vi "Labview_Mqtt_Toolkit.vi"() -> ()   [LabVIEW 2021]
uses:
  class/mqtt/mqttTypedef/mqttQOSlevel.ctl
  class/mqtt/mqttTypedef/mqttConnectionStatus.ctl
  class/mqtt/mqttTypedef/mqttBroker.ctl
  class/mqtt/mqttTXqueue/mqttTXdataQueueFunction.ctl
  class/mqtt/mqttConfigFunction.ctl
  class/mqtt/mqttTXqueue/mqttRXsubscriptionEventFunction.ctl
  class/mqtt/mqttTypedef/mqttConnectionFlags.ctl
  <vilib>/Utility/sysdir.llb/System Directory Type.ctl
  library/Epoch Date & Time/epoch.UNIX/Epoch.UNIX.lvclass
  C:/Users/Fujitsu/Desktop/Nouveau dossier/avril/Project mqtt/Src/library/Epoch Date & Time/epoch/Epoch.lvclass
  <vilib>/Utility/file.llb/Write Delimited Spreadsheet (string).vi
  library/Epoch Date & Time/Get Epoch Time.vi
  class/mqtt/mqtt.lvclass
panel:
  out "concatenated string":string
  in  "Tab Control":T1(tab)
  out "Connection Success":bool
  in  "connect":bool
  out "ConnStatus":T2
  in  "disconnect":bool
  in  "subscribe":bool
  out "Subscribe Success":bool
  out "subscribeMessageID":u16 format="%02x"
  in  "Subscription_Info":cluster{"Topic":string, "QoS":T3}[](array[cluster])=[{"Topic"="MacID/Topic", "QoS"=enum."At most once"}]
  out "Subscribed_Topic":string
  out "messageID":u16
  in  "quit":bool
  in  "Broker configuration":T4={"IP or  URL of the broker"="", "connTimeout"=2000, "writeTimeout"=2000, "readTimeout"=2000, "subTimeout"=30000, "port"=1883}
  out "Measure Graph":dbl(graph)
  out "Measure Mode":string
  out "Sensor Label":string
  out "Measure":dbl
  out "Date & time":string
  out "Device type":string
  out "End Date":string
  out "Start Date":string
  out "Average value":dbl
  out "Minimum value":dbl
  out "Maximum value":dbl
  out "Date":string
  out "Date":string
  out "File path":path
  out "File path":path
  out "Measure Mode":string
  out "Sensor Label":string
  out "Measure":dbl
  out "Date & time":string
  out "Device type":string
  out "Alarm status":string
  out "Waveform Chart":dbl(graph) caption="Measure Graph"
  out "File path 3":path
  out "Sampling rate":i16
  out "Frame sequence Id":u32
  out "Number of daq per channel":u16
  out "Data acquisition cycle":u32
  out "Data acquisition duration":u32
  out "Prev.Number of daq per channel":u16
  out "Enabled channels":string
  out "Device Type":string
  out "Measure Mode":string
  out "millisec":u16
  out "not synchronised":bool
  out "synchronised":bool
  out "Network Quality (LQI)":u8 format="%.0p"
  out "Time Ref":string
  out "INC_Y Graph":dbl[](graph)
  out "CH_Z Graph":dbl[](graph)
  out "CH_X Graph":dbl[](graph)
  out "CH_Y Graph":dbl[](graph)
  out "INC_X Graph":dbl[](graph)
  out "File path":path
  out "Enabled channels":string
  out "Device Type":string
  out "Measure Mode":string
  out "Frame sequence Id":u32
  out "Number of daq per channel":u16
  out "Data Notification cycle":u32
  out "Data acquisition duration":u32
  out "Prev.Number of daq per channel":u16
  out "not synchronised":bool
  out "synchronised":bool
  out "Network Quality (LQI)":u8 format="%.0p"
  out "Sampling rate":i16
  out "millisec":u16
  out "Time Ref":string
  out "channel that received alarm":u8
  out "CH_Z Graph":dbl[](graph)=[0.984, 0.974, 0.974, 0.986, 1.009, 0.965, 0.949, 0.987, 0.909, 0.979, 0.976, 1.021, 0.92, 0.95, 1.042, 0.989, 0.939, 1.09, 0.874, 0.972, 0.98, 0.977, 0.963, 0.971, 0.982, 0.977, 0.992, 0.993, 0.98, 0.969, 0.975, 0.969, 0.986, 0.985, 0.978, 0.977, 0.982, 0.979, 0.977, 0.972, 0.967, 0.968, 0.986, 0.97, 0.973, 0.977, 0.982, 0.973, 0.953, 0.969, 0.983, 0.968, 0.965, 0.975, 0.974, 0.972, 0.983, 0.99, 0.968, 0.972, 0.97, 0.981, 0.968, 0.982, 0.979, 0.972]
  out "CH_X Graph":dbl[](graph)=[0.011, 0.001, 0.002, 0.005, 0.007, 0.003, 0.001, 0.011, -0.001, 0.008, 0.006, 0.001, -0.001, 0.017, -0.002, 0.004, 0.0, -0.007, 0.002, -0.007, 0.001, 0.002, 0.0, 0.003, 0.004, 0.009, 0.004, 0.012, 0.003, 0.003, 0.004, 0.003, 0.006, 0.001, -0.001, 0.003, 0.002, 0.001, 0.003, 0.0, -0.001, 0.005, 0.0, 0.005, 0.001, 0.005, 0.005, -0.001, -0.002, -0.001, 0.005, 0.003, -0.003, -0.003, 0.002, -0.002, 0.002, 0.007, 0.0, 0.0, -0.002, 0.001, 0.002, 0.005, 0.011, 0.006]
  out "CH_Y Graph":dbl[](graph)=[-0.006, -0.012, -0.012, -0.009, -0.015, 0.009, 0.007, -0.013, 0.026, 0.009, -0.014, -0.014, 0.046, 0.055, -0.014, 0.004, 0.027, -0.027, 0.076, -0.008, -0.016, -0.026, -0.02, -0.015, -0.01, -0.002, -0.005, -0.011, -0.019, -0.019, -0.014, -0.009, -0.01, -0.01, -0.017, -0.015, -0.01, -0.013, -0.014, -0.014, -0.014, -0.014, -0.013, -0.017, -0.015, -0.013, -0.008, -0.015, -0.02, -0.017, -0.011, -0.014, -0.015, -0.016, -0.019, -0.016, -0.016, -0.012, -0.016, -0.016, -0.01, -0.013, -0.013, -0.019, -0.015, -0.012]
  out "INC_X Graph":dbl[](graph)=[0.03, 0.047, 0.036, 0.04, 0.082, 0.015, 0.021, 0.002, -0.032, 0.039, 0.026, 0.014, 0.037, 0.052, 0.099, 0.049, 0.039, 0.13, -0.382, 0.13, 0.113, 0.024, 0.006, -0.008, 0.051, 0.01, 0.082, 0.011, 0.03, 0.0, 0.031, 0.032, 0.033, 0.046, 0.032, 0.037, 0.018, 0.028, 0.024, 0.031, -0.008, 0.054, 0.011, 0.025, 0.04, 0.026, 0.022, 0.017, 0.028, 0.042, 0.024, 0.016, 0.034, 0.035, 0.018, 0.043, 0.014, 0.039, 0.033, 0.018, 0.035, 0.027, 0.041, 0.031, 0.035, 0.03]
  out "INC_Y Graph":dbl[](graph)=[0.458, 0.458, 0.458, 0.458, 0.458, 0.458, 0.458, 0.458, 0.458, 0.458, 0.458, 0.458, 0.458, 0.458, 0.458, 0.458, 0.458, 0.458, 0.458, 0.458, 0.458, 0.458, 0.458, 0.458, 0.458, 0.458, 0.458, 0.458, 0.458, 0.458, 0.458, 0.458, 0.458, 0.458, 0.458, 0.458, 0.458, 0.458, 0.458, 0.458, 0.458, 0.458, 0.458, 0.458, 0.458, 0.458, 0.458, 0.458, 0.458, 0.458, 0.458, 0.458, 0.458, 0.458, 0.458, 0.458, 0.458, 0.458, 0.458, 0.458, 0.458, 0.458, 0.458, 0.458, 0.458, 0.458]
  out "File path":path
  out "Device type":string
  out "Acquisition Mode":string
  out "Acquisition frequency":u16
  out "Acquisition cycle":u32
  out "Acquisition duration":u32
  out "Enabled channels":string
  out "Start date":string
  out "End date":string
  out "Number of data per channel":u16
  out "fid min ch1":u32
  out "index minval":u16
  out "fid max ch1":u32
  out "index maxval":u16
  out "Max value":dbl[](array[numeric])
  out "Average value":dbl[](array[numeric])
  out "Min value":dbl[](array[numeric])
  out "String":string="Ch_Z                    Ch_X                     Ch_Y                     INC_X                     INC_Y"
  out "File path":path
  out "Min date":string[](array[string])
  out "Max date":string[](array[string])
  out "Numeric":i32
  # "LowDutyCycle Measurement"
  # "MathMode Result"
  # "AlarmMode Data"
types:
  T1 = enum32{"Configuration", "LowDutyCycleData", "AlarmData ", "StreamingModeData", "S.E.T Mode", "Dynamic Math Result"}
  T2 = typedef "mqttConnectionStatus.ctl" = enum16{"Connection accepted", "Connection refused: unacceptable protocol version", "Connection refused: identifier rejected", "Connection refused: Server unavailable", "Connection refused: bad user name or password", "Connection refused: not authorized"}
  T3 = typedef "mqttQOSlevel.ctl" = enum8{"At most once", "At least once", "Exactly once", "Reserved"}
  T4 = typedef "mqttBroker.ctl" = cluster{"IP or  URL of the broker":string, "connTimeout":i32, "writeTimeout":i32, "readTimeout":i32, "subTimeout":i32, "port":u16}
  T5 = typedef "mqttConnectionFlags.ctl" = cluster{"reserved":bool, "clean session":bool, "will flag":bool, "willQOS":enum8{"At most once", "At least once", "Exactly once", "Reserved"}, "will retain":bool, "password":bool, "user name":bool}
  T6 = typedef "mqttRXsubscriptionEventFunction.ctl" = enum16{"init", "deinit", "getEventRef", "event"}
  T7 = typedef "mqtt.lvclass/mqttConfigFunction.ctl" = enum16{"init", "deinit", "set", "get"}
  T8 = typedef "mqttTXdataQueueFunction.ctl" = enum16{"init", "deinit", "getQueue", "enqueue"}
  T9 = enum8{"Enabled", "Disabled", "Disabled and Grayed Out"}
  T10 = enum16{"open", "replace", "create", "open or create", "replace or create", "replace or create with confirmation"}
  T11 = cluster{"[0]":u8, "[1]":u8, "[2]":u8, "[3]":u8, "[4]":u8, "[5]":u8, "[6]":u8, "[7]":u8, "[8]":u8}
  T12 = cluster{"[0]":u8, "[1]":u8, "[2]":u8, "[3]":u8, "[4]":u8, "[5]":u8, "[6]":u8, "[7]":u8, "[8]":u8, "[9]":u8, "[10]":u8, "[11]":u8, "[12]":u8}
  T13 = typedef "System Directory Type.ctl" = i32
  T14 = cluster{"unsigned byte array[0]":u8, "unsigned byte array[1]":u8}
  T15 = cluster{"[0]":u8, "[1]":u8, "[2]":u8, "[3]":u8, "[4]":u8, "[5]":u8, "[6]":u8, "[7]":u8, "[8]":u8, "[9]":u8, "[10]":u8, "[11]":u8, "[12]":u8, "[13]":u8, "[14]":u8, "[15]":u8}
  T16 = cluster{"unsigned byte array[0]":u8, "unsigned byte array[1]":u8, "unsigned byte array[2]":u8, "unsigned byte array[3]":u8, "unsigned byte array[4]":u8, "unsigned byte array[5]":u8, "unsigned byte array[6]":u8, "unsigned byte array[7]":u8, "unsigned byte array[8]":u8, "unsigned byte array[9]":u8, "unsigned byte array[10]":u8, "unsigned byte array[11]":u8, "unsigned byte array[12]":u8, "unsigned byte array[13]":u8, "unsigned byte array[14]":u8, "unsigned byte array[15]":u8, "unsigned byte array[16]":u8, "unsigned byte array[17]":u8, "unsigned byte array[18]":u8, "unsigned byte array[19]":u8, "unsigned byte array[20]":u8, "unsigned byte array[21]":u8, "unsigned byte array[22]":u8, "unsigned byte array[23]":u8, "unsigned byte array[24]":u8, "unsigned byte array[25]":u8, "unsigned byte array[26]":u8, "unsigned byte array[27]":u8, "unsigned byte array[28]":u8, "unsigned byte array[29]":u8, "unsigned byte array[30]":u8, "unsigned byte array[31]":u8, "unsigned byte array[32]":u8, "unsigned byte array[33]":u8, "unsigned byte array[34]":u8, "unsigned byte array[35]":u8}
  T17 = cluster{"[0]":string, "[1]":string, "[2]":string, "[3]":string, "[4]":string}
  T18 = cluster{"[0]":dbl, "[1]":dbl, "[2]":dbl, "[3]":dbl, "[4]":dbl}
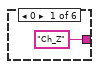
[diagram p7: hidden frame]
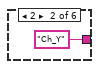
[diagram p8: hidden frame]
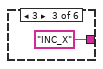
[diagram p9: hidden frame]
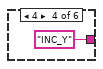
[diagram p10: hidden frame]
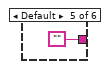
[diagram p11: hidden frame]
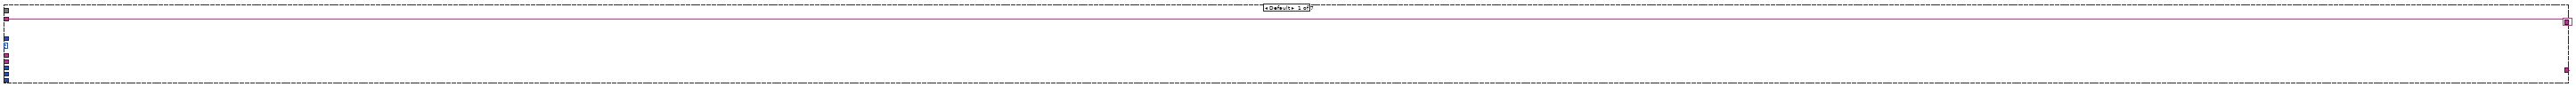
[diagram p12: hidden frame]
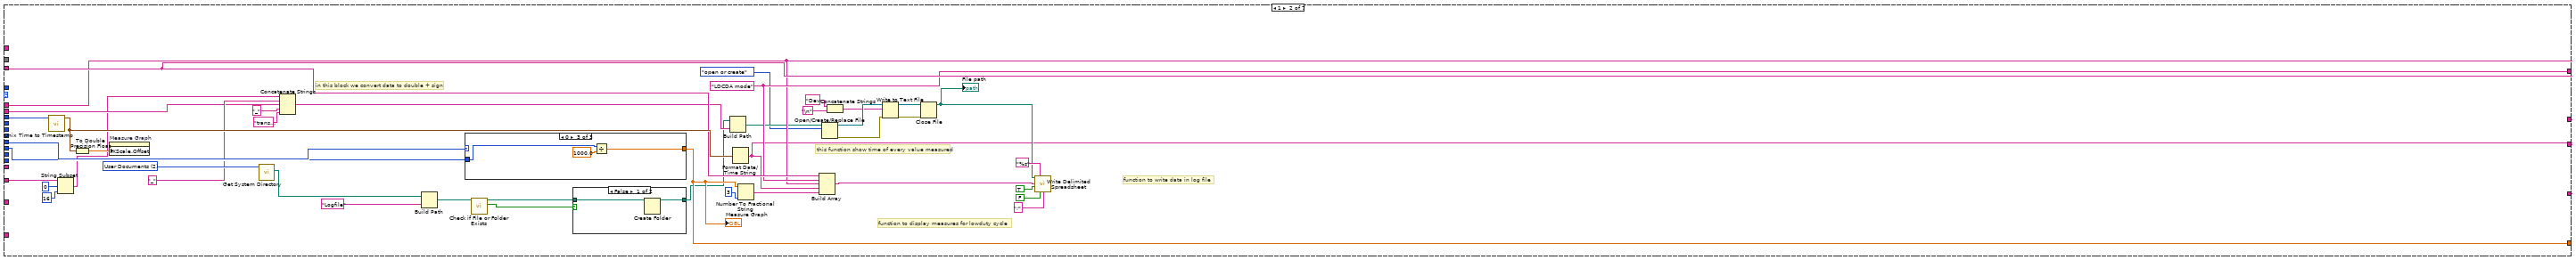
[diagram p13: hidden frame]
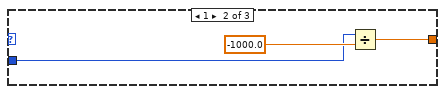
[diagram p16: hidden frame]
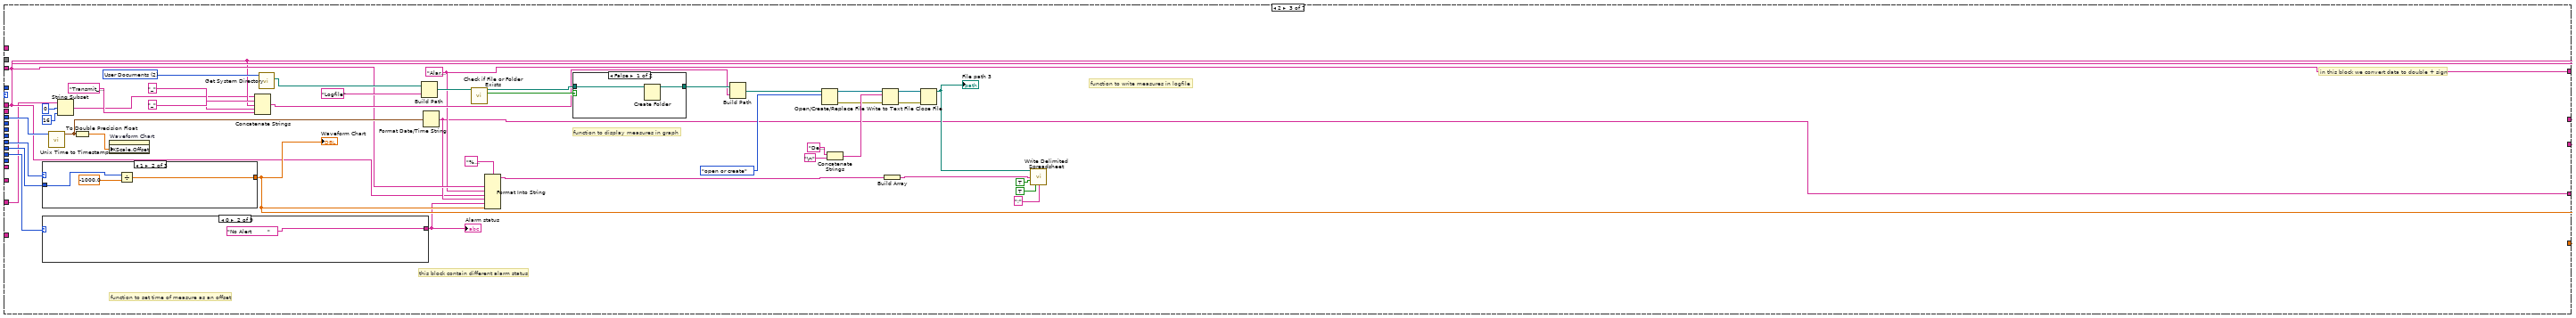
[diagram p17: hidden frame]
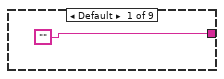
[diagram p18: hidden frame]
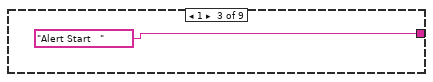
[diagram p19: hidden frame]
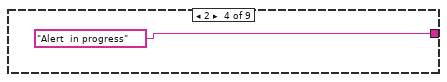
[diagram p20: hidden frame]
diagram:
  w6 = T5 {"reserved"=FALSE, "clean session"=TRUE, "will flag"=TRUE, "willQOS"=enum."At most once", "will retain"=FALSE, "password"=FALSE, "user name"=FALSE}  # connFlags
  # "used to reinitialize to default  data when you execute VI"
  # "cluster contain connection flags"
  # "cluster contain broker configuration"
  # "you will find the subscriptionData in event number 4 by click on this arrow"
  n1 = flat-sequence {
    tunnel: [w25] -> w19
    tunnel: [w22] -> w13
    frame #0 {
      w21 = T9."Disabled and Grayed Out" ("Disabled")
      n2 = property on="disconnect" class="Bool"("DisabledEnum"=w21) -> ()  [unwired: 2 in, 2 out]
      n3 = property on="subscribe" class="Bool"("DisabledEnum"=w21) -> ()  [unwired: 2 in, 2 out]
      n4 = call "mqttRXsubscriptionEvent.vi"("function"=mqttRXsubscriptionEventFunction."init") -> ("subscriptionData"=w22:refnum<user-event>, "error out"=w24:errorcluster)  [unwired: 13 in]
      n5 = call "mqttTXdataQueue.vi"("function"=mqttTXdataQueueFunction."init", "error in (no error)"=w24) -> ("error out"=w25:errorcluster)  [unwired: 12 in, 1 out]
    }
  }
  n6 = control-ref of="This VI"() -> (w5:refnum<vi>)
  n7 = invoke class="VI" method="Default Vals.Reinit All"(reference=w5) -> (reference out=w3:refnum<vi>, error out=w4:errorcluster)  [unwired: 2 in, 1 out]
  n8 = call "api_mqttInit.vi"("broker"="Broker configuration", "connFlags"=w6, "error in (no error)"=w19) -> ("error out"=w17:errorcluster)  [unwired: 12 in]
  n9 = register-events(w13) -> (reference out=w12:refnum<event-registration>)  [unwired: 2 in, 1 out]
  n10 = call "mqttConfigStore.vi"("function"=mqttConfigFunction."get", "error in (no error)"=w17) -> ("mqtt.lvclass out"=w16:refnum<class "mqtt.lvclass">, "error out"=w15:errorcluster)  [unwired: 12 in]
  n11 = call "mqttTCPIPserver.vi"("mqtt.lvclass"=w16, "error in (no error)"=w15) -> ()  [unwired: 12 in, 2 out]
  n12 = Close Reference(reference=w3, error in (no error)=w4) -> (error out=w2:errorcluster)
  n13 = while {
    shift-right: [w32] -> w9
    shift-left: w15 -> [w27]
    tunnel: w12 -> [w31]
    tunnel: [w30] -> w7
    tunnel: w2 -> [_]
    i -> [w28]
    stop <- w29 stop-if-true
    n14 = event shown="[4] <subscriptionData>: User Event" {
      selector: w31 -> [_ _ _ _ _]
      dyn-events: [_ _ _ _ _] -> w30
      timeout: _ -> [_ _ _ _ _]
      tunnel: [w33 w37 w40 w44 w129] -> w32
      tunnel: w27 -> [w33 w38 w41 w42 w129]
      tunnel: [TRUE _ _ _ _] -> w29
      tunnel: w28 -> [_ _ _ _ w50]
      event "quit": Value Change {
        # "when we press quit in front panel the process is stopped"
        n15 = event-data() -> ()  [unwired: 1 in, 1 out]
      }
      event "connect": Value Change {
        n16 = event-data() -> ()  [unwired: 1 in, 4 out]
        n17 = call "api_mqttConnect.vi"("error in (no error)"=w38) -> ("success"=→"Connection Success":bool, "connStatus"=w36:T2, "error out"=w37:errorcluster)  [unwired: 11 in, 1 out]
        "ConnStatus" <- w36
        n18 = case shown="\"Connection accepted\"" w36 {
          frame "Connection accepted" {
            w39 = T9."Enabled" ("Disabled")
            n19 = property on="subscribe" class="Bool"("DisabledEnum"=w39) -> ()  [unwired: 2 in, 2 out]
            n20 = property on="disconnect" class="Bool"("DisabledEnum"=w39) -> ()  [unwired: 2 in, 2 out]
          }
          frame Default {
          }
        }
      }
      event "disconnect": Value Change {
        n21 = event-data() -> ()  [unwired: 1 in, 4 out]
        n22 = call "api_mqttDisconnect.vi"("error in (no error)"=w41) -> ("error out"=w40:errorcluster)  [unwired: 13 in, 1 out]
      }
      event "subscribe": Value Change {
        # "this indicator turn to green when the subscription sucssed"
        n23 = event-data() -> ()  [unwired: 1 in, 4 out]
        n24 = feedback #1(u16 0) -> (w47:u16)
        n25 = Increment(x=w47) -> (x+1=w43:u16)
        "subscribeMessageID" <- w43
        n26 = feedback-in #1(w43) -> ()
        n27 = call "api_mqttSubscribe.vi"("subscriptionInfo"="Subscription_Info", "messageID"=w43, "error in (no error)"=w42) -> ("success"=→"Subscribe Success":bool, "error out"=w44:errorcluster)  [unwired: 11 in]
      }
      event User Event {
        # "here you will find different modes of  data acquisition"
        n28 = event-data() -> ("topic"=w49:string, "value"=w63:string, "messageID"=→"messageID":u16)  [unwired: 1 in]
        "Subscribed_Topic" <- w49
        n29 = String To Byte Array(string=w63) -> (unsigned byte array=w71:u8[])
        n30 = Reverse 1D Array(array=w71) -> (reversed array=w115:u8[])
        n31 = Array Subset(array=w115, index=0, length=3) -> (w54:u8[])
        n32 = Array Subset(array=w71, index=0, length=7) -> (w66:u8[])
        n33 = Array Subset(array=w71, index=7, length=1) -> (w73:u8[])
        n34 = Array To Cluster(array=w73) -> (cluster=w72:cluster{"[0]":u8})
        n35 = Array To Cluster(array=w66) -> (cluster=w121:T11)
        n36 = Array Subset(array=w71, index=3, length=13) -> (w108:u8[])
        n37 = Unbundle By Name(w72) -> ("[0]"=w52:u8)
        n38 = Unbundle By Name(w121) -> ("[0]"=w53:u8, "[1]"=w79:u8, "[2]"=w116:u8, "[3]"=w120:u8, "[4]"=w119:u8, "[5]"=w118:u8, "[6]"=w117:u8)
        n39 = Array To Cluster(array=w108) -> (cluster=w107:T12)
        n40 = Array To Cluster(array=w54) -> (cluster=w61:cluster{"[0]":u8, "[1]":u8, "[2]":u8})
        n41 = Unbundle By Name(w107) -> ("[0]"=w64:u8, "[1]"=w87:u8, "[2]"=w86:u8, "[3]"=w85:u8, "[4]"=w84:u8, "[5]"=w91:u8, "[6]"=w90:u8, "[7]"=w89:u8, "[8]"=w88:u8, "[9]"=w81:u8, "[10]"=w80:u8, "[11]"=w83:u8, "[12]"=w82:u8)
        n42 = Join Numbers(hi=w117, lo=w118) -> ((hi.lo)=w112:u16)
        n43 = Join Numbers(hi=w119, lo=w120) -> ((hi.lo)=w111:u16)
        n44 = Unbundle(w61) -> ("[0]"=w58:u8, "[1]"=w59:u8, "[2]"=w60:u8)
        n45 = case shown="6" w53 {
          tunnel: ["AX-3D" "HI_INC_MONO" "HI_INC_BI" "X_INC_MONO " "X _INC_BI " "AX_3DS" ""] -> w62
          frame 1 {
          }
          frame 2 {
          }
          frame 3 {
          }
          frame 4 {
          }
          frame 5 {
          }
          frame 6 {
          }
          frame Default {
          }
        }
        "Device type" <- w62
        n46 = case shown="1" w116 {
          tunnel: ["Ch_Z" "Ch_Y" "INC_X" "INC_Y" "" "Ch_X"] -> w51
          frame 0 {
          }
          frame 2 {
          }
          frame 3 {
          }
          frame 4 {
          }
          frame Default {
          }
          frame 1 {
          }
        }
        n47 = Join Numbers(hi=w59, lo=w60) -> ((hi.lo)=w56:u16)
        n48 = Join Numbers(hi=w84, lo=w85) -> ((hi.lo)=w103:u16)
        n49 = Join Numbers(hi=w86, lo=w87) -> ((hi.lo)=w102:u16)
        n50 = Join Numbers(hi=w88, lo=w89) -> ((hi.lo)=w98:u16)
        n51 = Join Numbers(hi=w90, lo=w91) -> ((hi.lo)=w97:u16)
        n52 = Join Numbers(hi=w82, lo=w83) -> ((hi.lo)=w93:u16)
        n53 = Join Numbers(hi=w80, lo=w81) -> ((hi.lo)=w92:u16)
        n54 = To Unsigned Word Integer(number=w112) -> (unsigned 16bit integer=w125:u16)
        n55 = To Unsigned Word Integer(number=w111) -> (unsigned 16bit integer=w124:u16)
        n56 = To Word Integer(number=w58) -> (16bit integer=w127:i16)
        n57 = Sign(1:w127) -> (0:w57:i16)
        n58 = Join Numbers(hi=w125, lo=w124) -> ((hi.lo)=w126:u32)
        n59 = To Unsigned Word Integer(number=w103) -> (unsigned 16bit integer=w105:u16)
        n60 = To Unsigned Word Integer(number=w102) -> (unsigned 16bit integer=w104:u16)
        n61 = To Unsigned Word Integer(number=w98) -> (unsigned 16bit integer=w100:u16)
        n62 = To Unsigned Word Integer(number=w97) -> (unsigned 16bit integer=w99:u16)
        n63 = To Unsigned Word Integer(number=w93) -> (unsigned 16bit integer=w95:u16)
        n64 = To Unsigned Word Integer(number=w92) -> (unsigned 16bit integer=w94:u16)
        n65 = Join Numbers(hi=w105, lo=w104) -> ((hi.lo)=w106:u32)
        n66 = Join Numbers(hi=w100, lo=w99) -> ((hi.lo)=w101:u32)
        n67 = Join Numbers(hi=w95, lo=w94) -> ((hi.lo)=w96:u32)
        n68 = To Unsigned Long Integer(number=w126) -> (unsigned 32bit integer=w78:u32)
        n69 = To Unsigned Long Integer(number=w106) -> (unsigned 32bit integer=w75:u32)
        n70 = To Unsigned Long Integer(number=w101) -> (unsigned 32bit integer=w76:u32)
        n71 = To Unsigned Long Integer(number=w96) -> (unsigned 32bit integer=w77:u32)
        n72 = case shown="3" w79 {
          tunnel: ["" w172 w206 "Streaming mode" "LDC Math Result" "S.E.T mode " "Dynamic Math Result"] -> w70
          tunnel: w78 -> [_ w178 w232 _ _ _ _]
          tunnel: [_ w146 w198 _ "" _ _] -> w65
          tunnel: w62 -> [w136 w174 w207 w406 w2481 w2648 w4843]
          tunnel: [w136 w174 w207 w406 w2481 w2648 w4843] -> w69
          tunnel: w51 -> [_ w171 w196 w405 w2479 _ w4842]
          tunnel: [_ w171 w196 w405 w2479 _ w4842] -> w68
          tunnel: w57 -> [_ w180 w230 _ w2475 _ _]
          tunnel: w56 -> [_ w179 w231 _ w2477 _ _]
          tunnel: [_ w175 w205 _ _ _ _] -> w55
          tunnel: w64 -> [_ _ _ _ w2476 _ _]
          tunnel: w77 -> [_ _ _ _ w2478 _ _]
          tunnel: w76 -> [_ _ _ _ w2433 _ _]
          tunnel: w75 -> [_ _ _ _ w2434 _ _]
          tunnel: w63 -> [_ _ _ w352 _ w2637 w4840]
          tunnel: w62 -> [_ _ _ _ _ _ w4841]
          tunnel: w54 -> [_ _ _ _ _ _ _]
          tunnel: w49 -> [_ _ _ w255 w2439 _ _]
          tunnel: w49 -> [_ _ w191 _ _ w2503 w4683]
          tunnel: w49 -> [_ w141 _ _ _ _ _]
          tunnel: w53 -> [_ _ _ _ _ _ w4721]
          tunnel: w52 -> [_ _ w200 _ _ _ _]
          tunnel: w51 -> [_ w144 _ _ w2444 _ _]
          frame Default {
          }
          frame 1 {
            w152 = T13 2 items=["User Home"=0, "User Desktop"=1, "User Documents"=2, "User Application Data"=3, "User Preferences"=4, "User Temporary"=5, "Public Documents"=6, "Public Application Data"=7, "Public Preferences"=8, "Public Cache"=13, "System Core Libraries"=9, "System Installed Libraries"=10, "Application Files"=11, "Boot Volume Root"=12] ("system directory type")
            w172 = "LDCDA mode"
            # "this function show time of every value measured"
            # "function to display measures for lowduty cycle"
            # "function to write data in log file"
            # "in this block we convert data to double + sign"
            n73 = call "Unix Time to Timestamp.vi"("Unix Time (s)"=w178) -> ("Timestamp"=w177:timestamp)  [unwired: 9 in, 1 out]
            n74 = String Subset(string=w141, offset (0)=0, length (rest)=16 ("length (rest)")) -> (substring=w138:string)
            n75 = To Double Precision Float(number=w177) -> (double precision float=w165:dbl)
            n76 = property on="Measure Graph" class="WFChart (strict)"("XScale.Offset"=w165) -> ()  [unwired: 2 in, 2 out]
            n77 = call <vilib>:"Get System Directory.vi"("system directory type"=w152) -> ("system directory"=w158:path)  [unwired: 10 in]
            n78 = Concatenate Strings(w138, "_" ("string"), w144, "_" ("string"), "transmit_LowDutyCycle.csv") -> (w164:string)
            n79 = Build Path(base path=w158, name or relative path="Logfile") -> (appended path=w159:path)
            n80 = case shown="0" w180 {
              tunnel: [_ w185 w188] -> w175
              tunnel: w179 -> [_ w184 w187]
              frame Default {
              }
              frame 1 {
                n81 = Divide(x=w184, y=-1000.0) -> (x/y=w185:dbl)
              }
              frame 0 {
                n82 = Divide(x=w187, y=1000.0) -> (x/y=w188:dbl)
              }
            }
            "Measure Graph" <- w175
            n83 = call <vilib>:"Check if File or Folder Exists.vi"("path"=w159) -> ("file or folder exists?"=w160:bool, "dup path"=w161:path)  [unwired: 8 in, 1 out]
            n84 = case shown="False" w160 {
              tunnel: w161 -> [w182 w183]
              tunnel: [w181 w183] -> w162
              frame False {
                n85 = Create Folder(path (use dialog)=w182) -> (created path=w181:path)  [unwired: 2 in, 2 out]
              }
              frame True {
              }
            }
            n86 = Build Path(base path=w162, name or relative path=w164) -> (appended path=w163:path)
            n87 = Format Date/Time String(seconds (now)=w177) -> (date/time string=w146:string)  [unwired: 2 in]
            n88 = Number To Fractional String(number=w175, precision (6)=i16 3) -> (F-format string=w173:string)  [unwired: 2 in]
            n89 = Build Array(w174, w172, w171, w146, w173) -> (w167:string[])
            n90 = Open/Create/Replace File(file path (use dialog)=w163, operation (0:open)=T10."open or create") -> (refnum out=w154:refnum<file>, error out=w156:errorcluster)  [unwired: 4 in, 1 out]
            n91 = Concatenate Strings("Device Type ;Measure mode;Sensor label;date & time;Measure  ", "\n") -> (w153:string)
            n92 = Write to Text File(file (use dialog)=w154, text=w153, error in=w156) -> (refnum out=w155:refnum<file>, error out=w157:errorcluster)  [unwired: 1 in, 1 out]
            n93 = Close File(refnum=w155, error in=w157) -> (path=w147:path)  [unwired: 1 out]
            "File path" <- w147
            n94 = call-poly <vilib>:"Write Delimited Spreadsheet.vi"("file path (dialog if empty)"=w147, "format (%s)"="%s" ("format (%.3f)"), "1D data"=w167, "append to file? (new file:F)"=TRUE, "transpose? (no:F)"=FALSE, "delimiter (\\t)"=";" ("delimiter (\\t)")) -> ()  [unwired: 8 in, 2 out]
          }
          frame 2 {
            w215 = T13 2 items=["User Home"=0, "User Desktop"=1, "User Documents"=2, "User Application Data"=3, "User Preferences"=4, "User Temporary"=5, "Public Documents"=6, "Public Application Data"=7, "Public Preferences"=8, "Public Cache"=13, "System Core Libraries"=9, "System Installed Libraries"=10, "Application Files"=11, "Boot Volume Root"=12] ("system directory type")
            w206 = "Alarm mode"
            # "function to write measures in logfile"
            # "function to set time of measure as an offset"
            # "function to display measures in graph"
            # "this block contain different alarm status"
            # "in this block we convert data to double + sign"
            n95 = case shown="1" w230 {
              tunnel: [_ w246 w249] -> w205
              tunnel: w231 -> [_ w245 w248]
              frame Default {
              }
              frame 1 {
                n96 = Divide(x=w245, y=-1000.0) -> (x/y=w246:dbl)
              }
              frame 0 {
                n97 = Divide(x=w248, y=1000.0) -> (x/y=w249:dbl)
              }
            }
            "Waveform Chart" <- w205
            n98 = case shown="0" w200 {
              tunnel: ["" "No Alert         " "Alert Start   " "Alert  in progress" "Alert  End   " "Action Start" "Action in Progress" "Alarm Start" "Alarm Progress"] -> w199
              frame Default {
              }
              frame 0 {
              }
              frame 1 {
              }
              frame 2 {
              }
              frame 3 {
              }
              frame 4 {
              }
              frame 5 {
              }
              frame 6 {
              }
              frame 7 {
              }
            }
            "Alarm status" <- w199
            n99 = call "Unix Time to Timestamp.vi"("Unix Time (s)"=w232) -> ("Timestamp"=w229:timestamp)  [unwired: 9 in, 1 out]
            n100 = String Subset(string=w191, offset (0)=0, length (rest)=16 ("length (rest)")) -> (substring=w190:string)
            n101 = To Double Precision Float(number=w229) -> (double precision float=w225:dbl)
            n102 = property on="Waveform Chart" class="WFChart (strict)"("XScale.Offset"=w225) -> ()  [unwired: 2 in, 2 out]
            n103 = Concatenate Strings(w190, "_" ("string"), w196, "_" ("string"), "Transmit_AlarmMode.csv") -> (w208:string)
            n104 = call <vilib>:"Get System Directory.vi"("system directory type"=w215) -> ("system directory"=w216:path)  [unwired: 10 in]
            n105 = Build Path(base path=w216, name or relative path="Logfile") -> (appended path=w213:path)
            n106 = Format Date/Time String(seconds (now)=w229) -> (date/time string=w198:string)  [unwired: 2 in]
            n107 = call <vilib>:"Check if File or Folder Exists.vi"("path"=w213) -> ("file or folder exists?"=w212:bool, "dup path"=w211:path)  [unwired: 8 in, 1 out]
            n108 = Format Into String(format string="%s;%s;%s;%s;%s;%.3f", w207, w206, w196, w198, w199, w205) -> (resulting string=w201:string)  [unwired: 2 in, 1 out]
            n109 = case shown="False" w212 {
              tunnel: w211 -> [w243 w244]
              tunnel: [w242 w244] -> w210
              frame False {
                n110 = Create Folder(path (use dialog)=w243) -> (created path=w242:path)  [unwired: 2 in, 2 out]
              }
              frame True {
              }
            }
            n111 = Build Path(base path=w210, name or relative path=w208) -> (appended path=w209:path)
            n112 = Open/Create/Replace File(file path (use dialog)=w209, operation (0:open)=T10."open or create") -> (refnum out=w223:refnum<file>, error out=w221:errorcluster)  [unwired: 4 in, 1 out]
            n113 = Concatenate Strings("Device Type ;Measure mode;Sensor label;date & time;Alarm status ;Measure  ", "\n") -> (w224:string)
            n114 = Write to Text File(file (use dialog)=w223, text=w224, error in=w221) -> (refnum out=w222:refnum<file>, error out=w220:errorcluster)  [unwired: 1 in, 1 out]
            n115 = Build Array(w201) -> (w203:string[])
            n116 = Close File(refnum=w222, error in=w220) -> (path=w202:path)  [unwired: 1 out]
            "File path 3" <- w202
            n117 = call-poly <vilib>:"Write Delimited Spreadsheet.vi"("file path (dialog if empty)"=w202, "1D data"=w203, "append to file? (new file:F)"=TRUE, "transpose? (no:F)"=TRUE, "delimiter (\\t)"=";") -> ()  [unwired: 9 in, 2 out]
          }
          frame 3 {
            # "this block contain measures+ time stamp which saved in the logfile"
            # "this block contain measured values"
            # "this block contain different device type"
            # "function towrite headers of the logfile"
            # "this block contain different types of streaming mode"
            # "function to calculate timestamp"
            n118 = String To Byte Array(string=w352) -> (unsigned byte array=w362:u8[])
            n119 = Array Size(array=w362) -> (size(s)=w363:i32)
            n120 = Array To Cluster(array=w362) -> (cluster=w371:T14)
            n121 = Array Subset(array=w362, index=2, length=8) -> (w402:u8[])
            n122 = Array Subset(array=w362, index=10, length=4) -> (w398:u8[])
            n123 = Array Subset(array=w362, index=14, length=15) -> (w393:u8[])
            n124 = Unbundle(w371) -> ("unsigned byte array[0]"=w329:u8, "unsigned byte array[1]"=w370:u8)
            n125 = Array To Cluster(array=w398) -> (cluster=w397:T11)
            n126 = Array To Cluster(array=w393) -> (cluster=w392:T15)
            n127 = Array To Cluster(array=w402) -> (cluster=w401:T11)
            n128 = Subtract(x=w363, y=29) -> (x-y=w358:i32)
            n129 = Unbundle By Name(w392) -> ("[0]"=w391:u8, "[1]"=w253:u8, "[2]"=w390:u8, "[3]"=w387:u8, "[4]"=w386:u8, "[5]"=w384:u8, "[6]"=w383:u8, "[7]"=w382:u8, "[8]"=w379:u8, "[9]"=w378:u8, "[10]"=w377:u8, "[11]"=w374:u8, "[12]"=w373:u8, "[13]"=w367:u8, "[14]"=→"Network Quality (LQI)":u8)
            n130 = Unbundle By Name(w397) -> ("[0]"=w396:u8)
            n131 = Unbundle By Name(w401) -> ("[0]"=w343:u8, "[1]"=w344:u8, "[2]"=w347:u8, "[3]"=w348:u8, "[4]"=w341:u8, "[5]"=w342:u8, "[6]"=w350:u8, "[7]"=w349:u8)
            n132 = Join Numbers(hi=w373, lo=w374) -> ((hi.lo)=w372:u16)
            n133 = To Unsigned Byte Integer(number=w396) -> (unsigned 8bit integer=w310:u8)
            n134 = Join Numbers(hi=w378, lo=w379) -> ((hi.lo)=w376:u16)
            n135 = Join Numbers(hi=w383, lo=w384) -> ((hi.lo)=w381:u16)
            n136 = Join Numbers "time"(hi=w344, lo=w343) -> ((hi.lo)=w340:u16)
            n137 = Join Numbers "date"(hi=w348, lo=w347) -> ((hi.lo)=w346:u16)
            n138 = Join Numbers(hi=w349, lo=w350) -> ((hi.lo)=w351:u16)
            n139 = Array Subset(array=w362, index=29, length=w358) -> (w360:u8[])
            n140 = To Word Integer(number=w372) -> (16bit integer=→"Prev.Number of daq per channel":i16)
            n141 = Join Numbers(hi=w342, lo=w341) -> ((hi.lo)=w333:u16)
            "millisec" <- w333
            n142 = To Word Integer(number=w351) -> (16bit integer=w277:i16)
            "Sampling rate" <- w277
            n143 = Join Numbers(hi=w382, lo=w381) -> ((hi.lo)=w380:u32)
            n144 = To Unsigned Word Integer(number=w346) -> (unsigned 16bit integer=w306:u16)
            n145 = Join Numbers(hi=w377, lo=w376) -> ((hi.lo)=w375:u32)
            n146 = To Long Integer(number=w380) -> (32bit integer=w275:i32)
            "Data acquisition cycle" <- w275
            n147 = To Long Integer(number=w375) -> (32bit integer=w276:i32)
            "Data acquisition duration" <- w276
            n148 = Join Numbers(hi=w386, lo=w387) -> ((hi.lo)=w385:u16)
            n149 = Join Numbers(hi=w253, lo=w391) -> ((hi.lo)=w389:u16)
            n150 = Equal To 0?(x=w367) -> (x = 0?=→"not synchronised":bool)
            n151 = Decimate 1D Array(w360) -> (w353:u8[], w359:u8[], w357:u8[])
            n152 = Not Equal To 0?(x=w367) -> (x != 0?=→"synchronised":bool)
            n153 = Join Numbers(hi=w359, lo=w353) -> ((hi.lo)=w356:u16[])
            n154 = Join Numbers(hi=w390, lo=w389) -> ((hi.lo)=w388:u32)
            n155 = To Double Precision Float(number=w277) -> (double precision float=w304:dbl)
            n156 = To Word Integer(number=w385) -> (16bit integer=w354:i16)
            "Number of daq per channel" <- w354
            n157 = Divide(x=w333, y=i16 1000) -> (x/y=w334:dbl)
            n158 = To Long Integer(number=w388) -> (32bit integer=w355:i32)
            "Frame sequence Id" <- w355
            n159 = To Unsigned Word Integer(number=w334) -> (unsigned 16bit integer=w338:u16)
            n160 = Add(x=w340, y=w338) -> (x+y=w307:u16)
            n161 = Join Numbers(hi=w306, lo=w307) -> ((hi.lo)=w345:u32)
            n162 = To Unsigned Quad Integer(1:w345) -> (0:w339:u64)
            n163 = Multiply(x=w354, y=w355) -> (x*y=w327:i32)
            n164 = To Unsigned Quad Integer(1:w327) -> (0:w326:u64)
            n165 = for {
              tunnel: w357 -> [w2391] mode=indexing
              tunnel: [w2389] -> w308 mode=indexing
              tunnel: w356 -> [w2387] mode=indexing
              n166 = To Word Integer(number=w2391) -> (16bit integer=w2388:i16)
              n167 = Sign(1:w2388) -> (0:w2390:i16)
              n168 = case shown="1" w2390 {
                tunnel: [_ w2393 w2396] -> w2389
                tunnel: w2387 -> [_ w2392 w2395]
                frame Default {
                }
                frame 1 {
                  n169 = Divide(x=w2392, y=-1000.0) -> (x/y=w2393:dbl)
                }
                frame 0 {
                  n170 = Divide(x=w2395, y=1000.0) -> (x/y=w2396:dbl)
                }
              }
            }
            n171 = case shown="3" w370 {
              tunnel: ["" "LDCDA mode" "Alarm mode" "Streaming mode" "Shock Detection mode" "LDC Math Result" "SET mode " "Dynamic Math Result"] -> w303
              tunnel: w276 -> [_ _ _ w2406 _ _ _ _]
              tunnel: w275 -> [_ _ _ w2418 _ _ _ _]
              tunnel: [w2398 _ _ w2409 _ _ _ _] -> w301
              tunnel: [w2398 _ _ w2403 _ _ _ _] -> w300
              tunnel: [w2398 _ _ w2402 _ _ _ _] -> w299
              frame Default {
                w2398 = ""
              }
              frame 1 {
              }
              frame 2 {
              }
              frame 3 {
                n172 = Equal To 0?(x=w2418) -> (x = 0?=w2420:bool)
                n173 = Greater Than 0?(x=w2418) -> (x > 0?=w2404:bool)
                n174 = Equal To 0?(x=w2418) -> (x = 0?=w2416:bool)
                n175 = Equal To 0?(x=w2406) -> (x = 0?=w2417:bool)
                n176 = Greater Than 0?(x=w2406) -> (x > 0?=w2405:bool)
                n177 = And(x=w2420, y=w2405) -> (x .and. y?=w2414:bool)
                n178 = And(x=w2405, y=w2404) -> (x .and. y?=w2413:bool)
                n179 = And(x=w2417, y=w2416) -> (x .and. y?=w2415:bool)
                n180 = Select(t="burst", s=w2413, f="") -> (s? t:f=w2403:string)
                n181 = Select(t="one shot", s=w2414, f="") -> (s? t:f=w2409:string)
                n182 = Select(t="continuous monitoring", s=w2415, f="") -> (s? t:f=w2402:string)
              }
              frame 4 {
              }
              frame 5 {
              }
              frame 6 {
              }
              frame 7 {
              }
            }
            n183 = call "Unix Time to Timestamp.vi"("Fractional Second"=w334, "Unix Time (s)"=w339) -> ("Timestamp"=w336:timestamp)  [unwired: 8 in, 1 out]
            n184 = Increment(x=w326) -> (x+1=w330:u64)
            n185 = for {
              N: w330 -> [_]
              tunnel: w326 -> [w2386]
              tunnel: [w2386] -> w332
            }
            n186 = Format Date/Time String(time format string (%c)="%x %X %3u", seconds (now)=w336) -> (date/time string=w269:string)  [unwired: 1 in]
            "Time Ref" <- w269
            n187 = Decrement(x=w332) -> (x-1=w331:u64)
            n188 = for {
              tunnel: w308 -> [w2385] mode=indexing
              shift-right: [w2383] -> _
              shift-left: w331 -> [w2384]
              tunnel: [w2382] -> w328 mode=indexing
              tunnel: [w2385] -> _ mode=indexing
              n189 = Increment(x=w2384) -> (x+1=w2383:u64)
              n190 = To Unsigned Quad Integer(1:w2383) -> (0:w2382:u64)
            }
            n191 = Search and Replace String(replace all?=TRUE ("replace all? (F)"), input string=w269, search string=":", replace string="_") -> (result string=w290:string)  [unwired: 4 in, 3 out]
            n192 = Search and Replace String(replace all?=TRUE ("replace all? (F)"), input string=w290, search string=",", replace string="_") -> (result string=w289:string)  [unwired: 4 in, 3 out]
            n193 = To Unsigned Quad Integer(1:w328) -> (0:w305:u64[])
            n194 = case shown="6" w329 {
              tunnel: ["AX-3D" "HI_INC_MONO" "HI_INC_BI" "X_INC_MONO " "X _INC_BI " "AX_3DS" ""] -> w251
              frame 1 {
              }
              frame 2 {
              }
              frame 3 {
              }
              frame 4 {
              }
              frame 5 {
              }
              frame 6 {
              }
              frame Default {
              }
            }
            "Device Type" <- w251
            n195 = call <vilib>:"Space Constant.vi"() -> ("String"=w302:string)
            n196 = Concatenate Strings(w303, w302, w301, w300, w299) -> (w252:string)
            "Measure Mode" <- w252
            "concatenated string" <- w252
            n197 = Number To Decimal String(number=w277) -> (decimal integer string=w266:string)  [unwired: 1 in]
            n198 = Number To Decimal String(number=w275) -> (decimal integer string=w263:string)  [unwired: 1 in]
            n199 = Number To Decimal String(number=w276) -> (decimal integer string=w260:string)  [unwired: 1 in]
            n200 = Search and Replace String(replace all?=TRUE ("replace all? (F)"), input string=w289, search string="/", replace string="_") -> (result string=w285:string)  [unwired: 4 in, 3 out]
            n201 = String Subset(string=w285, offset (0)=0, length (rest)=20 ("length (rest)")) -> (substring=w282:string)
            n202 = Concatenate Strings("Device type :", w251, ";", "Measure Mode :", w252, ";", "Time reference :" ("string"), w269, ";", " Sampling rate :", w266, ";" ("string"), "Data acquisition cycle :" ("string"), w263, ";" ("string"), "Data acquisition duration :" ("string"), w260, ";" ("string"), "\n") -> (w279:string)
            n203 = String Subset(string=w255, offset (0)=0, length (rest)=16 ("length (rest)")) -> (substring=w254:string)
            n204 = call <vilib>:"Space Constant.vi"() -> ("String"=w281:string)
            n205 = Build Array(w279) -> (w274:string[])
            n206 = Concatenate Strings(w282, "_" ("string"), w254, w281) -> (w295:string)
            n207 = case shown="1" w310 {
              tunnel: ["" "no active channel" "chZ " "chX  " "chZ & chX " "chY" "chZ & chY  " "chX & chY " "chZ& chX& chY " "INC_X " "chZ & INC_X  " "chX & INC_X" "chZ& chX & INC_X  " "chY & INC_X   " "chZ  & chY & INC_X " "chX  & chY & INC_X " "chZ& chX  & chY & INC_X " "INC_Y is " " chZ & INC_Y " " chX & INC_Y  " "chZ & chX & INC_Y " " chY & INC_Y  " "chZ & chY & INC_Y " "chX & chY & INC_Y  " " chZ &chX & chY & INC_Y" " INC_X & INC_Y " "chZ &   INC_X & INC_Y" "chX & INC_X & INC_Y  " " chZ & chX &  INC_X & INC_Y  " " chY &  INC_X & INC_Y " "chZ & chY &  INC_X & INC_Y " "chX & chY &  INC_X & INC_Y" "chZ & chX & chY &  INC_X & INC_Y"] -> w309
              tunnel: w308 -> [_ _ w444 w499 w556 w614 w672 w733 w797 w858 w916 w977 w1041 w1105 w1169 w1236 w1306 w1370 w1428 w1488 w1552 w1615 w1679 w1746 w1813 w1878 w1940 w2005 w2072 w2140 w2207 w2277 w2349]
              tunnel: [_ _ w441 w496 w552 w611 w670 w729 w793 w857 w913 w975 w1037 w1101 w1165 w1231 w1301 w1367 w1425 w1485 w1549 w1612 w1676 w1743 w1808 w1874 w1936 w2001 w2071 w2135 w2204 w2271 w2342] -> w278
              tunnel: w305 -> [_ _ w443 w498 w555 w612 w671 w732 w792 w856 w914 w976 w1040 w1104 w1168 w1235 w1305 w1369 w1427 w1487 w1551 w1614 w1678 w1744 w1809 w1877 w1939 w2002 w2068 w2139 w2206 w2275 w2344]
              tunnel: [_ _ w440 _ w551 _ w667 _ w791 _ w911 _ w1035 _ w1163 _ w1299 _ w1423 _ w1546 _ w1673 _ w1806 _ w1934 _ w2065 _ w2200 _ w2341] -> w321
              tunnel: [_ _ _ w495 w550 _ _ w728 w790 _ _ w972 w1034 _ _ w1230 w1298 _ _ w1483 w1545 _ _ w1740 w1805 _ _ w1999 w2064 _ _ w2270 w2340] -> w320
              tunnel: [_ _ _ _ _ w610 w666 w727 w789 _ _ _ _ w1100 w1162 w1229 w1297 _ _ _ _ w1610 w1672 w1739 w1804 _ _ _ _ w2134 w2199 w2269 w2339] -> w319
              tunnel: [_ _ _ _ _ _ _ _ _ w854 w910 w971 w1033 w1099 w1161 w1228 w1296 _ _ _ _ _ _ _ _ w1873 w1933 w1998 w2063 w2133 w2198 w2268 w2338] -> w318
              tunnel: [_ _ _ _ _ _ _ _ _ _ _ _ _ _ _ _ _ w1366 w1422 w1482 w1544 w1609 w1671 w1738 w1803 w1872 w1932 w1997 w2062 w2132 w2197 w2267 w2337] -> w317
              tunnel: w307 -> [_ _ w439 w493 w548 w608 w664 w725 w787 w852 w908 w969 w1031 w1097 w1159 w1226 w1294 w1364 w1420 w1480 w1542 w1607 w1669 w1736 w1801 w1870 w1930 w1995 w2060 w2130 w2195 w2265 w2335]
              tunnel: w306 -> [_ _ w438 w494 w549 w609 w665 w726 w788 w853 w909 w970 w1032 w1098 w1160 w1227 w1295 w1365 w1421 w1481 w1543 w1608 w1670 w1737 w1802 w1871 w1931 w1996 w2061 w2131 w2196 w2266 w2336]
              tunnel: w305 -> [_ _ w437 w492 w547 w607 w663 w724 w786 w851 w907 w968 w1030 w1096 w1158 w1225 w1293 w1363 w1419 w1479 w1541 w1606 w1668 w1735 w1800 w1869 w1929 w1994 w2059 w2129 w2194 w2264 w2334]
              tunnel: w304 -> [_ _ w436 w491 w546 w606 w662 w723 w785 w850 w906 w967 w1029 w1095 w1157 w1224 w1292 w1362 w1418 w1478 w1540 w1605 w1667 w1734 w1799 w1868 w1928 w1993 w2058 w2128 w2193 w2263 w2333]
              tunnel: [_ _ w435 _ w545 _ w661 _ w784 _ w905 _ w1028 _ w1156 _ w1291 _ w1417 _ w1539 _ w1666 _ w1798 _ w1927 _ w2057 _ w2192 _ w2332] -> w316
              tunnel: [_ _ _ w490 w545 _ _ w722 w783 _ _ w966 w1027 _ _ w1223 w1290 _ _ w1477 w1538 _ _ w1733 w1798 _ _ w1992 w2057 _ _ w2262 w2332] -> w315
              tunnel: [_ _ _ _ _ w605 w660 w721 w782 _ _ _ _ w1094 w1155 w1222 w1289 _ _ _ _ w1604 w1665 w1732 w1798 _ _ _ _ w2127 w2192 w2262 w2332] -> w314
              tunnel: [_ _ _ _ _ _ _ _ _ w849 w904 w965 w1026 w1093 w1154 w1221 w1288 _ _ _ _ _ _ _ _ w1867 w1927 w1992 w2057 w2127 w2192 w2262 w2332] -> w313
              tunnel: [_ _ _ _ _ _ _ _ _ _ _ _ _ _ _ _ _ w1361 w1416 w1477 w1537 w1604 w1664 w1731 w1798 w1867 w1927 w1992 w2057 w2127 w2192 w2262 w2332] -> w311
              tunnel: w295 -> [_ _ w421 w467 w522 w582 w636 w698 w759 w826 w881 w942 w1003 w1070 w1131 w1198 w1265 w1338 w1393 w1453 w1514 w1580 w1641 w1708 w1774 w1844 w1904 w1969 w2034 w2104 w2169 w2239 w2309]
              tunnel: [_ _ w411 w466 w521 w581 w637 w697 w758 w825 w880 w941 w1002 w1069 w1130 w1197 w1264 w1337 w1392 w1454 w1513 w1581 w1640 w1707 w1775 w1843 w1903 w1968 w2033 w2103 w2168 w2238 w2308] -> w312
              tunnel: w274 -> [_ _ w410 w465 w520 w580 w635 w696 w757 w824 w879 w940 w1001 w1068 w1129 w1196 w1263 w1336 w1391 w1452 w1512 w1579 w1639 w1706 w1773 w1842 w1902 w1967 w2032 w2102 w2167 w2237 w2307]
              frame Default {
              }
              frame 0 {
              }
              frame 1 {
                w416 = T13 2 items=["User Home"=0, "User Desktop"=1, "User Documents"=2, "User Application Data"=3, "User Preferences"=4, "User Temporary"=5, "Public Documents"=6, "Public Application Data"=7, "Public Preferences"=8, "Public Cache"=13, "System Core Libraries"=9, "System Installed Libraries"=10, "Application Files"=11, "Boot Volume Root"=12] ("system directory type")
                n208 = Decimate 1D Array(w444) -> (w442:dbl[])
                n209 = Search and Replace String(replace all?=TRUE ("replace all? (F)"), input string=w421, search string="/") -> (result string=w433:string)  [unwired: 5 in, 3 out]
                n210 = Concatenate Strings(w410, "TimeStamp;MeasureCh_Z(g);", "\n") -> (w426:string)
                n211 = for {
                  tunnel: w442 -> [w459] mode=indexing
                  tunnel: [w462] -> w441 mode=indexing
                  tunnel: w443 -> [w461] mode=indexing
                  tunnel: [w459] -> w440 mode=indexing
                  tunnel: w439 -> [w454]
                  tunnel: w438 -> [w453]
                  tunnel: w437 -> [w452] mode=indexing
                  tunnel: w436 -> [w451]
                  tunnel: [w449] -> w435
                  n212 = Join Numbers(hi=w453, lo=w454) -> ((hi.lo)=w456:u32)
                  n213 = To Double Precision Float(number=w452) -> (double precision float=w457:dbl)
                  n214 = Number To Decimal String(number=w461) -> (decimal integer string=w460:string)  [unwired: 1 in]
                  n215 = Number To Fractional String(number=w459, precision (6)=i16 3 ("width (-)")) -> (F-format string=w463:string)  [unwired: 2 in]
                  n216 = Divide(x=w457, y=w451) -> (x/y=w458:dbl)
                  n217 = To Unsigned Quad Integer(1:w456) -> (0:w455:u64)
                  n218 = Build Array(w460, w463) -> (w462:string[])
                  n219 = call "Unix Time to Timestamp.vi"("Fractional Second"=w458, "Unix Time (s)"=w455) -> ("Timestamp"=w450:timestamp)  [unwired: 8 in, 1 out]
                  n220 = To Double Precision Float(number=w450) -> (double precision float=w449:dbl)
                }
                n221 = call <vilib>:"Get System Directory.vi"("system directory type"=w416) -> ("system directory"=w427:path)  [unwired: 10 in]
                n222 = Concatenate Strings(w433, "_" ("string"), "streaming.csv") -> (w434:string)
                n223 = Build Path(base path=w427, name or relative path="Logfile") -> (appended path=w428:path)
                n224 = call <vilib>:"Check if File or Folder Exists.vi"("path"=w428) -> ("file or folder exists?"=w429:bool, "dup path"=w430:path)  [unwired: 8 in, 1 out]
                n225 = case shown="False" w429 {
                  tunnel: w430 -> [w447 w448]
                  tunnel: [w446 w448] -> w431
                  frame False {
                    n226 = Create Folder(path (use dialog)=w447) -> (created path=w446:path)  [unwired: 2 in, 2 out]
                  }
                  frame True {
                  }
                }
                n227 = Build Path(base path=w431, name or relative path=w434) -> (appended path=w432:path)
                n228 = Open/Create/Replace File(file path (use dialog)=w432, operation (0:open)=T10."open or create") -> (refnum out=w425:refnum<file>, error out=w423:errorcluster)  [unwired: 4 in, 1 out]
                n229 = Write to Text File(file (use dialog)=w425, text=w426, error in=w423) -> (refnum out=w424:refnum<file>, error out=w422:errorcluster)  [unwired: 1 in, 1 out]
                n230 = Close File(refnum=w424, error in=w422) -> (path=w411:path)  [unwired: 1 out]
              }
              frame 2 {
                w472 = T13 2 items=["User Home"=0, "User Desktop"=1, "User Documents"=2, "User Application Data"=3, "User Preferences"=4, "User Temporary"=5, "Public Documents"=6, "Public Application Data"=7, "Public Preferences"=8, "Public Cache"=13, "System Core Libraries"=9, "System Installed Libraries"=10, "Application Files"=11, "Boot Volume Root"=12] ("system directory type")
                n231 = Decimate 1D Array(w499) -> (w497:dbl[])
                n232 = Search and Replace String(replace all?=TRUE ("replace all? (F)"), input string=w467, search string="/") -> (result string=w488:string)  [unwired: 5 in, 3 out]
                n233 = for {
                  tunnel: w497 -> [w514] mode=indexing
                  tunnel: [w517] -> w496 mode=indexing
                  tunnel: w498 -> [w516] mode=indexing
                  tunnel: [w514] -> w495 mode=indexing
                  tunnel: w494 -> [w509]
                  tunnel: w493 -> [w508]
                  tunnel: w492 -> [w507] mode=indexing
                  tunnel: w491 -> [w506]
                  tunnel: [w504] -> w490
                  n234 = Join Numbers(hi=w509, lo=w508) -> ((hi.lo)=w511:u32)
                  n235 = To Double Precision Float(number=w507) -> (double precision float=w512:dbl)
                  n236 = Number To Decimal String(number=w516) -> (decimal integer string=w515:string)  [unwired: 1 in]
                  n237 = Number To Fractional String(number=w514, precision (6)=i16 3 ("width (-)")) -> (F-format string=w518:string)  [unwired: 2 in]
                  n238 = Divide(x=w512, y=w506) -> (x/y=w513:dbl)
                  n239 = To Unsigned Quad Integer(1:w511) -> (0:w510:u64)
                  n240 = Build Array(w515, w518) -> (w517:string[])
                  n241 = call "Unix Time to Timestamp.vi"("Fractional Second"=w513, "Unix Time (s)"=w510) -> ("Timestamp"=w505:timestamp)  [unwired: 8 in, 1 out]
                  n242 = To Double Precision Float(number=w505) -> (double precision float=w504:dbl)
                }
                n243 = Concatenate Strings(w465, "TimeStamp;MeasureCh_X(g);", "\n") -> (w481:string)
                n244 = call <vilib>:"Get System Directory.vi"("system directory type"=w472) -> ("system directory"=w482:path)  [unwired: 10 in]
                n245 = Concatenate Strings(w488, "_" ("string"), "streaming.csv") -> (w489:string)
                n246 = Build Path(base path=w482, name or relative path="Logfile") -> (appended path=w483:path)
                n247 = call <vilib>:"Check if File or Folder Exists.vi"("path"=w483) -> ("file or folder exists?"=w484:bool, "dup path"=w485:path)  [unwired: 8 in, 1 out]
                n248 = case shown="False" w484 {
                  tunnel: w485 -> [w502 w503]
                  tunnel: [w501 w503] -> w486
                  frame False {
                    n249 = Create Folder(path (use dialog)=w502) -> (created path=w501:path)  [unwired: 2 in, 2 out]
                  }
                  frame True {
                  }
                }
                n250 = Build Path(base path=w486, name or relative path=w489) -> (appended path=w487:path)
                n251 = Open/Create/Replace File(file path (use dialog)=w487, operation (0:open)=T10."open or create") -> (refnum out=w480:refnum<file>, error out=w478:errorcluster)  [unwired: 4 in, 1 out]
                n252 = Write to Text File(file (use dialog)=w480, text=w481, error in=w478) -> (refnum out=w479:refnum<file>, error out=w477:errorcluster)  [unwired: 1 in, 1 out]
                n253 = Close File(refnum=w479, error in=w477) -> (path=w466:path)  [unwired: 1 out]
              }
              frame 3 {
                w527 = T13 2 items=["User Home"=0, "User Desktop"=1, "User Documents"=2, "User Application Data"=3, "User Preferences"=4, "User Temporary"=5, "Public Documents"=6, "Public Application Data"=7, "Public Preferences"=8, "Public Cache"=13, "System Core Libraries"=9, "System Installed Libraries"=10, "Application Files"=11, "Boot Volume Root"=12] ("system directory type")
                n254 = Decimate 1D Array(w556) -> (w554:dbl[], w553:dbl[])
                n255 = Search and Replace String(replace all?=TRUE ("replace all? (F)"), input string=w522, search string="/") -> (result string=w543:string)  [unwired: 5 in, 3 out]
                n256 = for {
                  tunnel: w554 -> [w572] mode=indexing
                  tunnel: w553 -> [w571] mode=indexing
                  tunnel: [w575] -> w552 mode=indexing
                  tunnel: w555 -> [w574] mode=indexing
                  tunnel: [w572] -> w551 mode=indexing
                  tunnel: [w571] -> w550 mode=indexing
                  tunnel: w549 -> [w566]
                  tunnel: w548 -> [w565]
                  tunnel: w547 -> [w564] mode=indexing
                  tunnel: w546 -> [w563]
                  tunnel: [w561] -> w545
                  n257 = Join Numbers(hi=w566, lo=w565) -> ((hi.lo)=w568:u32)
                  n258 = To Double Precision Float(number=w564) -> (double precision float=w569:dbl)
                  n259 = Number To Decimal String(number=w574) -> (decimal integer string=w573:string)  [unwired: 1 in]
                  n260 = Number To Fractional String(number=w572, precision (6)=i16 3 ("width (-)")) -> (F-format string=w577:string)  [unwired: 2 in]
                  n261 = Number To Fractional String(number=w571, precision (6)=i16 3 ("width (-)")) -> (F-format string=w576:string)  [unwired: 2 in]
                  n262 = Divide(x=w569, y=w563) -> (x/y=w570:dbl)
                  n263 = To Unsigned Quad Integer(1:w568) -> (0:w567:u64)
                  n264 = Build Array(w573, w577, w576) -> (w575:string[])
                  n265 = call "Unix Time to Timestamp.vi"("Fractional Second"=w570, "Unix Time (s)"=w567) -> ("Timestamp"=w562:timestamp)  [unwired: 8 in, 1 out]
                  n266 = To Double Precision Float(number=w562) -> (double precision float=w561:dbl)
                }
                n267 = Concatenate Strings(w520, "TimeStamp;MeasureCh_Z(g);Ch_X(g);", "\n") -> (w536:string)
                n268 = call <vilib>:"Get System Directory.vi"("system directory type"=w527) -> ("system directory"=w537:path)  [unwired: 10 in]
                n269 = Concatenate Strings(w543, "_" ("string"), "streaming.csv") -> (w544:string)
                n270 = Build Path(base path=w537, name or relative path="Logfile") -> (appended path=w538:path)
                n271 = call <vilib>:"Check if File or Folder Exists.vi"("path"=w538) -> ("file or folder exists?"=w539:bool, "dup path"=w540:path)  [unwired: 8 in, 1 out]
                n272 = case shown="False" w539 {
                  tunnel: w540 -> [w559 w560]
                  tunnel: [w558 w560] -> w541
                  frame False {
                    n273 = Create Folder(path (use dialog)=w559) -> (created path=w558:path)  [unwired: 2 in, 2 out]
                  }
                  frame True {
                  }
                }
                n274 = Build Path(base path=w541, name or relative path=w544) -> (appended path=w542:path)
                n275 = Open/Create/Replace File(file path (use dialog)=w542, operation (0:open)=T10."open or create") -> (refnum out=w535:refnum<file>, error out=w533:errorcluster)  [unwired: 4 in, 1 out]
                n276 = Write to Text File(file (use dialog)=w535, text=w536, error in=w533) -> (refnum out=w534:refnum<file>, error out=w532:errorcluster)  [unwired: 1 in, 1 out]
                n277 = Close File(refnum=w534, error in=w532) -> (path=w521:path)  [unwired: 1 out]
              }
              frame 4 {
                w587 = T13 2 items=["User Home"=0, "User Desktop"=1, "User Documents"=2, "User Application Data"=3, "User Preferences"=4, "User Temporary"=5, "Public Documents"=6, "Public Application Data"=7, "Public Preferences"=8, "Public Cache"=13, "System Core Libraries"=9, "System Installed Libraries"=10, "Application Files"=11, "Boot Volume Root"=12] ("system directory type")
                n278 = Decimate 1D Array(w614) -> (w613:dbl[])
                n279 = Search and Replace String(replace all?=TRUE ("replace all? (F)"), input string=w582, search string="/") -> (result string=w603:string)  [unwired: 5 in, 3 out]
                n280 = for {
                  tunnel: w613 -> [w629] mode=indexing
                  tunnel: [w632] -> w611 mode=indexing
                  tunnel: w612 -> [w631] mode=indexing
                  tunnel: [w629] -> w610 mode=indexing
                  tunnel: w609 -> [w623]
                  tunnel: w608 -> [w620]
                  tunnel: w607 -> [w621] mode=indexing
                  tunnel: w606 -> [w622]
                  tunnel: [w619] -> w605
                  n281 = Join Numbers(hi=w623, lo=w620) -> ((hi.lo)=w626:u32)
                  n282 = To Double Precision Float(number=w621) -> (double precision float=w627:dbl)
                  n283 = Number To Decimal String(number=w631) -> (decimal integer string=w630:string)  [unwired: 1 in]
                  n284 = Number To Fractional String(number=w629, precision (6)=i16 3 ("width (-)")) -> (F-format string=w633:string)  [unwired: 2 in]
                  n285 = Divide(x=w627, y=w622) -> (x/y=w628:dbl)
                  n286 = To Unsigned Quad Integer(1:w626) -> (0:w625:u64)
                  n287 = Build Array(w630, w633) -> (w632:string[])
                  n288 = call "Unix Time to Timestamp.vi"("Fractional Second"=w628, "Unix Time (s)"=w625) -> ("Timestamp"=w624:timestamp)  [unwired: 8 in, 1 out]
                  n289 = To Double Precision Float(number=w624) -> (double precision float=w619:dbl)
                }
                n290 = Concatenate Strings(w580, "TimeStamp;MeasureCh_Y(g);", "\n") -> (w596:string)
                n291 = call <vilib>:"Get System Directory.vi"("system directory type"=w587) -> ("system directory"=w597:path)  [unwired: 10 in]
                n292 = Concatenate Strings(w603, "_" ("string"), "streaming.csv") -> (w604:string)
                n293 = Build Path(base path=w597, name or relative path="Logfile") -> (appended path=w598:path)
                n294 = call <vilib>:"Check if File or Folder Exists.vi"("path"=w598) -> ("file or folder exists?"=w599:bool, "dup path"=w600:path)  [unwired: 8 in, 1 out]
                n295 = case shown="False" w599 {
                  tunnel: w600 -> [w617 w618]
                  tunnel: [w616 w618] -> w601
                  frame False {
                    n296 = Create Folder(path (use dialog)=w617) -> (created path=w616:path)  [unwired: 2 in, 2 out]
                  }
                  frame True {
                  }
                }
                n297 = Build Path(base path=w601, name or relative path=w604) -> (appended path=w602:path)
                n298 = Open/Create/Replace File(file path (use dialog)=w602, operation (0:open)=T10."open or create") -> (refnum out=w595:refnum<file>, error out=w593:errorcluster)  [unwired: 4 in, 1 out]
                n299 = Write to Text File(file (use dialog)=w595, text=w596, error in=w593) -> (refnum out=w594:refnum<file>, error out=w592:errorcluster)  [unwired: 1 in, 1 out]
                n300 = Close File(refnum=w594, error in=w592) -> (path=w581:path)  [unwired: 1 out]
              }
              frame 5 {
                w642 = T13 2 items=["User Home"=0, "User Desktop"=1, "User Documents"=2, "User Application Data"=3, "User Preferences"=4, "User Temporary"=5, "Public Documents"=6, "Public Application Data"=7, "Public Preferences"=8, "Public Cache"=13, "System Core Libraries"=9, "System Installed Libraries"=10, "Application Files"=11, "Boot Volume Root"=12] ("system directory type")
                n301 = Decimate 1D Array(w672) -> (w668:dbl[], w669:dbl[])
                n302 = Search and Replace String(replace all?=TRUE ("replace all? (F)"), input string=w636, search string="/") -> (result string=w658:string)  [unwired: 5 in, 3 out]
                n303 = Concatenate Strings(w635, "TimeStamp;MeasureCh_Z(g);Ch_Y(g);", "\n") -> (w651:string)
                n304 = for {
                  tunnel: [w691] -> w670 mode=indexing
                  tunnel: w671 -> [w690] mode=indexing
                  tunnel: w668 -> [w688] mode=indexing
                  tunnel: w669 -> [w687] mode=indexing
                  tunnel: [w688] -> w667 mode=indexing
                  tunnel: [w687] -> w666 mode=indexing
                  tunnel: w665 -> [w681]
                  tunnel: w664 -> [w680]
                  tunnel: w663 -> [w679] mode=indexing
                  tunnel: w662 -> [w678]
                  tunnel: [w677] -> w661
                  tunnel: [w677] -> w660
                  n305 = Join Numbers(hi=w681, lo=w680) -> ((hi.lo)=w684:u32)
                  n306 = To Double Precision Float(number=w679) -> (double precision float=w685:dbl)
                  n307 = Number To Decimal String(number=w690) -> (decimal integer string=w689:string)  [unwired: 1 in]
                  n308 = Number To Fractional String(number=w688, precision (6)=i16 3 ("width (-)")) -> (F-format string=w693:string)  [unwired: 2 in]
                  n309 = Number To Fractional String(number=w687, precision (6)=i16 3 ("width (-)")) -> (F-format string=w692:string)  [unwired: 2 in]
                  n310 = Divide(x=w685, y=w678) -> (x/y=w686:dbl)
                  n311 = To Unsigned Quad Integer(1:w684) -> (0:w683:u64)
                  n312 = Build Array(w689, w693, w692) -> (w691:string[])
                  n313 = call "Unix Time to Timestamp.vi"("Fractional Second"=w686, "Unix Time (s)"=w683) -> ("Timestamp"=w682:timestamp)  [unwired: 8 in, 1 out]
                  n314 = To Double Precision Float(number=w682) -> (double precision float=w677:dbl)
                }
                n315 = call <vilib>:"Get System Directory.vi"("system directory type"=w642) -> ("system directory"=w652:path)  [unwired: 10 in]
                n316 = Concatenate Strings(w658, "_" ("string"), "streaming.csv") -> (w659:string)
                n317 = Build Path(base path=w652, name or relative path="Logfile") -> (appended path=w653:path)
                n318 = call <vilib>:"Check if File or Folder Exists.vi"("path"=w653) -> ("file or folder exists?"=w654:bool, "dup path"=w655:path)  [unwired: 8 in, 1 out]
                n319 = case shown="False" w654 {
                  tunnel: w655 -> [w675 w676]
                  tunnel: [w674 w676] -> w656
                  frame False {
                    n320 = Create Folder(path (use dialog)=w675) -> (created path=w674:path)  [unwired: 2 in, 2 out]
                  }
                  frame True {
                  }
                }
                n321 = Build Path(base path=w656, name or relative path=w659) -> (appended path=w657:path)
                n322 = Open/Create/Replace File(file path (use dialog)=w657, operation (0:open)=T10."open or create") -> (refnum out=w650:refnum<file>, error out=w648:errorcluster)  [unwired: 4 in, 1 out]
                n323 = Write to Text File(file (use dialog)=w650, text=w651, error in=w648) -> (refnum out=w649:refnum<file>, error out=w647:errorcluster)  [unwired: 1 in, 1 out]
                n324 = Close File(refnum=w649, error in=w647) -> (path=w637:path)  [unwired: 1 out]
              }
              frame 6 {
                w703 = T13 2 items=["User Home"=0, "User Desktop"=1, "User Documents"=2, "User Application Data"=3, "User Preferences"=4, "User Temporary"=5, "Public Documents"=6, "Public Application Data"=7, "Public Preferences"=8, "Public Cache"=13, "System Core Libraries"=9, "System Installed Libraries"=10, "Application Files"=11, "Boot Volume Root"=12] ("system directory type")
                n325 = Decimate 1D Array(w733) -> (w731:dbl[], w730:dbl[])
                n326 = Search and Replace String(replace all?=TRUE ("replace all? (F)"), input string=w698, search string="/") -> (result string=w719:string)  [unwired: 5 in, 3 out]
                n327 = for {
                  tunnel: w731 -> [w749] mode=indexing
                  tunnel: w730 -> [w748] mode=indexing
                  tunnel: [w752] -> w729 mode=indexing
                  tunnel: w732 -> [w751] mode=indexing
                  tunnel: [w749] -> w728 mode=indexing
                  tunnel: [w748] -> w727 mode=indexing
                  tunnel: w726 -> [w742]
                  tunnel: w725 -> [w741]
                  tunnel: w724 -> [w740] mode=indexing
                  tunnel: w723 -> [w739]
                  tunnel: [w738] -> w722
                  tunnel: [w738] -> w721
                  n328 = Join Numbers(hi=w742, lo=w741) -> ((hi.lo)=w745:u32)
                  n329 = To Double Precision Float(number=w740) -> (double precision float=w746:dbl)
                  n330 = Number To Decimal String(number=w751) -> (decimal integer string=w750:string)  [unwired: 1 in]
                  n331 = Number To Fractional String(number=w749, precision (6)=i16 3 ("width (-)")) -> (F-format string=w754:string)  [unwired: 2 in]
                  n332 = Number To Fractional String(number=w748, precision (6)=i16 3 ("width (-)")) -> (F-format string=w753:string)  [unwired: 2 in]
                  n333 = Divide(x=w746, y=w739) -> (x/y=w747:dbl)
                  n334 = To Unsigned Quad Integer(1:w745) -> (0:w744:u64)
                  n335 = Build Array(w750, w754, w753) -> (w752:string[])
                  n336 = call "Unix Time to Timestamp.vi"("Fractional Second"=w747, "Unix Time (s)"=w744) -> ("Timestamp"=w743:timestamp)  [unwired: 8 in, 1 out]
                  n337 = To Double Precision Float(number=w743) -> (double precision float=w738:dbl)
                }
                n338 = Concatenate Strings(w696, "TimeStamp;MeasureCh_X(g);Ch_Y(g);", "\n") -> (w712:string)
                n339 = call <vilib>:"Get System Directory.vi"("system directory type"=w703) -> ("system directory"=w713:path)  [unwired: 10 in]
                n340 = Concatenate Strings(w719, "_" ("string"), "streaming.csv") -> (w720:string)
                n341 = Build Path(base path=w713, name or relative path="Logfile") -> (appended path=w714:path)
                n342 = call <vilib>:"Check if File or Folder Exists.vi"("path"=w714) -> ("file or folder exists?"=w715:bool, "dup path"=w716:path)  [unwired: 8 in, 1 out]
                n343 = case shown="False" w715 {
                  tunnel: w716 -> [w736 w737]
                  tunnel: [w735 w737] -> w717
                  frame False {
                    n344 = Create Folder(path (use dialog)=w736) -> (created path=w735:path)  [unwired: 2 in, 2 out]
                  }
                  frame True {
                  }
                }
                n345 = Build Path(base path=w717, name or relative path=w720) -> (appended path=w718:path)
                n346 = Open/Create/Replace File(file path (use dialog)=w718, operation (0:open)=T10."open or create") -> (refnum out=w711:refnum<file>, error out=w709:errorcluster)  [unwired: 4 in, 1 out]
                n347 = Write to Text File(file (use dialog)=w711, text=w712, error in=w709) -> (refnum out=w710:refnum<file>, error out=w708:errorcluster)  [unwired: 1 in, 1 out]
                n348 = Close File(refnum=w710, error in=w708) -> (path=w697:path)  [unwired: 1 out]
              }
              frame 7 {
                w764 = T13 2 items=["User Home"=0, "User Desktop"=1, "User Documents"=2, "User Application Data"=3, "User Preferences"=4, "User Temporary"=5, "Public Documents"=6, "Public Application Data"=7, "Public Preferences"=8, "Public Cache"=13, "System Core Libraries"=9, "System Installed Libraries"=10, "Application Files"=11, "Boot Volume Root"=12] ("system directory type")
                n349 = Search and Replace String(replace all?=TRUE ("replace all? (F)"), input string=w759, search string="/") -> (result string=w780:string)  [unwired: 5 in, 3 out]
                n350 = Concatenate Strings(w757, "TimeStamp;MeasureCh_Z(g);Ch_X(g);Ch_Y(g);", "\n") -> (w773:string)
                n351 = call <vilib>:"Get System Directory.vi"("system directory type"=w764) -> ("system directory"=w774:path)  [unwired: 10 in]
                n352 = Concatenate Strings(w780, "_" ("string"), "streaming.csv") -> (w781:string)
                n353 = Build Path(base path=w774, name or relative path="Logfile") -> (appended path=w775:path)
                n354 = call <vilib>:"Check if File or Folder Exists.vi"("path"=w775) -> ("file or folder exists?"=w776:bool, "dup path"=w777:path)  [unwired: 8 in, 1 out]
                n355 = case shown="False" w776 {
                  tunnel: w777 -> [w800 w801]
                  tunnel: [w799 w801] -> w778
                  frame False {
                    n356 = Create Folder(path (use dialog)=w800) -> (created path=w799:path)  [unwired: 2 in, 2 out]
                  }
                  frame True {
                  }
                }
                n357 = Decimate 1D Array(w797) -> (w796:dbl[], w795:dbl[], w794:dbl[])
                n358 = for {
                  tunnel: w796 -> [w814] mode=indexing
                  tunnel: w795 -> [w813] mode=indexing
                  tunnel: w794 -> [w812] mode=indexing
                  tunnel: [w817] -> w793 mode=indexing
                  tunnel: w792 -> [w816] mode=indexing
                  tunnel: [w814] -> w791 mode=indexing
                  tunnel: [w813] -> w790 mode=indexing
                  tunnel: [w812] -> w789 mode=indexing
                  tunnel: w788 -> [w806]
                  tunnel: w787 -> [w805]
                  tunnel: w786 -> [w804] mode=indexing
                  tunnel: w785 -> [w803]
                  tunnel: [w802] -> w784
                  tunnel: [w802] -> w783
                  tunnel: [w802] -> w782
                  n359 = Join Numbers(hi=w806, lo=w805) -> ((hi.lo)=w809:u32)
                  n360 = To Double Precision Float(number=w804) -> (double precision float=w810:dbl)
                  n361 = Number To Decimal String(number=w816) -> (decimal integer string=w815:string)  [unwired: 1 in]
                  n362 = Number To Fractional String(number=w814, precision (6)=i16 3 ("width (-)")) -> (F-format string=w821:string)  [unwired: 2 in]
                  n363 = Number To Fractional String(number=w813, precision (6)=i16 3 ("width (-)")) -> (F-format string=w820:string)  [unwired: 2 in]
                  n364 = Number To Fractional String(number=w812, precision (6)=i16 3 ("width (-)")) -> (F-format string=w818:string)  [unwired: 2 in]
                  n365 = Divide(x=w810, y=w803) -> (x/y=w811:dbl)
                  n366 = To Unsigned Quad Integer(1:w809) -> (0:w808:u64)
                  n367 = Build Array(w815, w821, w820, w818) -> (w817:string[])
                  n368 = call "Unix Time to Timestamp.vi"("Fractional Second"=w811, "Unix Time (s)"=w808) -> ("Timestamp"=w807:timestamp)  [unwired: 8 in, 1 out]
                  n369 = To Double Precision Float(number=w807) -> (double precision float=w802:dbl)
                }
                n370 = Build Path(base path=w778, name or relative path=w781) -> (appended path=w779:path)
                n371 = Open/Create/Replace File(file path (use dialog)=w779, operation (0:open)=T10."open or create") -> (refnum out=w772:refnum<file>, error out=w770:errorcluster)  [unwired: 4 in, 1 out]
                n372 = Write to Text File(file (use dialog)=w772, text=w773, error in=w770) -> (refnum out=w771:refnum<file>, error out=w769:errorcluster)  [unwired: 1 in, 1 out]
                n373 = Close File(refnum=w771, error in=w769) -> (path=w758:path)  [unwired: 1 out]
              }
              frame 8 {
                w831 = T13 2 items=["User Home"=0, "User Desktop"=1, "User Documents"=2, "User Application Data"=3, "User Preferences"=4, "User Temporary"=5, "Public Documents"=6, "Public Application Data"=7, "Public Preferences"=8, "Public Cache"=13, "System Core Libraries"=9, "System Installed Libraries"=10, "Application Files"=11, "Boot Volume Root"=12] ("system directory type")
                n374 = Decimate 1D Array(w858) -> (w855:dbl[])
                n375 = Search and Replace String(replace all?=TRUE ("replace all? (F)"), input string=w826, search string="/") -> (result string=w847:string)  [unwired: 5 in, 3 out]
                n376 = Concatenate Strings(w824, "TimeStamp;Measure INC_X(Deg);", "\n") -> (w840:string)
                n377 = for {
                  tunnel: [w877] -> w857 mode=indexing
                  tunnel: w856 -> [w874] mode=indexing
                  tunnel: w855 -> [w873] mode=indexing
                  tunnel: [w873] -> w854 mode=indexing
                  tunnel: w853 -> [w867]
                  tunnel: w852 -> [w866]
                  tunnel: w851 -> [w865] mode=indexing
                  tunnel: w850 -> [w864]
                  tunnel: [w863] -> w849
                  n378 = Join Numbers(hi=w867, lo=w866) -> ((hi.lo)=w870:u32)
                  n379 = To Double Precision Float(number=w865) -> (double precision float=w871:dbl)
                  n380 = Number To Decimal String(number=w874) -> (decimal integer string=w876:string)  [unwired: 1 in]
                  n381 = Number To Fractional String(number=w873, precision (6)=i16 3 ("width (-)")) -> (F-format string=w875:string)  [unwired: 2 in]
                  n382 = Divide(x=w871, y=w864) -> (x/y=w872:dbl)
                  n383 = To Unsigned Quad Integer(1:w870) -> (0:w869:u64)
                  n384 = Build Array(w876, w875) -> (w877:string[])
                  n385 = call "Unix Time to Timestamp.vi"("Fractional Second"=w872, "Unix Time (s)"=w869) -> ("Timestamp"=w868:timestamp)  [unwired: 8 in, 1 out]
                  n386 = To Double Precision Float(number=w868) -> (double precision float=w863:dbl)
                }
                n387 = call <vilib>:"Get System Directory.vi"("system directory type"=w831) -> ("system directory"=w841:path)  [unwired: 10 in]
                n388 = Concatenate Strings(w847, "_" ("string"), "streaming.csv") -> (w848:string)
                n389 = Build Path(base path=w841, name or relative path="Logfile") -> (appended path=w842:path)
                n390 = call <vilib>:"Check if File or Folder Exists.vi"("path"=w842) -> ("file or folder exists?"=w843:bool, "dup path"=w844:path)  [unwired: 8 in, 1 out]
                n391 = case shown="False" w843 {
                  tunnel: w844 -> [w861 w862]
                  tunnel: [w860 w862] -> w845
                  frame False {
                    n392 = Create Folder(path (use dialog)=w861) -> (created path=w860:path)  [unwired: 2 in, 2 out]
                  }
                  frame True {
                  }
                }
                n393 = Build Path(base path=w845, name or relative path=w848) -> (appended path=w846:path)
                n394 = Open/Create/Replace File(file path (use dialog)=w846, operation (0:open)=T10."open or create") -> (refnum out=w839:refnum<file>, error out=w837:errorcluster)  [unwired: 4 in, 1 out]
                n395 = Write to Text File(file (use dialog)=w839, text=w840, error in=w837) -> (refnum out=w838:refnum<file>, error out=w836:errorcluster)  [unwired: 1 in, 1 out]
                n396 = Close File(refnum=w838, error in=w836) -> (path=w825:path)  [unwired: 1 out]
              }
              frame 9 {
                w886 = T13 2 items=["User Home"=0, "User Desktop"=1, "User Documents"=2, "User Application Data"=3, "User Preferences"=4, "User Temporary"=5, "Public Documents"=6, "Public Application Data"=7, "Public Preferences"=8, "Public Cache"=13, "System Core Libraries"=9, "System Installed Libraries"=10, "Application Files"=11, "Boot Volume Root"=12] ("system directory type")
                n397 = Decimate 1D Array(w916) -> (w912:dbl[], w915:dbl[])
                n398 = Search and Replace String(replace all?=TRUE ("replace all? (F)"), input string=w881, search string="/") -> (result string=w902:string)  [unwired: 5 in, 3 out]
                n399 = for {
                  tunnel: [w935] -> w913 mode=indexing
                  tunnel: w912 -> [w932] mode=indexing
                  tunnel: w915 -> [w931] mode=indexing
                  tunnel: w914 -> [w933] mode=indexing
                  tunnel: [w932] -> w911 mode=indexing
                  tunnel: [w931] -> w910 mode=indexing
                  tunnel: w909 -> [w925]
                  tunnel: w908 -> [w924]
                  tunnel: w907 -> [w923] mode=indexing
                  tunnel: w906 -> [w922]
                  tunnel: [w921] -> w904
                  tunnel: [w921] -> w905
                  n400 = Join Numbers(hi=w925, lo=w924) -> ((hi.lo)=w928:u32)
                  n401 = To Double Precision Float(number=w923) -> (double precision float=w929:dbl)
                  n402 = Number To Decimal String(number=w933) -> (decimal integer string=w934:string)  [unwired: 1 in]
                  n403 = Number To Fractional String(number=w932, precision (6)=i16 3 ("width (-)")) -> (F-format string=w937:string)  [unwired: 2 in]
                  n404 = Number To Fractional String(number=w931, precision (6)=i16 3 ("width (-)")) -> (F-format string=w936:string)  [unwired: 2 in]
                  n405 = Divide(x=w929, y=w922) -> (x/y=w930:dbl)
                  n406 = To Unsigned Quad Integer(1:w928) -> (0:w927:u64)
                  n407 = Build Array(w934, w937, w936) -> (w935:string[])
                  n408 = call "Unix Time to Timestamp.vi"("Fractional Second"=w930, "Unix Time (s)"=w927) -> ("Timestamp"=w926:timestamp)  [unwired: 8 in, 1 out]
                  n409 = To Double Precision Float(number=w926) -> (double precision float=w921:dbl)
                }
                n410 = Concatenate Strings(w879, "TimeStamp;Measure Ch_Z(g);INC_X(Deg);", "\n") -> (w895:string)
                n411 = call <vilib>:"Get System Directory.vi"("system directory type"=w886) -> ("system directory"=w896:path)  [unwired: 10 in]
                n412 = Concatenate Strings(w902, "_" ("string"), "streaming.csv") -> (w903:string)
                n413 = Build Path(base path=w896, name or relative path="Logfile") -> (appended path=w897:path)
                n414 = call <vilib>:"Check if File or Folder Exists.vi"("path"=w897) -> ("file or folder exists?"=w898:bool, "dup path"=w899:path)  [unwired: 8 in, 1 out]
                n415 = case shown="False" w898 {
                  tunnel: w899 -> [w919 w920]
                  tunnel: [w918 w920] -> w900
                  frame False {
                    n416 = Create Folder(path (use dialog)=w919) -> (created path=w918:path)  [unwired: 2 in, 2 out]
                  }
                  frame True {
                  }
                }
                n417 = Build Path(base path=w900, name or relative path=w903) -> (appended path=w901:path)
                n418 = Open/Create/Replace File(file path (use dialog)=w901, operation (0:open)=T10."open or create") -> (refnum out=w894:refnum<file>, error out=w892:errorcluster)  [unwired: 4 in, 1 out]
                n419 = Write to Text File(file (use dialog)=w894, text=w895, error in=w892) -> (refnum out=w893:refnum<file>, error out=w891:errorcluster)  [unwired: 1 in, 1 out]
                n420 = Close File(refnum=w893, error in=w891) -> (path=w880:path)  [unwired: 1 out]
              }
              frame 10 {
                w947 = T13 2 items=["User Home"=0, "User Desktop"=1, "User Documents"=2, "User Application Data"=3, "User Preferences"=4, "User Temporary"=5, "Public Documents"=6, "Public Application Data"=7, "Public Preferences"=8, "Public Cache"=13, "System Core Libraries"=9, "System Installed Libraries"=10, "Application Files"=11, "Boot Volume Root"=12] ("system directory type")
                n421 = Decimate 1D Array(w977) -> (w974:dbl[], w973:dbl[])
                n422 = Search and Replace String(replace all?=TRUE ("replace all? (F)"), input string=w942, search string="/") -> (result string=w963:string)  [unwired: 5 in, 3 out]
                n423 = for {
                  tunnel: [w994] -> _ mode=indexing
                  tunnel: [w998] -> w975 mode=indexing
                  tunnel: w976 -> [w997] mode=indexing
                  tunnel: w974 -> [w994] mode=indexing
                  tunnel: w973 -> [w993] mode=indexing
                  tunnel: [w994] -> w972 mode=indexing
                  tunnel: [w993] -> w971 mode=indexing
                  tunnel: w970 -> [w987]
                  tunnel: w969 -> [w986]
                  tunnel: w968 -> [w985] mode=indexing
                  tunnel: w967 -> [w984]
                  tunnel: [w983] -> w966
                  tunnel: [w983] -> w965
                  n424 = Join Numbers(hi=w987, lo=w986) -> ((hi.lo)=w990:u32)
                  n425 = To Double Precision Float(number=w985) -> (double precision float=w991:dbl)
                  n426 = Number To Decimal String(number=w997) -> (decimal integer string=w996:string)  [unwired: 1 in]
                  n427 = Number To Fractional String(number=w994, precision (6)=i16 3 ("width (-)")) -> (F-format string=w999:string)  [unwired: 2 in]
                  n428 = Number To Fractional String(number=w993, precision (6)=i16 3 ("width (-)")) -> (F-format string=w995:string)  [unwired: 2 in]
                  n429 = Divide(x=w991, y=w984) -> (x/y=w992:dbl)
                  n430 = To Unsigned Quad Integer(1:w990) -> (0:w989:u64)
                  n431 = Build Array(w996, w999, w995) -> (w998:string[])
                  n432 = call "Unix Time to Timestamp.vi"("Fractional Second"=w992, "Unix Time (s)"=w989) -> ("Timestamp"=w988:timestamp)  [unwired: 8 in, 1 out]
                  n433 = To Double Precision Float(number=w988) -> (double precision float=w983:dbl)
                }
                n434 = Concatenate Strings(w940, "TimeStamp;Measure Ch_X(g);INC_X(Deg);", "\n") -> (w956:string)
                n435 = call <vilib>:"Get System Directory.vi"("system directory type"=w947) -> ("system directory"=w957:path)  [unwired: 10 in]
                n436 = Concatenate Strings(w963, "_" ("string"), "streaming.csv") -> (w964:string)
                n437 = Build Path(base path=w957, name or relative path="Logfile") -> (appended path=w958:path)
                n438 = call <vilib>:"Check if File or Folder Exists.vi"("path"=w958) -> ("file or folder exists?"=w959:bool, "dup path"=w960:path)  [unwired: 8 in, 1 out]
                n439 = case shown="False" w959 {
                  tunnel: w960 -> [w980 w981]
                  tunnel: [w979 w981] -> w961
                  frame False {
                    n440 = Create Folder(path (use dialog)=w980) -> (created path=w979:path)  [unwired: 2 in, 2 out]
                  }
                  frame True {
                  }
                }
                n441 = Build Path(base path=w961, name or relative path=w964) -> (appended path=w962:path)
                n442 = Open/Create/Replace File(file path (use dialog)=w962, operation (0:open)=T10."open or create") -> (refnum out=w955:refnum<file>, error out=w953:errorcluster)  [unwired: 4 in, 1 out]
                n443 = Write to Text File(file (use dialog)=w955, text=w956, error in=w953) -> (refnum out=w954:refnum<file>, error out=w952:errorcluster)  [unwired: 1 in, 1 out]
                n444 = Close File(refnum=w954, error in=w952) -> (path=w941:path)  [unwired: 1 out]
              }
              frame 11 {
                w1008 = T13 2 items=["User Home"=0, "User Desktop"=1, "User Documents"=2, "User Application Data"=3, "User Preferences"=4, "User Temporary"=5, "Public Documents"=6, "Public Application Data"=7, "Public Preferences"=8, "Public Cache"=13, "System Core Libraries"=9, "System Installed Libraries"=10, "Application Files"=11, "Boot Volume Root"=12] ("system directory type")
                n445 = Search and Replace String(replace all?=TRUE ("replace all? (F)"), input string=w1003, search string="/") -> (result string=w1024:string)  [unwired: 5 in, 3 out]
                n446 = Concatenate Strings(w1001, "TimeStamp;Measure Ch_Z(g);Ch_X(g);INC_X(Deg);", "\n") -> (w1017:string)
                n447 = call <vilib>:"Get System Directory.vi"("system directory type"=w1008) -> ("system directory"=w1018:path)  [unwired: 10 in]
                n448 = Concatenate Strings(w1024, "_" ("string"), "streaming.csv") -> (w1025:string)
                n449 = Build Path(base path=w1018, name or relative path="Logfile") -> (appended path=w1019:path)
                n450 = call <vilib>:"Check if File or Folder Exists.vi"("path"=w1019) -> ("file or folder exists?"=w1020:bool, "dup path"=w1021:path)  [unwired: 8 in, 1 out]
                n451 = case shown="False" w1020 {
                  tunnel: w1021 -> [w1044 w1045]
                  tunnel: [w1043 w1045] -> w1022
                  frame False {
                    n452 = Create Folder(path (use dialog)=w1044) -> (created path=w1043:path)  [unwired: 2 in, 2 out]
                  }
                  frame True {
                  }
                }
                n453 = Decimate 1D Array(w1041) -> (w1039:dbl[], w1038:dbl[], w1036:dbl[])
                n454 = for {
                  tunnel: [w1065] -> w1037 mode=indexing
                  tunnel: w1040 -> [w1062] mode=indexing
                  tunnel: w1039 -> [w1060] mode=indexing
                  tunnel: w1038 -> [w1059] mode=indexing
                  tunnel: w1036 -> [w1058] mode=indexing
                  tunnel: [w1060] -> w1035 mode=indexing
                  tunnel: [w1059] -> w1034 mode=indexing
                  tunnel: [w1058] -> w1033 mode=indexing
                  tunnel: w1032 -> [w1052]
                  tunnel: w1031 -> [w1051]
                  tunnel: w1030 -> [w1050] mode=indexing
                  tunnel: w1029 -> [w1049]
                  tunnel: [w1048] -> w1028
                  tunnel: [w1048] -> w1027
                  tunnel: [w1048] -> w1026
                  n455 = Join Numbers(hi=w1052, lo=w1051) -> ((hi.lo)=w1055:u32)
                  n456 = To Double Precision Float(number=w1050) -> (double precision float=w1056:dbl)
                  n457 = Number To Decimal String(number=w1062) -> (decimal integer string=w1064:string)  [unwired: 1 in]
                  n458 = Number To Fractional String(number=w1060, precision (6)=i16 3 ("width (-)")) -> (F-format string=w1066:string)  [unwired: 2 in]
                  n459 = Number To Fractional String(number=w1059, precision (6)=i16 3 ("width (-)")) -> (F-format string=w1063:string)  [unwired: 2 in]
                  n460 = Number To Fractional String(number=w1058, precision (6)=i16 3 ("width (-)")) -> (F-format string=w1061:string)  [unwired: 2 in]
                  n461 = Divide(x=w1056, y=w1049) -> (x/y=w1057:dbl)
                  n462 = To Unsigned Quad Integer(1:w1055) -> (0:w1054:u64)
                  n463 = Build Array(w1064, w1066, w1063, w1061) -> (w1065:string[])
                  n464 = call "Unix Time to Timestamp.vi"("Fractional Second"=w1057, "Unix Time (s)"=w1054) -> ("Timestamp"=w1053:timestamp)  [unwired: 8 in, 1 out]
                  n465 = To Double Precision Float(number=w1053) -> (double precision float=w1048:dbl)
                }
                n466 = Build Path(base path=w1022, name or relative path=w1025) -> (appended path=w1023:path)
                n467 = Open/Create/Replace File(file path (use dialog)=w1023, operation (0:open)=T10."open or create") -> (refnum out=w1016:refnum<file>, error out=w1014:errorcluster)  [unwired: 4 in, 1 out]
                n468 = Write to Text File(file (use dialog)=w1016, text=w1017, error in=w1014) -> (refnum out=w1015:refnum<file>, error out=w1013:errorcluster)  [unwired: 1 in, 1 out]
                n469 = Close File(refnum=w1015, error in=w1013) -> (path=w1002:path)  [unwired: 1 out]
              }
              frame 12 {
                w1075 = T13 2 items=["User Home"=0, "User Desktop"=1, "User Documents"=2, "User Application Data"=3, "User Preferences"=4, "User Temporary"=5, "Public Documents"=6, "Public Application Data"=7, "Public Preferences"=8, "Public Cache"=13, "System Core Libraries"=9, "System Installed Libraries"=10, "Application Files"=11, "Boot Volume Root"=12] ("system directory type")
                n470 = Decimate 1D Array(w1105) -> (w1103:dbl[], w1102:dbl[])
                n471 = Search and Replace String(replace all?=TRUE ("replace all? (F)"), input string=w1070, search string="/") -> (result string=w1091:string)  [unwired: 5 in, 3 out]
                n472 = for {
                  tunnel: [w1126] -> w1101 mode=indexing
                  tunnel: w1104 -> [w1123] mode=indexing
                  tunnel: w1103 -> [w1122] mode=indexing
                  tunnel: w1102 -> [w1121] mode=indexing
                  tunnel: [w1122] -> w1100 mode=indexing
                  tunnel: [w1121] -> w1099 mode=indexing
                  tunnel: w1098 -> [w1115]
                  tunnel: w1097 -> [w1114]
                  tunnel: w1096 -> [w1113] mode=indexing
                  tunnel: w1095 -> [w1112]
                  tunnel: [w1111] -> w1094
                  tunnel: [w1111] -> w1093
                  n473 = Join Numbers(hi=w1115, lo=w1114) -> ((hi.lo)=w1118:u32)
                  n474 = To Double Precision Float(number=w1113) -> (double precision float=w1119:dbl)
                  n475 = Number To Decimal String(number=w1123) -> (decimal integer string=w1125:string)  [unwired: 1 in]
                  n476 = Number To Fractional String(number=w1122, precision (6)=i16 3 ("width (-)")) -> (F-format string=w1127:string)  [unwired: 2 in]
                  n477 = Number To Fractional String(number=w1121, precision (6)=i16 3 ("width (-)")) -> (F-format string=w1124:string)  [unwired: 2 in]
                  n478 = Divide(x=w1119, y=w1112) -> (x/y=w1120:dbl)
                  n479 = To Unsigned Quad Integer(1:w1118) -> (0:w1117:u64)
                  n480 = Build Array(w1125, w1127, w1124) -> (w1126:string[])
                  n481 = call "Unix Time to Timestamp.vi"("Fractional Second"=w1120, "Unix Time (s)"=w1117) -> ("Timestamp"=w1116:timestamp)  [unwired: 8 in, 1 out]
                  n482 = To Double Precision Float(number=w1116) -> (double precision float=w1111:dbl)
                }
                n483 = Concatenate Strings(w1068, "TimeStamp;Measure Ch_Y(g);INC_X(Deg);", "\n") -> (w1084:string)
                n484 = call <vilib>:"Get System Directory.vi"("system directory type"=w1075) -> ("system directory"=w1085:path)  [unwired: 10 in]
                n485 = Concatenate Strings(w1091, "_" ("string"), "streaming.csv") -> (w1092:string)
                n486 = Build Path(base path=w1085, name or relative path="Logfile") -> (appended path=w1086:path)
                n487 = call <vilib>:"Check if File or Folder Exists.vi"("path"=w1086) -> ("file or folder exists?"=w1087:bool, "dup path"=w1088:path)  [unwired: 8 in, 1 out]
                n488 = case shown="False" w1087 {
                  tunnel: w1088 -> [w1108 w1109]
                  tunnel: [w1107 w1109] -> w1089
                  frame False {
                    n489 = Create Folder(path (use dialog)=w1108) -> (created path=w1107:path)  [unwired: 2 in, 2 out]
                  }
                  frame True {
                  }
                }
                n490 = Build Path(base path=w1089, name or relative path=w1092) -> (appended path=w1090:path)
                n491 = Open/Create/Replace File(file path (use dialog)=w1090, operation (0:open)=T10."open or create") -> (refnum out=w1083:refnum<file>, error out=w1081:errorcluster)  [unwired: 4 in, 1 out]
                n492 = Write to Text File(file (use dialog)=w1083, text=w1084, error in=w1081) -> (refnum out=w1082:refnum<file>, error out=w1080:errorcluster)  [unwired: 1 in, 1 out]
                n493 = Close File(refnum=w1082, error in=w1080) -> (path=w1069:path)  [unwired: 1 out]
              }
              frame 13 {
                w1136 = T13 2 items=["User Home"=0, "User Desktop"=1, "User Documents"=2, "User Application Data"=3, "User Preferences"=4, "User Temporary"=5, "Public Documents"=6, "Public Application Data"=7, "Public Preferences"=8, "Public Cache"=13, "System Core Libraries"=9, "System Installed Libraries"=10, "Application Files"=11, "Boot Volume Root"=12] ("system directory type")
                n494 = Search and Replace String(replace all?=TRUE ("replace all? (F)"), input string=w1131, search string="/") -> (result string=w1152:string)  [unwired: 5 in, 3 out]
                n495 = Concatenate Strings(w1129, "TimeStamp;Measure Ch_Z(g);Ch_Y(g);INC_X(Deg)", "\n") -> (w1145:string)
                n496 = call <vilib>:"Get System Directory.vi"("system directory type"=w1136) -> ("system directory"=w1146:path)  [unwired: 10 in]
                n497 = Concatenate Strings(w1152, "_" ("string"), "streaming.csv") -> (w1153:string)
                n498 = Build Path(base path=w1146, name or relative path="Logfile") -> (appended path=w1147:path)
                n499 = call <vilib>:"Check if File or Folder Exists.vi"("path"=w1147) -> ("file or folder exists?"=w1148:bool, "dup path"=w1149:path)  [unwired: 8 in, 1 out]
                n500 = case shown="False" w1148 {
                  tunnel: w1149 -> [w1172 w1173]
                  tunnel: [w1171 w1173] -> w1150
                  frame False {
                    n501 = Create Folder(path (use dialog)=w1172) -> (created path=w1171:path)  [unwired: 2 in, 2 out]
                  }
                  frame True {
                  }
                }
                n502 = Decimate 1D Array(w1169) -> (w1164:dbl[], w1167:dbl[], w1166:dbl[])
                n503 = for {
                  tunnel: [w1193] -> w1165 mode=indexing
                  tunnel: w1168 -> [w1189] mode=indexing
                  tunnel: w1164 -> [w1188] mode=indexing
                  tunnel: w1167 -> [w1187] mode=indexing
                  tunnel: w1166 -> [w1186] mode=indexing
                  tunnel: [w1188] -> w1163 mode=indexing
                  tunnel: [w1187] -> w1162 mode=indexing
                  tunnel: [w1186] -> w1161 mode=indexing
                  tunnel: w1160 -> [w1180]
                  tunnel: w1159 -> [w1179]
                  tunnel: w1158 -> [w1178] mode=indexing
                  tunnel: w1157 -> [w1177]
                  tunnel: [w1176] -> w1156
                  tunnel: [w1176] -> w1155
                  tunnel: [w1176] -> w1154
                  n504 = Join Numbers(hi=w1180, lo=w1179) -> ((hi.lo)=w1183:u32)
                  n505 = To Double Precision Float(number=w1178) -> (double precision float=w1184:dbl)
                  n506 = Number To Decimal String(number=w1189) -> (decimal integer string=w1192:string)  [unwired: 1 in]
                  n507 = Number To Fractional String(number=w1188, precision (6)=i16 3 ("width (-)")) -> (F-format string=w1194:string)  [unwired: 2 in]
                  n508 = Number To Fractional String(number=w1187, precision (6)=i16 3 ("width (-)")) -> (F-format string=w1191:string)  [unwired: 2 in]
                  n509 = Number To Fractional String(number=w1186, precision (6)=i16 3 ("width (-)")) -> (F-format string=w1190:string)  [unwired: 2 in]
                  n510 = Divide(x=w1184, y=w1177) -> (x/y=w1185:dbl)
                  n511 = To Unsigned Quad Integer(1:w1183) -> (0:w1182:u64)
                  n512 = Build Array(w1192, w1194, w1191, w1190) -> (w1193:string[])
                  n513 = call "Unix Time to Timestamp.vi"("Fractional Second"=w1185, "Unix Time (s)"=w1182) -> ("Timestamp"=w1181:timestamp)  [unwired: 8 in, 1 out]
                  n514 = To Double Precision Float(number=w1181) -> (double precision float=w1176:dbl)
                }
                n515 = Build Path(base path=w1150, name or relative path=w1153) -> (appended path=w1151:path)
                n516 = Open/Create/Replace File(file path (use dialog)=w1151, operation (0:open)=T10."open or create") -> (refnum out=w1144:refnum<file>, error out=w1142:errorcluster)  [unwired: 4 in, 1 out]
                n517 = Write to Text File(file (use dialog)=w1144, text=w1145, error in=w1142) -> (refnum out=w1143:refnum<file>, error out=w1141:errorcluster)  [unwired: 1 in, 1 out]
                n518 = Close File(refnum=w1143, error in=w1141) -> (path=w1130:path)  [unwired: 1 out]
              }
              frame 14 {
                w1203 = T13 2 items=["User Home"=0, "User Desktop"=1, "User Documents"=2, "User Application Data"=3, "User Preferences"=4, "User Temporary"=5, "Public Documents"=6, "Public Application Data"=7, "Public Preferences"=8, "Public Cache"=13, "System Core Libraries"=9, "System Installed Libraries"=10, "Application Files"=11, "Boot Volume Root"=12] ("system directory type")
                n519 = Search and Replace String(replace all?=TRUE ("replace all? (F)"), input string=w1198, search string="/") -> (result string=w1219:string)  [unwired: 5 in, 3 out]
                n520 = Concatenate Strings(w1196, "TimeStamp;Measure Ch_X(g);Ch_Y(g);INC_X(Deg)", "\n") -> (w1212:string)
                n521 = call <vilib>:"Get System Directory.vi"("system directory type"=w1203) -> ("system directory"=w1213:path)  [unwired: 10 in]
                n522 = Concatenate Strings(w1219, "_" ("string"), "streaming.csv") -> (w1220:string)
                n523 = Build Path(base path=w1213, name or relative path="Logfile") -> (appended path=w1214:path)
                n524 = call <vilib>:"Check if File or Folder Exists.vi"("path"=w1214) -> ("file or folder exists?"=w1215:bool, "dup path"=w1216:path)  [unwired: 8 in, 1 out]
                n525 = case shown="False" w1215 {
                  tunnel: w1216 -> [w1239 w1240]
                  tunnel: [w1238 w1240] -> w1217
                  frame False {
                    n526 = Create Folder(path (use dialog)=w1239) -> (created path=w1238:path)  [unwired: 2 in, 2 out]
                  }
                  frame True {
                  }
                }
                n527 = Decimate 1D Array(w1236) -> (w1234:dbl[], w1233:dbl[], w1232:dbl[])
                n528 = for {
                  tunnel: [w1260] -> w1231 mode=indexing
                  tunnel: w1235 -> [w1256] mode=indexing
                  tunnel: w1234 -> [w1255] mode=indexing
                  tunnel: w1233 -> [w1254] mode=indexing
                  tunnel: w1232 -> [w1253] mode=indexing
                  tunnel: [w1255] -> w1230 mode=indexing
                  tunnel: [w1254] -> w1229 mode=indexing
                  tunnel: [w1253] -> w1228 mode=indexing
                  tunnel: w1227 -> [w1247]
                  tunnel: w1226 -> [w1246]
                  tunnel: w1225 -> [w1245] mode=indexing
                  tunnel: w1224 -> [w1244]
                  tunnel: [w1243] -> w1223
                  tunnel: [w1243] -> w1222
                  tunnel: [w1243] -> w1221
                  n529 = Join Numbers(hi=w1247, lo=w1246) -> ((hi.lo)=w1250:u32)
                  n530 = To Double Precision Float(number=w1245) -> (double precision float=w1251:dbl)
                  n531 = Number To Decimal String(number=w1256) -> (decimal integer string=w1259:string)  [unwired: 1 in]
                  n532 = Number To Fractional String(number=w1255, precision (6)=i16 3 ("width (-)")) -> (F-format string=w1261:string)  [unwired: 2 in]
                  n533 = Number To Fractional String(number=w1254, precision (6)=i16 3 ("width (-)")) -> (F-format string=w1258:string)  [unwired: 2 in]
                  n534 = Number To Fractional String(number=w1253, precision (6)=i16 3 ("width (-)")) -> (F-format string=w1257:string)  [unwired: 2 in]
                  n535 = Divide(x=w1251, y=w1244) -> (x/y=w1252:dbl)
                  n536 = To Unsigned Quad Integer(1:w1250) -> (0:w1249:u64)
                  n537 = Build Array(w1259, w1261, w1258, w1257) -> (w1260:string[])
                  n538 = call "Unix Time to Timestamp.vi"("Fractional Second"=w1252, "Unix Time (s)"=w1249) -> ("Timestamp"=w1248:timestamp)  [unwired: 8 in, 1 out]
                  n539 = To Double Precision Float(number=w1248) -> (double precision float=w1243:dbl)
                }
                n540 = Build Path(base path=w1217, name or relative path=w1220) -> (appended path=w1218:path)
                n541 = Open/Create/Replace File(file path (use dialog)=w1218, operation (0:open)=T10."open or create") -> (refnum out=w1211:refnum<file>, error out=w1209:errorcluster)  [unwired: 4 in, 1 out]
                n542 = Write to Text File(file (use dialog)=w1211, text=w1212, error in=w1209) -> (refnum out=w1210:refnum<file>, error out=w1208:errorcluster)  [unwired: 1 in, 1 out]
                n543 = Close File(refnum=w1210, error in=w1208) -> (path=w1197:path)  [unwired: 1 out]
              }
              frame 15 {
                w1270 = T13 2 items=["User Home"=0, "User Desktop"=1, "User Documents"=2, "User Application Data"=3, "User Preferences"=4, "User Temporary"=5, "Public Documents"=6, "Public Application Data"=7, "Public Preferences"=8, "Public Cache"=13, "System Core Libraries"=9, "System Installed Libraries"=10, "Application Files"=11, "Boot Volume Root"=12] ("system directory type")
                n544 = Search and Replace String(replace all?=TRUE ("replace all? (F)"), input string=w1265, search string="/") -> (result string=w1286:string)  [unwired: 5 in, 3 out]
                n545 = Concatenate Strings(w1263, "TimeStamp;MeasureCh_Z(g);Ch_X(g);Ch_Y(g);INC_X(Deg)", "\n") -> (w1279:string)
                n546 = call <vilib>:"Get System Directory.vi"("system directory type"=w1270) -> ("system directory"=w1280:path)  [unwired: 10 in]
                n547 = Concatenate Strings(w1286, "_" ("string"), "streaming.csv") -> (w1287:string)
                n548 = Build Path(base path=w1280, name or relative path="Logfile") -> (appended path=w1281:path)
                n549 = call <vilib>:"Check if File or Folder Exists.vi"("path"=w1281) -> ("file or folder exists?"=w1282:bool, "dup path"=w1283:path)  [unwired: 8 in, 1 out]
                n550 = case shown="False" w1282 {
                  tunnel: w1283 -> [w1309 w1310]
                  tunnel: [w1308 w1310] -> w1284
                  frame False {
                    n551 = Create Folder(path (use dialog)=w1309) -> (created path=w1308:path)  [unwired: 2 in, 2 out]
                  }
                  frame True {
                  }
                }
                n552 = Decimate 1D Array(w1306) -> (w1304:dbl[], w1303:dbl[], w1302:dbl[], w1300:dbl[])
                n553 = for {
                  tunnel: [w1333] -> w1301 mode=indexing
                  tunnel: w1305 -> [w1328] mode=indexing
                  tunnel: w1304 -> [w1327] mode=indexing
                  tunnel: w1303 -> [w1326] mode=indexing
                  tunnel: w1302 -> [w1325] mode=indexing
                  tunnel: w1300 -> [w1324] mode=indexing
                  tunnel: [w1327] -> w1299 mode=indexing
                  tunnel: [w1326] -> w1298 mode=indexing
                  tunnel: [w1325] -> w1297 mode=indexing
                  tunnel: [w1324] -> w1296 mode=indexing
                  tunnel: w1295 -> [w1318]
                  tunnel: w1294 -> [w1317]
                  tunnel: w1293 -> [w1316] mode=indexing
                  tunnel: w1292 -> [w1315]
                  tunnel: [w1314] -> w1291
                  tunnel: [w1314] -> w1290
                  tunnel: [w1314] -> w1289
                  tunnel: [w1314] -> w1288
                  n554 = Join Numbers(hi=w1318, lo=w1317) -> ((hi.lo)=w1321:u32)
                  n555 = To Double Precision Float(number=w1316) -> (double precision float=w1322:dbl)
                  n556 = Number To Decimal String(number=w1328) -> (decimal integer string=w1332:string)  [unwired: 1 in]
                  n557 = Number To Fractional String(number=w1327, precision (6)=i16 3 ("width (-)")) -> (F-format string=w1334:string)  [unwired: 2 in]
                  n558 = Number To Fractional String(number=w1326, precision (6)=i16 3 ("width (-)")) -> (F-format string=w1331:string)  [unwired: 2 in]
                  n559 = Number To Fractional String(number=w1325, precision (6)=i16 3 ("width (-)")) -> (F-format string=w1330:string)  [unwired: 2 in]
                  n560 = Number To Fractional String(number=w1324, precision (6)=i16 3 ("width (-)")) -> (F-format string=w1329:string)  [unwired: 2 in]
                  n561 = Divide(x=w1322, y=w1315) -> (x/y=w1323:dbl)
                  n562 = To Unsigned Quad Integer(1:w1321) -> (0:w1320:u64)
                  n563 = Build Array(w1332, w1334, w1331, w1330, w1329) -> (w1333:string[])
                  n564 = call "Unix Time to Timestamp.vi"("Fractional Second"=w1323, "Unix Time (s)"=w1320) -> ("Timestamp"=w1319:timestamp)  [unwired: 8 in, 1 out]
                  n565 = To Double Precision Float(number=w1319) -> (double precision float=w1314:dbl)
                }
                n566 = Build Path(base path=w1284, name or relative path=w1287) -> (appended path=w1285:path)
                n567 = Open/Create/Replace File(file path (use dialog)=w1285, operation (0:open)=T10."open or create") -> (refnum out=w1278:refnum<file>, error out=w1276:errorcluster)  [unwired: 4 in, 1 out]
                n568 = Write to Text File(file (use dialog)=w1278, text=w1279, error in=w1276) -> (refnum out=w1277:refnum<file>, error out=w1275:errorcluster)  [unwired: 1 in, 1 out]
                n569 = Close File(refnum=w1277, error in=w1275) -> (path=w1264:path)  [unwired: 1 out]
              }
              frame 16 {
                w1343 = T13 2 items=["User Home"=0, "User Desktop"=1, "User Documents"=2, "User Application Data"=3, "User Preferences"=4, "User Temporary"=5, "Public Documents"=6, "Public Application Data"=7, "Public Preferences"=8, "Public Cache"=13, "System Core Libraries"=9, "System Installed Libraries"=10, "Application Files"=11, "Boot Volume Root"=12] ("system directory type")
                n570 = Decimate 1D Array(w1370) -> (w1368:dbl[])
                n571 = Search and Replace String(replace all?=TRUE ("replace all? (F)"), input string=w1338, search string="/") -> (result string=w1359:string)  [unwired: 5 in, 3 out]
                n572 = for {
                  tunnel: [w1388] -> w1367 mode=indexing
                  tunnel: w1369 -> [w1386] mode=indexing
                  tunnel: w1368 -> [w1385] mode=indexing
                  tunnel: [w1385] -> w1366 mode=indexing
                  tunnel: w1365 -> [w1379]
                  tunnel: w1364 -> [w1378]
                  tunnel: w1363 -> [w1377] mode=indexing
                  tunnel: w1362 -> [w1376]
                  tunnel: [w1375] -> w1361
                  n573 = Join Numbers(hi=w1379, lo=w1378) -> ((hi.lo)=w1382:u32)
                  n574 = To Double Precision Float(number=w1377) -> (double precision float=w1383:dbl)
                  n575 = Number To Decimal String(number=w1386) -> (decimal integer string=w1387:string)  [unwired: 1 in]
                  n576 = Number To Fractional String(number=w1385, precision (6)=i16 3 ("width (-)")) -> (F-format string=w1389:string)  [unwired: 2 in]
                  n577 = Divide(x=w1383, y=w1376) -> (x/y=w1384:dbl)
                  n578 = To Unsigned Quad Integer(1:w1382) -> (0:w1381:u64)
                  n579 = Build Array(w1387, w1389) -> (w1388:string[])
                  n580 = call "Unix Time to Timestamp.vi"("Fractional Second"=w1384, "Unix Time (s)"=w1381) -> ("Timestamp"=w1380:timestamp)  [unwired: 8 in, 1 out]
                  n581 = To Double Precision Float(number=w1380) -> (double precision float=w1375:dbl)
                }
                n582 = Concatenate Strings(w1336, "TimeStamp;MeasureINC_Y(Deg)", "\n") -> (w1352:string)
                n583 = call <vilib>:"Get System Directory.vi"("system directory type"=w1343) -> ("system directory"=w1353:path)  [unwired: 10 in]
                n584 = Concatenate Strings(w1359, "_" ("string"), "streaming.csv") -> (w1360:string)
                n585 = Build Path(base path=w1353, name or relative path="Logfile") -> (appended path=w1354:path)
                n586 = call <vilib>:"Check if File or Folder Exists.vi"("path"=w1354) -> ("file or folder exists?"=w1355:bool, "dup path"=w1356:path)  [unwired: 8 in, 1 out]
                n587 = case shown="False" w1355 {
                  tunnel: w1356 -> [w1373 w1374]
                  tunnel: [w1372 w1374] -> w1357
                  frame False {
                    n588 = Create Folder(path (use dialog)=w1373) -> (created path=w1372:path)  [unwired: 2 in, 2 out]
                  }
                  frame True {
                  }
                }
                n589 = Build Path(base path=w1357, name or relative path=w1360) -> (appended path=w1358:path)
                n590 = Open/Create/Replace File(file path (use dialog)=w1358, operation (0:open)=T10."open or create") -> (refnum out=w1351:refnum<file>, error out=w1349:errorcluster)  [unwired: 4 in, 1 out]
                n591 = Write to Text File(file (use dialog)=w1351, text=w1352, error in=w1349) -> (refnum out=w1350:refnum<file>, error out=w1348:errorcluster)  [unwired: 1 in, 1 out]
                n592 = Close File(refnum=w1350, error in=w1348) -> (path=w1337:path)  [unwired: 1 out]
              }
              frame 17 {
                w1398 = T13 2 items=["User Home"=0, "User Desktop"=1, "User Documents"=2, "User Application Data"=3, "User Preferences"=4, "User Temporary"=5, "Public Documents"=6, "Public Application Data"=7, "Public Preferences"=8, "Public Cache"=13, "System Core Libraries"=9, "System Installed Libraries"=10, "Application Files"=11, "Boot Volume Root"=12] ("system directory type")
                n593 = Decimate 1D Array(w1428) -> (w1424:dbl[], w1426:dbl[])
                n594 = Search and Replace String(replace all?=TRUE ("replace all? (F)"), input string=w1393, search string="/") -> (result string=w1414:string)  [unwired: 5 in, 3 out]
                n595 = for {
                  tunnel: [w1449] -> w1425 mode=indexing
                  tunnel: w1427 -> [w1447] mode=indexing
                  tunnel: w1424 -> [w1444] mode=indexing
                  tunnel: w1426 -> [w1443] mode=indexing
                  tunnel: [w1444] -> w1423 mode=indexing
                  tunnel: [w1443] -> w1422 mode=indexing
                  tunnel: w1421 -> [w1437]
                  tunnel: w1420 -> [w1436]
                  tunnel: w1419 -> [w1435] mode=indexing
                  tunnel: w1418 -> [w1434]
                  tunnel: [w1433] -> w1417
                  tunnel: [w1433] -> w1416
                  n596 = Join Numbers(hi=w1437, lo=w1436) -> ((hi.lo)=w1440:u32)
                  n597 = To Double Precision Float(number=w1435) -> (double precision float=w1441:dbl)
                  n598 = Number To Decimal String(number=w1447) -> (decimal integer string=w1448:string)  [unwired: 1 in]
                  n599 = Number To Fractional String(number=w1444, precision (6)=i16 3 ("width (-)")) -> (F-format string=w1450:string)  [unwired: 2 in]
                  n600 = Number To Fractional String(number=w1443, precision (6)=i16 3 ("width (-)")) -> (F-format string=w1445:string)  [unwired: 2 in]
                  n601 = Divide(x=w1441, y=w1434) -> (x/y=w1442:dbl)
                  n602 = To Unsigned Quad Integer(1:w1440) -> (0:w1439:u64)
                  n603 = Build Array(w1448, w1450, w1445) -> (w1449:string[])
                  n604 = call "Unix Time to Timestamp.vi"("Fractional Second"=w1442, "Unix Time (s)"=w1439) -> ("Timestamp"=w1438:timestamp)  [unwired: 8 in, 1 out]
                  n605 = To Double Precision Float(number=w1438) -> (double precision float=w1433:dbl)
                }
                n606 = Concatenate Strings(w1391, "TimeStamp;MeasureCh_Z(g);INC_Y(Deg)", "\n") -> (w1407:string)
                n607 = call <vilib>:"Get System Directory.vi"("system directory type"=w1398) -> ("system directory"=w1408:path)  [unwired: 10 in]
                n608 = Concatenate Strings(w1414, "_" ("string"), "streaming.csv") -> (w1415:string)
                n609 = Build Path(base path=w1408, name or relative path="Logfile") -> (appended path=w1409:path)
                n610 = call <vilib>:"Check if File or Folder Exists.vi"("path"=w1409) -> ("file or folder exists?"=w1410:bool, "dup path"=w1411:path)  [unwired: 8 in, 1 out]
                n611 = case shown="False" w1410 {
                  tunnel: w1411 -> [w1431 w1432]
                  tunnel: [w1430 w1432] -> w1412
                  frame False {
                    n612 = Create Folder(path (use dialog)=w1431) -> (created path=w1430:path)  [unwired: 2 in, 2 out]
                  }
                  frame True {
                  }
                }
                n613 = Build Path(base path=w1412, name or relative path=w1415) -> (appended path=w1413:path)
                n614 = Open/Create/Replace File(file path (use dialog)=w1413, operation (0:open)=T10."open or create") -> (refnum out=w1406:refnum<file>, error out=w1404:errorcluster)  [unwired: 4 in, 1 out]
                n615 = Write to Text File(file (use dialog)=w1406, text=w1407, error in=w1404) -> (refnum out=w1405:refnum<file>, error out=w1403:errorcluster)  [unwired: 1 in, 1 out]
                n616 = Close File(refnum=w1405, error in=w1403) -> (path=w1392:path)  [unwired: 1 out]
              }
              frame 18 {
                w1459 = T13 2 items=["User Home"=0, "User Desktop"=1, "User Documents"=2, "User Application Data"=3, "User Preferences"=4, "User Temporary"=5, "Public Documents"=6, "Public Application Data"=7, "Public Preferences"=8, "Public Cache"=13, "System Core Libraries"=9, "System Installed Libraries"=10, "Application Files"=11, "Boot Volume Root"=12] ("system directory type")
                n617 = Decimate 1D Array(w1488) -> (w1484:dbl[], w1486:dbl[])
                n618 = Search and Replace String(replace all?=TRUE ("replace all? (F)"), input string=w1453, search string="/") -> (result string=w1475:string)  [unwired: 5 in, 3 out]
                n619 = for {
                  tunnel: [w1509] -> w1485 mode=indexing
                  tunnel: w1487 -> [w1505] mode=indexing
                  tunnel: w1484 -> [w1504] mode=indexing
                  tunnel: w1486 -> [w1503] mode=indexing
                  tunnel: [w1504] -> w1483 mode=indexing
                  tunnel: [w1503] -> w1482 mode=indexing
                  tunnel: w1481 -> [w1497]
                  tunnel: w1480 -> [w1496]
                  tunnel: w1479 -> [w1495] mode=indexing
                  tunnel: w1478 -> [w1494]
                  tunnel: [w1493] -> w1477
                  n620 = Join Numbers(hi=w1497, lo=w1496) -> ((hi.lo)=w1500:u32)
                  n621 = To Double Precision Float(number=w1495) -> (double precision float=w1501:dbl)
                  n622 = Number To Decimal String(number=w1505) -> (decimal integer string=w1508:string)  [unwired: 1 in]
                  n623 = Number To Fractional String(number=w1504, precision (6)=i16 3 ("width (-)")) -> (F-format string=w1510:string)  [unwired: 2 in]
                  n624 = Number To Fractional String(number=w1503, precision (6)=i16 3 ("width (-)")) -> (F-format string=w1506:string)  [unwired: 2 in]
                  n625 = Divide(x=w1501, y=w1494) -> (x/y=w1502:dbl)
                  n626 = To Unsigned Quad Integer(1:w1500) -> (0:w1499:u64)
                  n627 = Build Array(w1508, w1510, w1506) -> (w1509:string[])
                  n628 = call "Unix Time to Timestamp.vi"("Fractional Second"=w1502, "Unix Time (s)"=w1499) -> ("Timestamp"=w1498:timestamp)  [unwired: 8 in, 1 out]
                  n629 = To Double Precision Float(number=w1498) -> (double precision float=w1493:dbl)
                }
                n630 = Concatenate Strings(w1452, "TimeStamp;MeasureCh_X(g);INC_Y(Deg)", "\n") -> (w1468:string)
                n631 = call <vilib>:"Get System Directory.vi"("system directory type"=w1459) -> ("system directory"=w1469:path)  [unwired: 10 in]
                n632 = Concatenate Strings(w1475, "_" ("string"), "streaming.csv") -> (w1476:string)
                n633 = Build Path(base path=w1469, name or relative path="Logfile") -> (appended path=w1470:path)
                n634 = call <vilib>:"Check if File or Folder Exists.vi"("path"=w1470) -> ("file or folder exists?"=w1471:bool, "dup path"=w1472:path)  [unwired: 8 in, 1 out]
                n635 = case shown="False" w1471 {
                  tunnel: w1472 -> [w1491 w1492]
                  tunnel: [w1490 w1492] -> w1473
                  frame False {
                    n636 = Create Folder(path (use dialog)=w1491) -> (created path=w1490:path)  [unwired: 2 in, 2 out]
                  }
                  frame True {
                  }
                }
                n637 = Build Path(base path=w1473, name or relative path=w1476) -> (appended path=w1474:path)
                n638 = Open/Create/Replace File(file path (use dialog)=w1474, operation (0:open)=T10."open or create") -> (refnum out=w1467:refnum<file>, error out=w1465:errorcluster)  [unwired: 4 in, 1 out]
                n639 = Write to Text File(file (use dialog)=w1467, text=w1468, error in=w1465) -> (refnum out=w1466:refnum<file>, error out=w1464:errorcluster)  [unwired: 1 in, 1 out]
                n640 = Close File(refnum=w1466, error in=w1464) -> (path=w1454:path)  [unwired: 1 out]
              }
              frame 19 {
                w1519 = T13 2 items=["User Home"=0, "User Desktop"=1, "User Documents"=2, "User Application Data"=3, "User Preferences"=4, "User Temporary"=5, "Public Documents"=6, "Public Application Data"=7, "Public Preferences"=8, "Public Cache"=13, "System Core Libraries"=9, "System Installed Libraries"=10, "Application Files"=11, "Boot Volume Root"=12] ("system directory type")
                n641 = Search and Replace String(replace all?=TRUE ("replace all? (F)"), input string=w1514, search string="/") -> (result string=w1535:string)  [unwired: 5 in, 3 out]
                n642 = Concatenate Strings(w1512, "TimeStamp;MeasureCh_Z(g);Ch_X(g);INC_Y(Deg)", "\n") -> (w1528:string)
                n643 = call <vilib>:"Get System Directory.vi"("system directory type"=w1519) -> ("system directory"=w1529:path)  [unwired: 10 in]
                n644 = Concatenate Strings(w1535, "_" ("string"), "streaming.csv") -> (w1536:string)
                n645 = Build Path(base path=w1529, name or relative path="Logfile") -> (appended path=w1530:path)
                n646 = call <vilib>:"Check if File or Folder Exists.vi"("path"=w1530) -> ("file or folder exists?"=w1531:bool, "dup path"=w1532:path)  [unwired: 8 in, 1 out]
                n647 = case shown="False" w1531 {
                  tunnel: w1532 -> [w1555 w1556]
                  tunnel: [w1554 w1556] -> w1533
                  frame False {
                    n648 = Create Folder(path (use dialog)=w1555) -> (created path=w1554:path)  [unwired: 2 in, 2 out]
                  }
                  frame True {
                  }
                }
                n649 = Decimate 1D Array(w1552) -> (w1548:dbl[], w1547:dbl[], w1550:dbl[])
                n650 = for {
                  tunnel: [w1576] -> w1549 mode=indexing
                  tunnel: w1551 -> [w1570] mode=indexing
                  tunnel: w1548 -> [w1569] mode=indexing
                  tunnel: w1547 -> [w1568] mode=indexing
                  tunnel: w1550 -> [w1567] mode=indexing
                  tunnel: [w1569] -> w1546 mode=indexing
                  tunnel: [w1568] -> w1545 mode=indexing
                  tunnel: [w1567] -> w1544 mode=indexing
                  tunnel: w1543 -> [w1561]
                  tunnel: w1542 -> [w1560]
                  tunnel: w1541 -> [w1559] mode=indexing
                  tunnel: w1540 -> [w1558]
                  tunnel: [w1557] -> w1539
                  tunnel: [w1557] -> w1538
                  tunnel: [w1557] -> w1537
                  n651 = Join Numbers(hi=w1561, lo=w1560) -> ((hi.lo)=w1564:u32)
                  n652 = To Double Precision Float(number=w1559) -> (double precision float=w1565:dbl)
                  n653 = Number To Decimal String(number=w1570) -> (decimal integer string=w1575:string)  [unwired: 1 in]
                  n654 = Number To Fractional String(number=w1569, precision (6)=i16 3 ("width (-)")) -> (F-format string=w1577:string)  [unwired: 2 in]
                  n655 = Number To Fractional String(number=w1568, precision (6)=i16 3 ("width (-)")) -> (F-format string=w1573:string)  [unwired: 2 in]
                  n656 = Number To Fractional String(number=w1567, precision (6)=i16 3 ("width (-)")) -> (F-format string=w1571:string)  [unwired: 2 in]
                  n657 = Divide(x=w1565, y=w1558) -> (x/y=w1566:dbl)
                  n658 = To Unsigned Quad Integer(1:w1564) -> (0:w1563:u64)
                  n659 = Build Array(w1575, w1577, w1573, w1571) -> (w1576:string[])
                  n660 = call "Unix Time to Timestamp.vi"("Fractional Second"=w1566, "Unix Time (s)"=w1563) -> ("Timestamp"=w1562:timestamp)  [unwired: 8 in, 1 out]
                  n661 = To Double Precision Float(number=w1562) -> (double precision float=w1557:dbl)
                }
                n662 = Build Path(base path=w1533, name or relative path=w1536) -> (appended path=w1534:path)
                n663 = Open/Create/Replace File(file path (use dialog)=w1534, operation (0:open)=T10."open or create") -> (refnum out=w1527:refnum<file>, error out=w1525:errorcluster)  [unwired: 4 in, 1 out]
                n664 = Write to Text File(file (use dialog)=w1527, text=w1528, error in=w1525) -> (refnum out=w1526:refnum<file>, error out=w1524:errorcluster)  [unwired: 1 in, 1 out]
                n665 = Close File(refnum=w1526, error in=w1524) -> (path=w1513:path)  [unwired: 1 out]
              }
              frame 20 {
                w1586 = T13 2 items=["User Home"=0, "User Desktop"=1, "User Documents"=2, "User Application Data"=3, "User Preferences"=4, "User Temporary"=5, "Public Documents"=6, "Public Application Data"=7, "Public Preferences"=8, "Public Cache"=13, "System Core Libraries"=9, "System Installed Libraries"=10, "Application Files"=11, "Boot Volume Root"=12] ("system directory type")
                n666 = Decimate 1D Array(w1615) -> (w1611:dbl[], w1613:dbl[])
                n667 = Search and Replace String(replace all?=TRUE ("replace all? (F)"), input string=w1580, search string="/") -> (result string=w1602:string)  [unwired: 5 in, 3 out]
                n668 = for {
                  tunnel: [w1636] -> w1612 mode=indexing
                  tunnel: w1614 -> [w1632] mode=indexing
                  tunnel: w1611 -> [w1631] mode=indexing
                  tunnel: w1613 -> [w1630] mode=indexing
                  tunnel: [w1631] -> w1610 mode=indexing
                  tunnel: [w1630] -> w1609 mode=indexing
                  tunnel: w1608 -> [w1624]
                  tunnel: w1607 -> [w1623]
                  tunnel: w1606 -> [w1622] mode=indexing
                  tunnel: w1605 -> [w1621]
                  tunnel: [w1620] -> w1604
                  n669 = Join Numbers(hi=w1624, lo=w1623) -> ((hi.lo)=w1627:u32)
                  n670 = To Double Precision Float(number=w1622) -> (double precision float=w1628:dbl)
                  n671 = Number To Decimal String(number=w1632) -> (decimal integer string=w1635:string)  [unwired: 1 in]
                  n672 = Number To Fractional String(number=w1631, precision (6)=i16 3 ("width (-)")) -> (F-format string=w1637:string)  [unwired: 2 in]
                  n673 = Number To Fractional String(number=w1630, precision (6)=i16 3 ("width (-)")) -> (F-format string=w1633:string)  [unwired: 2 in]
                  n674 = Divide(x=w1628, y=w1621) -> (x/y=w1629:dbl)
                  n675 = To Unsigned Quad Integer(1:w1627) -> (0:w1626:u64)
                  n676 = Build Array(w1635, w1637, w1633) -> (w1636:string[])
                  n677 = call "Unix Time to Timestamp.vi"("Fractional Second"=w1629, "Unix Time (s)"=w1626) -> ("Timestamp"=w1625:timestamp)  [unwired: 8 in, 1 out]
                  n678 = To Double Precision Float(number=w1625) -> (double precision float=w1620:dbl)
                }
                n679 = Concatenate Strings(w1579, "TimeStamp;MeasureCh_Y(g);INC_Y(Deg)", "\n") -> (w1595:string)
                n680 = call <vilib>:"Get System Directory.vi"("system directory type"=w1586) -> ("system directory"=w1596:path)  [unwired: 10 in]
                n681 = Concatenate Strings(w1602, "_" ("string"), "streaming.csv") -> (w1603:string)
                n682 = Build Path(base path=w1596, name or relative path="Logfile") -> (appended path=w1597:path)
                n683 = call <vilib>:"Check if File or Folder Exists.vi"("path"=w1597) -> ("file or folder exists?"=w1598:bool, "dup path"=w1599:path)  [unwired: 8 in, 1 out]
                n684 = case shown="False" w1598 {
                  tunnel: w1599 -> [w1618 w1619]
                  tunnel: [w1617 w1619] -> w1600
                  frame False {
                    n685 = Create Folder(path (use dialog)=w1618) -> (created path=w1617:path)  [unwired: 2 in, 2 out]
                  }
                  frame True {
                  }
                }
                n686 = Build Path(base path=w1600, name or relative path=w1603) -> (appended path=w1601:path)
                n687 = Open/Create/Replace File(file path (use dialog)=w1601, operation (0:open)=T10."open or create") -> (refnum out=w1594:refnum<file>, error out=w1592:errorcluster)  [unwired: 4 in, 1 out]
                n688 = Write to Text File(file (use dialog)=w1594, text=w1595, error in=w1592) -> (refnum out=w1593:refnum<file>, error out=w1591:errorcluster)  [unwired: 1 in, 1 out]
                n689 = Close File(refnum=w1593, error in=w1591) -> (path=w1581:path)  [unwired: 1 out]
              }
              frame 21 {
                w1646 = T13 2 items=["User Home"=0, "User Desktop"=1, "User Documents"=2, "User Application Data"=3, "User Preferences"=4, "User Temporary"=5, "Public Documents"=6, "Public Application Data"=7, "Public Preferences"=8, "Public Cache"=13, "System Core Libraries"=9, "System Installed Libraries"=10, "Application Files"=11, "Boot Volume Root"=12] ("system directory type")
                n690 = Search and Replace String(replace all?=TRUE ("replace all? (F)"), input string=w1641, search string="/") -> (result string=w1662:string)  [unwired: 5 in, 3 out]
                n691 = Concatenate Strings(w1639, "TimeStamp;MeasureCh_Z(g);Ch_Y(g);INC_Y(Deg)", "\n") -> (w1655:string)
                n692 = call <vilib>:"Get System Directory.vi"("system directory type"=w1646) -> ("system directory"=w1656:path)  [unwired: 10 in]
                n693 = Concatenate Strings(w1662, "_" ("string"), "streaming.csv") -> (w1663:string)
                n694 = Build Path(base path=w1656, name or relative path="Logfile") -> (appended path=w1657:path)
                n695 = call <vilib>:"Check if File or Folder Exists.vi"("path"=w1657) -> ("file or folder exists?"=w1658:bool, "dup path"=w1659:path)  [unwired: 8 in, 1 out]
                n696 = case shown="False" w1658 {
                  tunnel: w1659 -> [w1682 w1683]
                  tunnel: [w1681 w1683] -> w1660
                  frame False {
                    n697 = Create Folder(path (use dialog)=w1682) -> (created path=w1681:path)  [unwired: 2 in, 2 out]
                  }
                  frame True {
                  }
                }
                n698 = Decimate 1D Array(w1679) -> (w1675:dbl[], w1674:dbl[], w1677:dbl[])
                n699 = for {
                  tunnel: [w1703] -> w1676 mode=indexing
                  tunnel: w1678 -> [w1697] mode=indexing
                  tunnel: w1675 -> [w1696] mode=indexing
                  tunnel: w1674 -> [w1695] mode=indexing
                  tunnel: w1677 -> [w1694] mode=indexing
                  tunnel: [w1696] -> w1673 mode=indexing
                  tunnel: [w1695] -> w1672 mode=indexing
                  tunnel: [w1694] -> w1671 mode=indexing
                  tunnel: w1670 -> [w1688]
                  tunnel: w1669 -> [w1687]
                  tunnel: w1668 -> [w1686] mode=indexing
                  tunnel: w1667 -> [w1685]
                  tunnel: [w1684] -> w1666
                  tunnel: [w1684] -> w1665
                  tunnel: [w1684] -> w1664
                  n700 = Join Numbers(hi=w1688, lo=w1687) -> ((hi.lo)=w1691:u32)
                  n701 = To Double Precision Float(number=w1686) -> (double precision float=w1692:dbl)
                  n702 = Number To Decimal String(number=w1697) -> (decimal integer string=w1702:string)  [unwired: 1 in]
                  n703 = Number To Fractional String(number=w1696, precision (6)=i16 3 ("width (-)")) -> (F-format string=w1704:string)  [unwired: 2 in]
                  n704 = Number To Fractional String(number=w1695, precision (6)=i16 3 ("width (-)")) -> (F-format string=w1700:string)  [unwired: 2 in]
                  n705 = Number To Fractional String(number=w1694, precision (6)=i16 3 ("width (-)")) -> (F-format string=w1698:string)  [unwired: 2 in]
                  n706 = Divide(x=w1692, y=w1685) -> (x/y=w1693:dbl)
                  n707 = To Unsigned Quad Integer(1:w1691) -> (0:w1690:u64)
                  n708 = Build Array(w1702, w1704, w1700, w1698) -> (w1703:string[])
                  n709 = call "Unix Time to Timestamp.vi"("Fractional Second"=w1693, "Unix Time (s)"=w1690) -> ("Timestamp"=w1689:timestamp)  [unwired: 8 in, 1 out]
                  n710 = To Double Precision Float(number=w1689) -> (double precision float=w1684:dbl)
                }
                n711 = Build Path(base path=w1660, name or relative path=w1663) -> (appended path=w1661:path)
                n712 = Open/Create/Replace File(file path (use dialog)=w1661, operation (0:open)=T10."open or create") -> (refnum out=w1654:refnum<file>, error out=w1652:errorcluster)  [unwired: 4 in, 1 out]
                n713 = Write to Text File(file (use dialog)=w1654, text=w1655, error in=w1652) -> (refnum out=w1653:refnum<file>, error out=w1651:errorcluster)  [unwired: 1 in, 1 out]
                n714 = Close File(refnum=w1653, error in=w1651) -> (path=w1640:path)  [unwired: 1 out]
              }
              frame 22 {
                w1713 = T13 2 items=["User Home"=0, "User Desktop"=1, "User Documents"=2, "User Application Data"=3, "User Preferences"=4, "User Temporary"=5, "Public Documents"=6, "Public Application Data"=7, "Public Preferences"=8, "Public Cache"=13, "System Core Libraries"=9, "System Installed Libraries"=10, "Application Files"=11, "Boot Volume Root"=12] ("system directory type")
                n715 = Search and Replace String(replace all?=TRUE ("replace all? (F)"), input string=w1708, search string="/") -> (result string=w1729:string)  [unwired: 5 in, 3 out]
                n716 = Concatenate Strings(w1706, "TimeStamp;MeasureCh_X(g);Ch_Y(g);INC_X(Deg)", "\n") -> (w1722:string)
                n717 = call <vilib>:"Get System Directory.vi"("system directory type"=w1713) -> ("system directory"=w1723:path)  [unwired: 10 in]
                n718 = Concatenate Strings(w1729, "_" ("string"), "streaming.csv") -> (w1730:string)
                n719 = Build Path(base path=w1723, name or relative path="Logfile") -> (appended path=w1724:path)
                n720 = call <vilib>:"Check if File or Folder Exists.vi"("path"=w1724) -> ("file or folder exists?"=w1725:bool, "dup path"=w1726:path)  [unwired: 8 in, 1 out]
                n721 = case shown="False" w1725 {
                  tunnel: w1726 -> [w1749 w1750]
                  tunnel: [w1748 w1750] -> w1727
                  frame False {
                    n722 = Create Folder(path (use dialog)=w1749) -> (created path=w1748:path)  [unwired: 2 in, 2 out]
                  }
                  frame True {
                  }
                }
                n723 = Decimate 1D Array(w1746) -> (w1742:dbl[], w1741:dbl[], w1745:dbl[])
                n724 = for {
                  tunnel: [w1770] -> w1743 mode=indexing
                  tunnel: w1744 -> [w1764] mode=indexing
                  tunnel: w1742 -> [w1763] mode=indexing
                  tunnel: w1741 -> [w1762] mode=indexing
                  tunnel: w1745 -> [w1761] mode=indexing
                  tunnel: [w1763] -> w1740 mode=indexing
                  tunnel: [w1762] -> w1739 mode=indexing
                  tunnel: [w1761] -> w1738 mode=indexing
                  tunnel: w1737 -> [w1755]
                  tunnel: w1736 -> [w1754]
                  tunnel: w1735 -> [w1753] mode=indexing
                  tunnel: w1734 -> [w1752]
                  tunnel: [w1751] -> w1733
                  tunnel: [w1751] -> w1732
                  tunnel: [w1751] -> w1731
                  n725 = Join Numbers(hi=w1755, lo=w1754) -> ((hi.lo)=w1758:u32)
                  n726 = To Double Precision Float(number=w1753) -> (double precision float=w1759:dbl)
                  n727 = Number To Decimal String(number=w1764) -> (decimal integer string=w1769:string)  [unwired: 1 in]
                  n728 = Number To Fractional String(number=w1763, precision (6)=i16 3 ("width (-)")) -> (F-format string=w1771:string)  [unwired: 2 in]
                  n729 = Number To Fractional String(number=w1762, precision (6)=i16 3 ("width (-)")) -> (F-format string=w1767:string)  [unwired: 2 in]
                  n730 = Number To Fractional String(number=w1761, precision (6)=i16 3 ("width (-)")) -> (F-format string=w1765:string)  [unwired: 2 in]
                  n731 = Divide(x=w1759, y=w1752) -> (x/y=w1760:dbl)
                  n732 = To Unsigned Quad Integer(1:w1758) -> (0:w1757:u64)
                  n733 = Build Array(w1769, w1771, w1767, w1765) -> (w1770:string[])
                  n734 = call "Unix Time to Timestamp.vi"("Fractional Second"=w1760, "Unix Time (s)"=w1757) -> ("Timestamp"=w1756:timestamp)  [unwired: 8 in, 1 out]
                  n735 = To Double Precision Float(number=w1756) -> (double precision float=w1751:dbl)
                }
                n736 = Build Path(base path=w1727, name or relative path=w1730) -> (appended path=w1728:path)
                n737 = Open/Create/Replace File(file path (use dialog)=w1728, operation (0:open)=T10."open or create") -> (refnum out=w1721:refnum<file>, error out=w1719:errorcluster)  [unwired: 4 in, 1 out]
                n738 = Write to Text File(file (use dialog)=w1721, text=w1722, error in=w1719) -> (refnum out=w1720:refnum<file>, error out=w1718:errorcluster)  [unwired: 1 in, 1 out]
                n739 = Close File(refnum=w1720, error in=w1718) -> (path=w1707:path)  [unwired: 1 out]
              }
              frame 23 {
                w1780 = T13 2 items=["User Home"=0, "User Desktop"=1, "User Documents"=2, "User Application Data"=3, "User Preferences"=4, "User Temporary"=5, "Public Documents"=6, "Public Application Data"=7, "Public Preferences"=8, "Public Cache"=13, "System Core Libraries"=9, "System Installed Libraries"=10, "Application Files"=11, "Boot Volume Root"=12] ("system directory type")
                n740 = Search and Replace String(replace all?=TRUE ("replace all? (F)"), input string=w1774, search string="/") -> (result string=w1796:string)  [unwired: 5 in, 3 out]
                n741 = Concatenate Strings(w1773, "TimeStamp;MeasureCh_Z(g);Ch_X(g);Ch_Y(g);INC_Y(Deg)", "\n") -> (w1789:string)
                n742 = call <vilib>:"Get System Directory.vi"("system directory type"=w1780) -> ("system directory"=w1790:path)  [unwired: 10 in]
                n743 = Concatenate Strings(w1796, "_" ("string"), "streaming.csv") -> (w1797:string)
                n744 = Build Path(base path=w1790, name or relative path="Logfile") -> (appended path=w1791:path)
                n745 = call <vilib>:"Check if File or Folder Exists.vi"("path"=w1791) -> ("file or folder exists?"=w1792:bool, "dup path"=w1793:path)  [unwired: 8 in, 1 out]
                n746 = Decimate 1D Array(w1813) -> (w1812:dbl[], w1811:dbl[], w1810:dbl[], w1807:dbl[])
                n747 = case shown="False" w1792 {
                  tunnel: w1793 -> [w1816 w1817]
                  tunnel: [w1815 w1817] -> w1794
                  frame False {
                    n748 = Create Folder(path (use dialog)=w1816) -> (created path=w1815:path)  [unwired: 2 in, 2 out]
                  }
                  frame True {
                  }
                }
                n749 = for {
                  tunnel: [w1839] -> w1808 mode=indexing
                  tunnel: w1809 -> [w1833] mode=indexing
                  tunnel: w1812 -> [w1831] mode=indexing
                  tunnel: w1811 -> [w1830] mode=indexing
                  tunnel: w1810 -> [w1829] mode=indexing
                  tunnel: w1807 -> [w1828] mode=indexing
                  tunnel: [w1831] -> w1806 mode=indexing
                  tunnel: [w1830] -> w1805 mode=indexing
                  tunnel: [w1829] -> w1804 mode=indexing
                  tunnel: [w1828] -> w1803 mode=indexing
                  tunnel: w1802 -> [w1822]
                  tunnel: w1801 -> [w1821]
                  tunnel: w1800 -> [w1820] mode=indexing
                  tunnel: w1799 -> [w1819]
                  tunnel: [w1818] -> w1798
                  n750 = Number To Fractional String(number=w1828, precision (6)=i16 3 ("width (-)")) -> ()  [unwired: 2 in, 1 out]
                  n751 = Join Numbers(hi=w1822, lo=w1821) -> ((hi.lo)=w1825:u32)
                  n752 = To Double Precision Float(number=w1820) -> (double precision float=w1826:dbl)
                  n753 = Number To Decimal String(number=w1833) -> (decimal integer string=w1838:string)  [unwired: 1 in]
                  n754 = Number To Fractional String(number=w1831, precision (6)=i16 3 ("width (-)")) -> (F-format string=w1840:string)  [unwired: 2 in]
                  n755 = Number To Fractional String(number=w1830, precision (6)=i16 3 ("width (-)")) -> (F-format string=w1836:string)  [unwired: 2 in]
                  n756 = Number To Fractional String(number=w1829, precision (6)=i16 3 ("width (-)")) -> (F-format string=w1834:string)  [unwired: 2 in]
                  n757 = Divide(x=w1826, y=w1819) -> (x/y=w1827:dbl)
                  n758 = To Unsigned Quad Integer(1:w1825) -> (0:w1824:u64)
                  n759 = Build Array(w1838, w1840, w1836, w1834) -> (w1839:string[])
                  n760 = call "Unix Time to Timestamp.vi"("Fractional Second"=w1827, "Unix Time (s)"=w1824) -> ("Timestamp"=w1823:timestamp)  [unwired: 8 in, 1 out]
                  n761 = To Double Precision Float(number=w1823) -> (double precision float=w1818:dbl)
                }
                n762 = Build Path(base path=w1794, name or relative path=w1797) -> (appended path=w1795:path)
                n763 = Open/Create/Replace File(file path (use dialog)=w1795, operation (0:open)=T10."open or create") -> (refnum out=w1788:refnum<file>, error out=w1786:errorcluster)  [unwired: 4 in, 1 out]
                n764 = Write to Text File(file (use dialog)=w1788, text=w1789, error in=w1786) -> (refnum out=w1787:refnum<file>, error out=w1785:errorcluster)  [unwired: 1 in, 1 out]
                n765 = Close File(refnum=w1787, error in=w1785) -> (path=w1775:path)  [unwired: 1 out]
              }
              frame 24 {
                w1849 = T13 2 items=["User Home"=0, "User Desktop"=1, "User Documents"=2, "User Application Data"=3, "User Preferences"=4, "User Temporary"=5, "Public Documents"=6, "Public Application Data"=7, "Public Preferences"=8, "Public Cache"=13, "System Core Libraries"=9, "System Installed Libraries"=10, "Application Files"=11, "Boot Volume Root"=12] ("system directory type")
                n766 = Decimate 1D Array(w1878) -> (w1876:dbl[], w1875:dbl[])
                n767 = Search and Replace String(replace all?=TRUE ("replace all? (F)"), input string=w1844, search string="/") -> (result string=w1865:string)  [unwired: 5 in, 3 out]
                n768 = Concatenate Strings(w1842, "TimeStamp;Measure INC_X(Deg);INC_Y(Deg)", "\n") -> (w1858:string)
                n769 = for {
                  tunnel: [w1899] -> w1874 mode=indexing
                  tunnel: w1877 -> [w1895] mode=indexing
                  tunnel: w1876 -> [w1894] mode=indexing
                  tunnel: w1875 -> [w1893] mode=indexing
                  tunnel: [w1894] -> w1873 mode=indexing
                  tunnel: [w1893] -> w1872 mode=indexing
                  tunnel: w1871 -> [w1887]
                  tunnel: w1870 -> [w1886]
                  tunnel: w1869 -> [w1885] mode=indexing
                  tunnel: w1868 -> [w1884]
                  tunnel: [w1883] -> w1867
                  n770 = Join Numbers(hi=w1887, lo=w1886) -> ((hi.lo)=w1890:u32)
                  n771 = To Double Precision Float(number=w1885) -> (double precision float=w1891:dbl)
                  n772 = Number To Decimal String(number=w1895) -> (decimal integer string=w1898:string)  [unwired: 1 in]
                  n773 = Number To Fractional String(number=w1894, precision (6)=i16 3 ("width (-)")) -> (F-format string=w1900:string)  [unwired: 2 in]
                  n774 = Number To Fractional String(number=w1893, precision (6)=i16 3 ("width (-)")) -> (F-format string=w1896:string)  [unwired: 2 in]
                  n775 = Divide(x=w1891, y=w1884) -> (x/y=w1892:dbl)
                  n776 = To Unsigned Quad Integer(1:w1890) -> (0:w1889:u64)
                  n777 = Build Array(w1898, w1900, w1896) -> (w1899:string[])
                  n778 = call "Unix Time to Timestamp.vi"("Fractional Second"=w1892, "Unix Time (s)"=w1889) -> ("Timestamp"=w1888:timestamp)  [unwired: 8 in, 1 out]
                  n779 = To Double Precision Float(number=w1888) -> (double precision float=w1883:dbl)
                }
                n780 = call <vilib>:"Get System Directory.vi"("system directory type"=w1849) -> ("system directory"=w1859:path)  [unwired: 10 in]
                n781 = Concatenate Strings(w1865, "_" ("string"), "streaming.csv") -> (w1866:string)
                n782 = Build Path(base path=w1859, name or relative path="Logfile") -> (appended path=w1860:path)
                n783 = call <vilib>:"Check if File or Folder Exists.vi"("path"=w1860) -> ("file or folder exists?"=w1861:bool, "dup path"=w1862:path)  [unwired: 8 in, 1 out]
                n784 = case shown="False" w1861 {
                  tunnel: w1862 -> [w1881 w1882]
                  tunnel: [w1880 w1882] -> w1863
                  frame False {
                    n785 = Create Folder(path (use dialog)=w1881) -> (created path=w1880:path)  [unwired: 2 in, 2 out]
                  }
                  frame True {
                  }
                }
                n786 = Build Path(base path=w1863, name or relative path=w1866) -> (appended path=w1864:path)
                n787 = Open/Create/Replace File(file path (use dialog)=w1864, operation (0:open)=T10."open or create") -> (refnum out=w1857:refnum<file>, error out=w1855:errorcluster)  [unwired: 4 in, 1 out]
                n788 = Write to Text File(file (use dialog)=w1857, text=w1858, error in=w1855) -> (refnum out=w1856:refnum<file>, error out=w1854:errorcluster)  [unwired: 1 in, 1 out]
                n789 = Close File(refnum=w1856, error in=w1854) -> (path=w1843:path)  [unwired: 1 out]
              }
              frame 25 {
                w1909 = T13 2 items=["User Home"=0, "User Desktop"=1, "User Documents"=2, "User Application Data"=3, "User Preferences"=4, "User Temporary"=5, "Public Documents"=6, "Public Application Data"=7, "Public Preferences"=8, "Public Cache"=13, "System Core Libraries"=9, "System Installed Libraries"=10, "Application Files"=11, "Boot Volume Root"=12] ("system directory type")
                n790 = Search and Replace String(replace all?=TRUE ("replace all? (F)"), input string=w1904, search string="/") -> (result string=w1925:string)  [unwired: 5 in, 3 out]
                n791 = Concatenate Strings(w1902, "TimeStamp;Measure Ch_Z(g);INC_X(Deg);INC_Y(Deg)", "\n") -> (w1918:string)
                n792 = call <vilib>:"Get System Directory.vi"("system directory type"=w1909) -> ("system directory"=w1919:path)  [unwired: 10 in]
                n793 = Concatenate Strings(w1925, "_" ("string"), "streaming.csv") -> (w1926:string)
                n794 = Build Path(base path=w1919, name or relative path="Logfile") -> (appended path=w1920:path)
                n795 = call <vilib>:"Check if File or Folder Exists.vi"("path"=w1920) -> ("file or folder exists?"=w1921:bool, "dup path"=w1922:path)  [unwired: 8 in, 1 out]
                n796 = case shown="False" w1921 {
                  tunnel: w1922 -> [w1943 w1944]
                  tunnel: [w1942 w1944] -> w1923
                  frame False {
                    n797 = Create Folder(path (use dialog)=w1943) -> (created path=w1942:path)  [unwired: 2 in, 2 out]
                  }
                  frame True {
                  }
                }
                n798 = Decimate 1D Array(w1940) -> (w1935:dbl[], w1938:dbl[], w1937:dbl[])
                n799 = for {
                  tunnel: [w1964] -> w1936 mode=indexing
                  tunnel: w1939 -> [w1958] mode=indexing
                  tunnel: w1935 -> [w1957] mode=indexing
                  tunnel: w1938 -> [w1956] mode=indexing
                  tunnel: w1937 -> [w1955] mode=indexing
                  tunnel: [w1957] -> w1934 mode=indexing
                  tunnel: [w1956] -> w1933 mode=indexing
                  tunnel: [w1955] -> w1932 mode=indexing
                  tunnel: w1931 -> [w1949]
                  tunnel: w1930 -> [w1948]
                  tunnel: w1929 -> [w1947] mode=indexing
                  tunnel: w1928 -> [w1946]
                  tunnel: [w1945] -> w1927
                  n800 = Join Numbers(hi=w1949, lo=w1948) -> ((hi.lo)=w1952:u32)
                  n801 = To Double Precision Float(number=w1947) -> (double precision float=w1953:dbl)
                  n802 = Number To Decimal String(number=w1958) -> (decimal integer string=w1963:string)  [unwired: 1 in]
                  n803 = Number To Fractional String(number=w1957, precision (6)=i16 3 ("width (-)")) -> (F-format string=w1965:string)  [unwired: 2 in]
                  n804 = Number To Fractional String(number=w1956, precision (6)=i16 3 ("width (-)")) -> (F-format string=w1961:string)  [unwired: 2 in]
                  n805 = Number To Fractional String(number=w1955, precision (6)=i16 3 ("width (-)")) -> (F-format string=w1959:string)  [unwired: 2 in]
                  n806 = Divide(x=w1953, y=w1946) -> (x/y=w1954:dbl)
                  n807 = To Unsigned Quad Integer(1:w1952) -> (0:w1951:u64)
                  n808 = Build Array(w1963, w1965, w1961, w1959) -> (w1964:string[])
                  n809 = call "Unix Time to Timestamp.vi"("Fractional Second"=w1954, "Unix Time (s)"=w1951) -> ("Timestamp"=w1950:timestamp)  [unwired: 8 in, 1 out]
                  n810 = To Double Precision Float(number=w1950) -> (double precision float=w1945:dbl)
                }
                n811 = Build Path(base path=w1923, name or relative path=w1926) -> (appended path=w1924:path)
                n812 = Open/Create/Replace File(file path (use dialog)=w1924, operation (0:open)=T10."open or create") -> (refnum out=w1917:refnum<file>, error out=w1915:errorcluster)  [unwired: 4 in, 1 out]
                n813 = Write to Text File(file (use dialog)=w1917, text=w1918, error in=w1915) -> (refnum out=w1916:refnum<file>, error out=w1914:errorcluster)  [unwired: 1 in, 1 out]
                n814 = Close File(refnum=w1916, error in=w1914) -> (path=w1903:path)  [unwired: 1 out]
              }
              frame 26 {
                w1974 = T13 2 items=["User Home"=0, "User Desktop"=1, "User Documents"=2, "User Application Data"=3, "User Preferences"=4, "User Temporary"=5, "Public Documents"=6, "Public Application Data"=7, "Public Preferences"=8, "Public Cache"=13, "System Core Libraries"=9, "System Installed Libraries"=10, "Application Files"=11, "Boot Volume Root"=12] ("system directory type")
                n815 = Search and Replace String(replace all?=TRUE ("replace all? (F)"), input string=w1969, search string="/") -> (result string=w1990:string)  [unwired: 5 in, 3 out]
                n816 = Concatenate Strings(w1967, "TimeStamp;Measure Ch_X(g);INC_X(Deg);INC_Y(Deg)", "\n") -> (w1983:string)
                n817 = call <vilib>:"Get System Directory.vi"("system directory type"=w1974) -> ("system directory"=w1984:path)  [unwired: 10 in]
                n818 = Concatenate Strings(w1990, "_" ("string"), "streaming.csv") -> (w1991:string)
                n819 = Build Path(base path=w1984, name or relative path="Logfile") -> (appended path=w1985:path)
                n820 = call <vilib>:"Check if File or Folder Exists.vi"("path"=w1985) -> ("file or folder exists?"=w1986:bool, "dup path"=w1987:path)  [unwired: 8 in, 1 out]
                n821 = case shown="False" w1986 {
                  tunnel: w1987 -> [w2008 w2009]
                  tunnel: [w2007 w2009] -> w1988
                  frame False {
                    n822 = Create Folder(path (use dialog)=w2008) -> (created path=w2007:path)  [unwired: 2 in, 2 out]
                  }
                  frame True {
                  }
                }
                n823 = Decimate 1D Array(w2005) -> (w2000:dbl[], w2004:dbl[], w2003:dbl[])
                n824 = for {
                  tunnel: [w2029] -> w2001 mode=indexing
                  tunnel: w2002 -> [w2023] mode=indexing
                  tunnel: w2000 -> [w2022] mode=indexing
                  tunnel: w2004 -> [w2021] mode=indexing
                  tunnel: w2003 -> [w2020] mode=indexing
                  tunnel: [w2022] -> w1999 mode=indexing
                  tunnel: [w2021] -> w1998 mode=indexing
                  tunnel: [w2020] -> w1997 mode=indexing
                  tunnel: w1996 -> [w2014]
                  tunnel: w1995 -> [w2013]
                  tunnel: w1994 -> [w2012] mode=indexing
                  tunnel: w1993 -> [w2011]
                  tunnel: [w2010] -> w1992
                  n825 = Join Numbers(hi=w2014, lo=w2013) -> ((hi.lo)=w2017:u32)
                  n826 = To Double Precision Float(number=w2012) -> (double precision float=w2018:dbl)
                  n827 = Number To Decimal String(number=w2023) -> (decimal integer string=w2028:string)  [unwired: 1 in]
                  n828 = Number To Fractional String(number=w2022, precision (6)=i16 3 ("width (-)")) -> (F-format string=w2030:string)  [unwired: 2 in]
                  n829 = Number To Fractional String(number=w2021, precision (6)=i16 3 ("width (-)")) -> (F-format string=w2026:string)  [unwired: 2 in]
                  n830 = Number To Fractional String(number=w2020, precision (6)=i16 3 ("width (-)")) -> (F-format string=w2024:string)  [unwired: 2 in]
                  n831 = Divide(x=w2018, y=w2011) -> (x/y=w2019:dbl)
                  n832 = To Unsigned Quad Integer(1:w2017) -> (0:w2016:u64)
                  n833 = Build Array(w2028, w2030, w2026, w2024) -> (w2029:string[])
                  n834 = call "Unix Time to Timestamp.vi"("Fractional Second"=w2019, "Unix Time (s)"=w2016) -> ("Timestamp"=w2015:timestamp)  [unwired: 8 in, 1 out]
                  n835 = To Double Precision Float(number=w2015) -> (double precision float=w2010:dbl)
                }
                n836 = Build Path(base path=w1988, name or relative path=w1991) -> (appended path=w1989:path)
                n837 = Open/Create/Replace File(file path (use dialog)=w1989, operation (0:open)=T10."open or create") -> (refnum out=w1982:refnum<file>, error out=w1980:errorcluster)  [unwired: 4 in, 1 out]
                n838 = Write to Text File(file (use dialog)=w1982, text=w1983, error in=w1980) -> (refnum out=w1981:refnum<file>, error out=w1979:errorcluster)  [unwired: 1 in, 1 out]
                n839 = Close File(refnum=w1981, error in=w1979) -> (path=w1968:path)  [unwired: 1 out]
              }
              frame 27 {
                w2039 = T13 2 items=["User Home"=0, "User Desktop"=1, "User Documents"=2, "User Application Data"=3, "User Preferences"=4, "User Temporary"=5, "Public Documents"=6, "Public Application Data"=7, "Public Preferences"=8, "Public Cache"=13, "System Core Libraries"=9, "System Installed Libraries"=10, "Application Files"=11, "Boot Volume Root"=12] ("system directory type")
                n840 = Search and Replace String(replace all?=TRUE ("replace all? (F)"), input string=w2034, search string="/") -> (result string=w2055:string)  [unwired: 5 in, 3 out]
                n841 = Concatenate Strings(w2032, "TimeStamp;Measure Ch_Z(g);Ch_X(g);INC_X(Deg);INC_Y(Deg)", "\n") -> (w2048:string)
                n842 = call <vilib>:"Get System Directory.vi"("system directory type"=w2039) -> ("system directory"=w2049:path)  [unwired: 10 in]
                n843 = Concatenate Strings(w2055, "_" ("string"), "streaming.csv") -> (w2056:string)
                n844 = Build Path(base path=w2049, name or relative path="Logfile") -> (appended path=w2050:path)
                n845 = call <vilib>:"Check if File or Folder Exists.vi"("path"=w2050) -> ("file or folder exists?"=w2051:bool, "dup path"=w2052:path)  [unwired: 8 in, 1 out]
                n846 = case shown="False" w2051 {
                  tunnel: w2052 -> [w2075 w2076]
                  tunnel: [w2074 w2076] -> w2053
                  frame False {
                    n847 = Create Folder(path (use dialog)=w2075) -> (created path=w2074:path)  [unwired: 2 in, 2 out]
                  }
                  frame True {
                  }
                }
                n848 = Decimate 1D Array(w2072) -> (w2070:dbl[], w2069:dbl[], w2067:dbl[], w2066:dbl[])
                n849 = for {
                  tunnel: [w2099] -> w2071 mode=indexing
                  tunnel: w2068 -> [w2093] mode=indexing
                  tunnel: w2070 -> [w2090] mode=indexing
                  tunnel: w2069 -> [w2089] mode=indexing
                  tunnel: w2067 -> [w2088] mode=indexing
                  tunnel: w2066 -> [w2087] mode=indexing
                  tunnel: [w2090] -> w2065 mode=indexing
                  tunnel: [w2089] -> w2064 mode=indexing
                  tunnel: [w2088] -> w2063 mode=indexing
                  tunnel: [w2087] -> w2062 mode=indexing
                  tunnel: w2061 -> [w2081]
                  tunnel: w2060 -> [w2080]
                  tunnel: w2059 -> [w2079] mode=indexing
                  tunnel: w2058 -> [w2078]
                  tunnel: [w2077] -> w2057
                  n850 = Join Numbers(hi=w2081, lo=w2080) -> ((hi.lo)=w2084:u32)
                  n851 = To Double Precision Float(number=w2079) -> (double precision float=w2085:dbl)
                  n852 = Number To Decimal String(number=w2093) -> (decimal integer string=w2098:string)  [unwired: 1 in]
                  n853 = Number To Fractional String(number=w2090, precision (6)=i16 3 ("width (-)")) -> (F-format string=w2100:string)  [unwired: 2 in]
                  n854 = Number To Fractional String(number=w2089, precision (6)=i16 3 ("width (-)")) -> (F-format string=w2096:string)  [unwired: 2 in]
                  n855 = Number To Fractional String(number=w2088, precision (6)=i16 3 ("width (-)")) -> (F-format string=w2094:string)  [unwired: 2 in]
                  n856 = Number To Fractional String(number=w2087, precision (6)=i16 3 ("width (-)")) -> (F-format string=w2091:string)  [unwired: 2 in]
                  n857 = Divide(x=w2085, y=w2078) -> (x/y=w2086:dbl)
                  n858 = To Unsigned Quad Integer(1:w2084) -> (0:w2083:u64)
                  n859 = Build Array(w2098, w2100, w2096, w2094, w2091) -> (w2099:string[])
                  n860 = call "Unix Time to Timestamp.vi"("Fractional Second"=w2086, "Unix Time (s)"=w2083) -> ("Timestamp"=w2082:timestamp)  [unwired: 8 in, 1 out]
                  n861 = To Double Precision Float(number=w2082) -> (double precision float=w2077:dbl)
                }
                n862 = Build Path(base path=w2053, name or relative path=w2056) -> (appended path=w2054:path)
                n863 = Open/Create/Replace File(file path (use dialog)=w2054, operation (0:open)=T10."open or create") -> (refnum out=w2047:refnum<file>, error out=w2045:errorcluster)  [unwired: 4 in, 1 out]
                n864 = Write to Text File(file (use dialog)=w2047, text=w2048, error in=w2045) -> (refnum out=w2046:refnum<file>, error out=w2044:errorcluster)  [unwired: 1 in, 1 out]
                n865 = Close File(refnum=w2046, error in=w2044) -> (path=w2033:path)  [unwired: 1 out]
              }
              frame 28 {
                w2109 = T13 2 items=["User Home"=0, "User Desktop"=1, "User Documents"=2, "User Application Data"=3, "User Preferences"=4, "User Temporary"=5, "Public Documents"=6, "Public Application Data"=7, "Public Preferences"=8, "Public Cache"=13, "System Core Libraries"=9, "System Installed Libraries"=10, "Application Files"=11, "Boot Volume Root"=12] ("system directory type")
                n866 = Search and Replace String(replace all?=TRUE ("replace all? (F)"), input string=w2104, search string="/") -> (result string=w2125:string)  [unwired: 5 in, 3 out]
                n867 = Concatenate Strings(w2102, "TimeStamp;Measure Ch_Y(g);INC_X(Deg);INC_Y(Deg)", "\n") -> (w2118:string)
                n868 = call <vilib>:"Get System Directory.vi"("system directory type"=w2109) -> ("system directory"=w2119:path)  [unwired: 10 in]
                n869 = Concatenate Strings(w2125, "_" ("string"), "streaming.csv") -> (w2126:string)
                n870 = Build Path(base path=w2119, name or relative path="Logfile") -> (appended path=w2120:path)
                n871 = call <vilib>:"Check if File or Folder Exists.vi"("path"=w2120) -> ("file or folder exists?"=w2121:bool, "dup path"=w2122:path)  [unwired: 8 in, 1 out]
                n872 = case shown="False" w2121 {
                  tunnel: w2122 -> [w2143 w2144]
                  tunnel: [w2142 w2144] -> w2123
                  frame False {
                    n873 = Create Folder(path (use dialog)=w2143) -> (created path=w2142:path)  [unwired: 2 in, 2 out]
                  }
                  frame True {
                  }
                }
                n874 = Decimate 1D Array(w2140) -> (w2138:dbl[], w2137:dbl[], w2136:dbl[])
                n875 = for {
                  tunnel: [w2164] -> w2135 mode=indexing
                  tunnel: w2139 -> [w2158] mode=indexing
                  tunnel: w2138 -> [w2157] mode=indexing
                  tunnel: w2137 -> [w2156] mode=indexing
                  tunnel: w2136 -> [w2155] mode=indexing
                  tunnel: [w2157] -> w2134 mode=indexing
                  tunnel: [w2156] -> w2133 mode=indexing
                  tunnel: [w2155] -> w2132 mode=indexing
                  tunnel: w2131 -> [w2149]
                  tunnel: w2130 -> [w2148]
                  tunnel: w2129 -> [w2147] mode=indexing
                  tunnel: w2128 -> [w2146]
                  tunnel: [w2145] -> w2127
                  n876 = Join Numbers(hi=w2149, lo=w2148) -> ((hi.lo)=w2152:u32)
                  n877 = To Double Precision Float(number=w2147) -> (double precision float=w2153:dbl)
                  n878 = Number To Decimal String(number=w2158) -> (decimal integer string=w2163:string)  [unwired: 1 in]
                  n879 = Number To Fractional String(number=w2157, precision (6)=i16 3 ("width (-)")) -> (F-format string=w2165:string)  [unwired: 2 in]
                  n880 = Number To Fractional String(number=w2156, precision (6)=i16 3 ("width (-)")) -> (F-format string=w2161:string)  [unwired: 2 in]
                  n881 = Number To Fractional String(number=w2155, precision (6)=i16 3 ("width (-)")) -> (F-format string=w2159:string)  [unwired: 2 in]
                  n882 = Divide(x=w2153, y=w2146) -> (x/y=w2154:dbl)
                  n883 = To Unsigned Quad Integer(1:w2152) -> (0:w2151:u64)
                  n884 = Build Array(w2163, w2165, w2161, w2159) -> (w2164:string[])
                  n885 = call "Unix Time to Timestamp.vi"("Fractional Second"=w2154, "Unix Time (s)"=w2151) -> ("Timestamp"=w2150:timestamp)  [unwired: 8 in, 1 out]
                  n886 = To Double Precision Float(number=w2150) -> (double precision float=w2145:dbl)
                }
                n887 = Build Path(base path=w2123, name or relative path=w2126) -> (appended path=w2124:path)
                n888 = Open/Create/Replace File(file path (use dialog)=w2124, operation (0:open)=T10."open or create") -> (refnum out=w2117:refnum<file>, error out=w2115:errorcluster)  [unwired: 4 in, 1 out]
                n889 = Write to Text File(file (use dialog)=w2117, text=w2118, error in=w2115) -> (refnum out=w2116:refnum<file>, error out=w2114:errorcluster)  [unwired: 1 in, 1 out]
                n890 = Close File(refnum=w2116, error in=w2114) -> (path=w2103:path)  [unwired: 1 out]
              }
              frame 29 {
                w2174 = T13 2 items=["User Home"=0, "User Desktop"=1, "User Documents"=2, "User Application Data"=3, "User Preferences"=4, "User Temporary"=5, "Public Documents"=6, "Public Application Data"=7, "Public Preferences"=8, "Public Cache"=13, "System Core Libraries"=9, "System Installed Libraries"=10, "Application Files"=11, "Boot Volume Root"=12] ("system directory type")
                n891 = Search and Replace String(replace all?=TRUE ("replace all? (F)"), input string=w2169, search string="/") -> (result string=w2190:string)  [unwired: 5 in, 3 out]
                n892 = Concatenate Strings(w2167, "TimeStamp;Measure Ch_Z(g);Ch_Y(g);INC_X(Deg);INC_Y(Deg)", "\n") -> (w2183:string)
                n893 = call <vilib>:"Get System Directory.vi"("system directory type"=w2174) -> ("system directory"=w2184:path)  [unwired: 10 in]
                n894 = Concatenate Strings(w2190, "_" ("string"), "streaming.csv") -> (w2191:string)
                n895 = Build Path(base path=w2184, name or relative path="Logfile") -> (appended path=w2185:path)
                n896 = call <vilib>:"Check if File or Folder Exists.vi"("path"=w2185) -> ("file or folder exists?"=w2186:bool, "dup path"=w2187:path)  [unwired: 8 in, 1 out]
                n897 = case shown="False" w2186 {
                  tunnel: w2187 -> [w2210 w2211]
                  tunnel: [w2209 w2211] -> w2188
                  frame False {
                    n898 = Create Folder(path (use dialog)=w2210) -> (created path=w2209:path)  [unwired: 2 in, 2 out]
                  }
                  frame True {
                  }
                }
                n899 = Decimate 1D Array(w2207) -> (w2201:dbl[], w2205:dbl[], w2202:dbl[], w2203:dbl[])
                n900 = for {
                  tunnel: [w2234] -> w2204 mode=indexing
                  tunnel: w2206 -> [w2228] mode=indexing
                  tunnel: w2201 -> [w2225] mode=indexing
                  tunnel: w2205 -> [w2224] mode=indexing
                  tunnel: w2202 -> [w2223] mode=indexing
                  tunnel: w2203 -> [w2222] mode=indexing
                  tunnel: [w2225] -> w2200 mode=indexing
                  tunnel: [w2224] -> w2199 mode=indexing
                  tunnel: [w2223] -> w2198 mode=indexing
                  tunnel: [w2222] -> w2197 mode=indexing
                  tunnel: w2196 -> [w2216]
                  tunnel: w2195 -> [w2215]
                  tunnel: w2194 -> [w2214] mode=indexing
                  tunnel: w2193 -> [w2213]
                  tunnel: [w2212] -> w2192
                  n901 = Join Numbers(hi=w2216, lo=w2215) -> ((hi.lo)=w2219:u32)
                  n902 = To Double Precision Float(number=w2214) -> (double precision float=w2220:dbl)
                  n903 = Number To Decimal String(number=w2228) -> (decimal integer string=w2233:string)  [unwired: 1 in]
                  n904 = Number To Fractional String(number=w2225, precision (6)=i16 3 ("width (-)")) -> (F-format string=w2235:string)  [unwired: 2 in]
                  n905 = Number To Fractional String(number=w2224, precision (6)=i16 3 ("width (-)")) -> (F-format string=w2231:string)  [unwired: 2 in]
                  n906 = Number To Fractional String(number=w2223, precision (6)=i16 3 ("width (-)")) -> (F-format string=w2229:string)  [unwired: 2 in]
                  n907 = Number To Fractional String(number=w2222, precision (6)=i16 3 ("width (-)")) -> (F-format string=w2226:string)  [unwired: 2 in]
                  n908 = Divide(x=w2220, y=w2213) -> (x/y=w2221:dbl)
                  n909 = To Unsigned Quad Integer(1:w2219) -> (0:w2218:u64)
                  n910 = Build Array(w2233, w2235, w2231, w2229, w2226) -> (w2234:string[])
                  n911 = call "Unix Time to Timestamp.vi"("Fractional Second"=w2221, "Unix Time (s)"=w2218) -> ("Timestamp"=w2217:timestamp)  [unwired: 8 in, 1 out]
                  n912 = To Double Precision Float(number=w2217) -> (double precision float=w2212:dbl)
                }
                n913 = Build Path(base path=w2188, name or relative path=w2191) -> (appended path=w2189:path)
                n914 = Open/Create/Replace File(file path (use dialog)=w2189, operation (0:open)=T10."open or create") -> (refnum out=w2182:refnum<file>, error out=w2180:errorcluster)  [unwired: 4 in, 1 out]
                n915 = Write to Text File(file (use dialog)=w2182, text=w2183, error in=w2180) -> (refnum out=w2181:refnum<file>, error out=w2179:errorcluster)  [unwired: 1 in, 1 out]
                n916 = Close File(refnum=w2181, error in=w2179) -> (path=w2168:path)  [unwired: 1 out]
              }
              frame 30 {
                w2244 = T13 2 items=["User Home"=0, "User Desktop"=1, "User Documents"=2, "User Application Data"=3, "User Preferences"=4, "User Temporary"=5, "Public Documents"=6, "Public Application Data"=7, "Public Preferences"=8, "Public Cache"=13, "System Core Libraries"=9, "System Installed Libraries"=10, "Application Files"=11, "Boot Volume Root"=12] ("system directory type")
                n917 = Search and Replace String(replace all?=TRUE ("replace all? (F)"), input string=w2239, search string="/") -> (result string=w2260:string)  [unwired: 5 in, 3 out]
                n918 = Concatenate Strings(w2237, "TimeStamp;Measure Ch_X(g);Ch_Y(g);INC_X(Deg);INC_Y(Deg)", "\n") -> (w2253:string)
                n919 = call <vilib>:"Get System Directory.vi"("system directory type"=w2244) -> ("system directory"=w2254:path)  [unwired: 10 in]
                n920 = Concatenate Strings(w2260, "_" ("string"), "streaming.csv") -> (w2261:string)
                n921 = Build Path(base path=w2254, name or relative path="Logfile") -> (appended path=w2255:path)
                n922 = call <vilib>:"Check if File or Folder Exists.vi"("path"=w2255) -> ("file or folder exists?"=w2256:bool, "dup path"=w2257:path)  [unwired: 8 in, 1 out]
                n923 = case shown="False" w2256 {
                  tunnel: w2257 -> [w2280 w2281]
                  tunnel: [w2279 w2281] -> w2258
                  frame False {
                    n924 = Create Folder(path (use dialog)=w2280) -> (created path=w2279:path)  [unwired: 2 in, 2 out]
                  }
                  frame True {
                  }
                }
                n925 = Decimate 1D Array(w2277) -> (w2276:dbl[], w2274:dbl[], w2272:dbl[], w2273:dbl[])
                n926 = for {
                  tunnel: [w2304] -> w2271 mode=indexing
                  tunnel: w2275 -> [w2298] mode=indexing
                  tunnel: w2276 -> [w2295] mode=indexing
                  tunnel: w2274 -> [w2294] mode=indexing
                  tunnel: w2272 -> [w2293] mode=indexing
                  tunnel: w2273 -> [w2292] mode=indexing
                  tunnel: [w2295] -> w2270 mode=indexing
                  tunnel: [w2294] -> w2269 mode=indexing
                  tunnel: [w2293] -> w2268 mode=indexing
                  tunnel: [w2292] -> w2267 mode=indexing
                  tunnel: w2266 -> [w2286]
                  tunnel: w2265 -> [w2285]
                  tunnel: w2264 -> [w2284] mode=indexing
                  tunnel: w2263 -> [w2283]
                  tunnel: [w2282] -> w2262
                  n927 = Join Numbers(hi=w2286, lo=w2285) -> ((hi.lo)=w2289:u32)
                  n928 = To Double Precision Float(number=w2284) -> (double precision float=w2290:dbl)
                  n929 = Number To Decimal String(number=w2298) -> (decimal integer string=w2303:string)  [unwired: 1 in]
                  n930 = Number To Fractional String(number=w2295, precision (6)=i16 3 ("width (-)")) -> (F-format string=w2305:string)  [unwired: 2 in]
                  n931 = Number To Fractional String(number=w2294, precision (6)=i16 3 ("width (-)")) -> (F-format string=w2301:string)  [unwired: 2 in]
                  n932 = Number To Fractional String(number=w2293, precision (6)=i16 3 ("width (-)")) -> (F-format string=w2299:string)  [unwired: 2 in]
                  n933 = Number To Fractional String(number=w2292, precision (6)=i16 3 ("width (-)")) -> (F-format string=w2296:string)  [unwired: 2 in]
                  n934 = Divide(x=w2290, y=w2283) -> (x/y=w2291:dbl)
                  n935 = To Unsigned Quad Integer(1:w2289) -> (0:w2288:u64)
                  n936 = Build Array(w2303, w2305, w2301, w2299, w2296) -> (w2304:string[])
                  n937 = call "Unix Time to Timestamp.vi"("Fractional Second"=w2291, "Unix Time (s)"=w2288) -> ("Timestamp"=w2287:timestamp)  [unwired: 8 in, 1 out]
                  n938 = To Double Precision Float(number=w2287) -> (double precision float=w2282:dbl)
                }
                n939 = Build Path(base path=w2258, name or relative path=w2261) -> (appended path=w2259:path)
                n940 = Open/Create/Replace File(file path (use dialog)=w2259, operation (0:open)=T10."open or create") -> (refnum out=w2252:refnum<file>, error out=w2250:errorcluster)  [unwired: 4 in, 1 out]
                n941 = Write to Text File(file (use dialog)=w2252, text=w2253, error in=w2250) -> (refnum out=w2251:refnum<file>, error out=w2249:errorcluster)  [unwired: 1 in, 1 out]
                n942 = Close File(refnum=w2251, error in=w2249) -> (path=w2238:path)  [unwired: 1 out]
              }
              frame 31 {
                w2314 = T13 2 items=["User Home"=0, "User Desktop"=1, "User Documents"=2, "User Application Data"=3, "User Preferences"=4, "User Temporary"=5, "Public Documents"=6, "Public Application Data"=7, "Public Preferences"=8, "Public Cache"=13, "System Core Libraries"=9, "System Installed Libraries"=10, "Application Files"=11, "Boot Volume Root"=12] ("system directory type")
                n943 = Search and Replace String(replace all?=TRUE ("replace all? (F)"), input string=w2309, search string="/") -> (result string=w2330:string)  [unwired: 5 in, 3 out]
                n944 = Concatenate Strings(w2307, "TimeStamp;Measure Ch_Z(g);Ch_X(g);Ch_Y(g);INC_X(Deg);INC_Y(Deg)", "\n") -> (w2323:string)
                n945 = call <vilib>:"Get System Directory.vi"("system directory type"=w2314) -> ("system directory"=w2324:path)  [unwired: 10 in]
                n946 = Concatenate Strings(w2330, "_" ("string"), "streaming.csv") -> (w2331:string)
                n947 = Build Path(base path=w2324, name or relative path="Logfile") -> (appended path=w2325:path)
                n948 = call <vilib>:"Check if File or Folder Exists.vi"("path"=w2325) -> ("file or folder exists?"=w2326:bool, "dup path"=w2327:path)  [unwired: 8 in, 1 out]
                n949 = case shown="False" w2326 {
                  tunnel: w2327 -> [w2352 w2353]
                  tunnel: [w2351 w2353] -> w2328
                  frame False {
                    n950 = Create Folder(path (use dialog)=w2352) -> (created path=w2351:path)  [unwired: 2 in, 2 out]
                  }
                  frame True {
                  }
                }
                n951 = Decimate 1D Array(w2349) -> (w2348:dbl[], w2347:dbl[], w2346:dbl[], w2345:dbl[], w2343:dbl[])
                n952 = for {
                  tunnel: [w2379] -> w2342 mode=indexing
                  tunnel: w2344 -> [w2373] mode=indexing
                  tunnel: w2348 -> [w2368] mode=indexing
                  tunnel: w2347 -> [w2367] mode=indexing
                  tunnel: w2346 -> [w2366] mode=indexing
                  tunnel: w2345 -> [w2365] mode=indexing
                  tunnel: w2343 -> [w2364] mode=indexing
                  tunnel: [w2368] -> w2341 mode=indexing
                  tunnel: [w2367] -> w2340 mode=indexing
                  tunnel: [w2366] -> w2339 mode=indexing
                  tunnel: [w2365] -> w2338 mode=indexing
                  tunnel: [w2364] -> w2337 mode=indexing
                  tunnel: w2336 -> [w2358]
                  tunnel: w2335 -> [w2357]
                  tunnel: w2334 -> [w2356] mode=indexing
                  tunnel: w2333 -> [w2355]
                  tunnel: [w2354] -> w2332
                  n953 = Join Numbers(hi=w2358, lo=w2357) -> ((hi.lo)=w2361:u32)
                  n954 = To Double Precision Float(number=w2356) -> (double precision float=w2362:dbl)
                  n955 = Number To Decimal String(number=w2373) -> (decimal integer string=w2378:string)  [unwired: 1 in]
                  n956 = Number To Fractional String(number=w2368, precision (6)=i16 3 ("width (-)")) -> (F-format string=w2380:string)  [unwired: 2 in]
                  n957 = Number To Fractional String(number=w2367, precision (6)=i16 3 ("width (-)")) -> (F-format string=w2376:string)  [unwired: 2 in]
                  n958 = Number To Fractional String(number=w2366, precision (6)=i16 3 ("width (-)")) -> (F-format string=w2374:string)  [unwired: 2 in]
                  n959 = Number To Fractional String(number=w2365, precision (6)=i16 3 ("width (-)")) -> (F-format string=w2371:string)  [unwired: 2 in]
                  n960 = Number To Fractional String(number=w2364, precision (6)=i16 3 ("width (-)")) -> (F-format string=w2369:string)  [unwired: 2 in]
                  n961 = Divide(x=w2362, y=w2355) -> (x/y=w2363:dbl)
                  n962 = To Unsigned Quad Integer(1:w2361) -> (0:w2360:u64)
                  n963 = Build Array(w2378, w2380, w2376, w2374, w2371, w2369) -> (w2379:string[])
                  n964 = call "Unix Time to Timestamp.vi"("Fractional Second"=w2363, "Unix Time (s)"=w2360) -> ("Timestamp"=w2359:timestamp)  [unwired: 8 in, 1 out]
                  n965 = To Double Precision Float(number=w2359) -> (double precision float=w2354:dbl)
                }
                n966 = Build Path(base path=w2328, name or relative path=w2331) -> (appended path=w2329:path)
                n967 = Open/Create/Replace File(file path (use dialog)=w2329, operation (0:open)=T10."open or create") -> (refnum out=w2322:refnum<file>, error out=w2320:errorcluster)  [unwired: 4 in, 1 out]
                n968 = Write to Text File(file (use dialog)=w2322, text=w2323, error in=w2320) -> (refnum out=w2321:refnum<file>, error out=w2319:errorcluster)  [unwired: 1 in, 1 out]
                n969 = Close File(refnum=w2321, error in=w2319) -> (path=w2308:path)  [unwired: 1 out]
              }
            }
            "Enabled channels" <- w309
            "CH_Z Graph" <- w321
            "CH_X Graph" <- w320
            "CH_Y Graph" <- w319
            "INC_X Graph" <- w318
            "INC_Y Graph" <- w317
            "File path" <- w312
            n970 = property on="INC_Y Graph" class="WFChart (strict)"("XScale.Offset"=w311) -> ()  [unwired: 2 in, 2 out]
            n971 = property on="CH_Z Graph" class="WFChart (strict)"("XScale.Offset"=w316) -> ()  [unwired: 2 in, 2 out]
            n972 = property on="CH_X Graph" class="WFChart (strict)"("XScale.Offset"=w315) -> ()  [unwired: 2 in, 2 out]
            n973 = property on="INC_X Graph" class="WFChart (strict)"("XScale.Offset"=w313) -> ()  [unwired: 2 in, 2 out]
            n974 = property on="CH_Y Graph" class="WFChart (strict)"("XScale.Offset"=w314) -> ()  [unwired: 2 in, 2 out]
            n975 = call-poly <vilib>:"Write Delimited Spreadsheet.vi"("file path (dialog if empty)"=w312, "format (%s)"="%s", "2D data"=w278, "append to file? (new file:F)"=TRUE, "transpose? (no:F)"=FALSE, "delimiter (\\t)"=";" ("delimiter (\\t)")) -> ()  [unwired: 8 in, 2 out]
          }
          frame 5 {
            w2454 = T13 2 items=["User Home"=0, "User Desktop"=1, "User Documents"=2, "User Application Data"=3, "User Preferences"=4, "User Temporary"=5, "Public Documents"=6, "Public Application Data"=7, "Public Preferences"=8, "Public Cache"=13, "System Core Libraries"=9, "System Installed Libraries"=10, "Application Files"=11, "Boot Volume Root"=12] ("system directory type")
            # "this block contain event date date"
            # "function to write data in log file"
            # "logfile path"
            # "precision"
            # "this block contain start date"
            # "measured value"
            # "this function contain end date"
            # "this block contain mathmode type +date"
            n976 = Less?(x=w2434, y=w2433) -> (x < y?=w2471:bool)
            n977 = call "Unix Time to Timestamp.vi"("Unix Time (s)"=w2434) -> ("Timestamp"=w2435:timestamp)  [unwired: 9 in, 1 out]
            n978 = call "Unix Time to Timestamp.vi"("Unix Time (s)"=w2478) -> ("Timestamp"=w2473:timestamp)  [unwired: 9 in, 1 out]
            n979 = String Subset(string=w2439, offset (0)=0, length (rest)=16 ("length (rest)")) -> (substring=w2438:string)
            n980 = case shown="1" w2475 {
              tunnel: [_ w2486 w2489] -> w2458
              tunnel: w2477 -> [_ w2485 w2488]
              frame Default {
              }
              frame 1 {
                n981 = Divide(x=w2485, y=-1000.0) -> (x/y=w2486:dbl)
              }
              frame 0 {
                n982 = Divide(x=w2488, y=1000.0) -> (x/y=w2489:dbl)
              }
            }
            n983 = Format Date/Time String(seconds (now)=w2435) -> (date/time string=w2437:string)  [unwired: 2 in]
            n984 = Concatenate Strings(w2438, "_" ("string"), w2444, "_" ("string"), "Transmit_Math_LowDutyCycle.txt") -> (w2447:string)
            n985 = Select(t="NA                 ", s=w2471, f=w2437) -> (s? t:f=w2456:string)
            n986 = call <vilib>:"Get System Directory.vi"("system directory type"=w2454) -> ("system directory"=w2455:path)  [unwired: 10 in]
            n987 = case shown="2" w2476 {
              tunnel: w2458 -> [w2492 w2495 w2498 _]
              tunnel: w2456 -> [w2493 w2496 _ _]
              tunnel: [w2492 _ _ _] -> _
              tunnel: [_ w2495 _ _] -> _
              tunnel: [_ _ w2498 _] -> _
              tunnel: ["Maximum value" "Minimum value" "Average value" _] -> w2459
              frame 1 {
                "Maximum value" <- w2492
                "Date" <- w2493
              }
              frame 2 {
                "Minimum value" <- w2495
                "Date" <- w2496
              }
              frame 3 {
                "Average value" <- w2498
              }
              frame Default {
              }
            }
            n988 = Build Path(base path=w2455, name or relative path="Logfile") -> (appended path=w2452:path)
            n989 = call <vilib>:"Check if File or Folder Exists.vi"("path"=w2452) -> ("file or folder exists?"=w2451:bool, "dup path"=w2450:path)  [unwired: 8 in, 1 out]
            n990 = case shown="False" w2451 {
              tunnel: w2450 -> [w2483 w2484]
              tunnel: [w2482 w2484] -> w2449
              frame False {
                n991 = Create Folder(path (use dialog)=w2483) -> (created path=w2482:path)  [unwired: 2 in, 2 out]
              }
              frame True {
              }
            }
            n992 = call "Unix Time to Timestamp.vi"("Unix Time (s)"=w2433) -> ("Timestamp"=w2472:timestamp)  [unwired: 9 in, 1 out]
            n993 = Format Date/Time String(seconds (now)=w2473) -> (date/time string=w2460:string)  [unwired: 2 in]
            "End Date" <- w2460
            n994 = Format Date/Time String(seconds (now)=w2472) -> (date/time string=w2446:string)  [unwired: 2 in]
            "Start Date" <- w2446
            n995 = Number To Fractional String(number=w2458, precision (6)=i16 3) -> (F-format string=w2457:string)  [unwired: 2 in]
            n996 = Build Path(base path=w2449, name or relative path=w2447) -> (appended path=w2448:path)
            "File path" <- w2448
            n997 = Format Into String(format string="%s %s;%s %s;%s %s;%s %s", "Start Date  ", w2446, "End Date", w2460, "Event Date", w2456, w2459, w2457) -> (resulting string=w2465:string)  [unwired: 2 in, 1 out]
            n998 = Build Array(w2465) -> (w2466:string[])
            n999 = call-poly <vilib>:"Write Delimited Spreadsheet.vi"("file path (dialog if empty)"=w2448, "1D data"=w2466, "append to file? (new file:F)"=TRUE, "transpose? (no:F)"=TRUE, "delimiter (\\t)"="\\t") -> ()  [unwired: 9 in, 2 out]
          }
          frame 6 {
            # "this block contain measures+ time stamp which saved in the logfile"
            # "this block contain device type"
            # "this block contain measure mode"
            # "this block contain time reference"
            # "logfile headers"
            n1000 = String To Byte Array(string=w2637) -> (unsigned byte array=w2584:u8[])
            n1001 = String Subset(string=w2503, offset (0)=0, length (rest)=16 ("length (rest)")) -> (substring=w2502:string)
            n1002 = Array Size(array=w2584) -> (size(s)=w2606:i32)
            n1003 = Array To Cluster(array=w2584) -> (cluster=w2638:T14)
            n1004 = Array Subset(array=w2584, index=2, length=8) -> (w2645:u8[])
            n1005 = Array Subset(array=w2584, index=10, length=4) -> (w2642:u8[])
            n1006 = Array Subset(array=w2584, index=14, length=17) -> (w2583:u8[])
            n1007 = Unbundle(w2638) -> ("unsigned byte array[0]"=w2560:u8, "unsigned byte array[1]"=w2580:u8)
            n1008 = Array To Cluster(array=w2645) -> (cluster=w2585:T11)
            n1009 = Subtract(x=w2606, y=30) -> (x-y=w2602:i32)
            n1010 = Array To Cluster(array=w2583) -> (cluster=w2634:T15)
            n1011 = Unbundle By Name(w2634) -> ("[0]"=w2633:u8, "[1]"=w2632:u8, "[2]"=w2631:u8, "[3]"=w2628:u8, "[4]"=w2627:u8, "[5]"=w2625:u8, "[6]"=w2624:u8, "[7]"=w2623:u8, "[8]"=w2620:u8, "[9]"=w2619:u8, "[10]"=w2618:u8, "[11]"=w2615:u8, "[12]"=w2614:u8, "[13]"=w2610:u8, "[14]"=→"Network Quality (LQI)":u8, "[15]"=→"channel that received alarm":u8)
            n1012 = Unbundle By Name(w2585) -> ("[0]"=w2590:u8, "[1]"=w2591:u8, "[2]"=w2594:u8, "[3]"=w2595:u8, "[4]"=w2588:u8, "[5]"=w2589:u8, "[6]"=w2597:u8, "[7]"=w2596:u8)
            n1013 = Array To Cluster(array=w2642) -> (cluster=w2641:T11)
            n1014 = Join Numbers(hi=w2632, lo=w2633) -> ((hi.lo)=w2630:u16)
            n1015 = Join Numbers(hi=w2627, lo=w2628) -> ((hi.lo)=w2626:u16)
            n1016 = Join Numbers(hi=w2624, lo=w2625) -> ((hi.lo)=w2622:u16)
            n1017 = Join Numbers(hi=w2619, lo=w2620) -> ((hi.lo)=w2617:u16)
            n1018 = Join Numbers(hi=w2614, lo=w2615) -> ((hi.lo)=w2613:u16)
            n1019 = Equal To 0?(x=w2610) -> (x = 0?=→"not synchronised":bool)
            n1020 = Not Equal To 0?(x=w2610) -> (x != 0?=→"synchronised":bool)
            n1021 = Join Numbers(hi=w2631, lo=w2630) -> ((hi.lo)=w2629:u32)
            n1022 = Join Numbers(hi=w2623, lo=w2622) -> ((hi.lo)=w2621:u32)
            n1023 = Join Numbers(hi=w2618, lo=w2617) -> ((hi.lo)=w2616:u32)
            n1024 = To Word Integer(number=w2626) -> (16bit integer=w2581:i16)
            "Number of daq per channel" <- w2581
            n1025 = To Word Integer(number=w2613) -> (16bit integer=→"Prev.Number of daq per channel":i16)
            n1026 = Join Numbers "time"(hi=w2591, lo=w2590) -> ((hi.lo)=w2587:u16)
            n1027 = Join Numbers "date"(hi=w2595, lo=w2594) -> ((hi.lo)=w2593:u16)
            n1028 = Unbundle By Name(w2641) -> ("[0]"=w2640:u8)
            n1029 = Join Numbers(hi=w2596, lo=w2597) -> ((hi.lo)=w2598:u16)
            n1030 = Array Subset(array=w2584, index=30, length=w2602) -> (w2604:u8[])
            n1031 = Join Numbers(hi=w2589, lo=w2588) -> ((hi.lo)=w2579:u16)
            "millisec" <- w2579
            n1032 = To Long Integer(number=w2629) -> (32bit integer=w2582:i32)
            "Frame sequence Id" <- w2582
            n1033 = To Long Integer(number=w2621) -> (32bit integer=w2509:i32)
            "Data Notification cycle" <- w2509
            n1034 = To Long Integer(number=w2616) -> (32bit integer=w2508:i32)
            "Data acquisition duration" <- w2508
            n1035 = To Word Integer(number=w2598) -> (16bit integer=w2500:i16)
            "Sampling rate" <- w2500
            n1036 = Multiply(x=w2581, y=w2582) -> (x*y=w2569:i32)
            n1037 = Number To Decimal String(number=w2509) -> (decimal integer string=w2518:string)  [unwired: 1 in]
            n1038 = Number To Decimal String(number=w2508) -> (decimal integer string=w2515:string)  [unwired: 1 in]
            n1039 = Decimate 1D Array(w2604) -> (w2599:u8[], w2603:u8[], w2601:u8[])
            n1040 = To Unsigned Byte Integer(number=w2640) -> (unsigned 8bit integer=w2499:u8)
            n1041 = To Unsigned Word Integer(number=w2593) -> (unsigned 16bit integer=w2554:u16)
            n1042 = Number To Decimal String(number=w2500) -> (decimal integer string=w2521:string)  [unwired: 1 in]
            n1043 = Join Numbers(hi=w2603, lo=w2599) -> ((hi.lo)=w2600:u16[])
            n1044 = Divide(x=w2579, y=1000) -> (x/y=w2574:dbl)
            n1045 = To Unsigned Word Integer(number=w2574) -> (unsigned 16bit integer=w2578:u16)
            n1046 = Add(x=w2587, y=w2578) -> (x+y=w2555:u16)
            n1047 = for {
              tunnel: w2601 -> [w2659] mode=indexing
              tunnel: [w2655] -> w2562 mode=indexing
              tunnel: w2600 -> [w2656] mode=indexing
              n1048 = To Word Integer(number=w2659) -> (16bit integer=w2657:i16)
              n1049 = Sign(1:w2657) -> (0:w2658:i16)
              n1050 = case shown="1" w2658 {
                tunnel: [_ w2661 w2664] -> w2655
                tunnel: w2656 -> [_ w2660 w2663]
                frame Default {
                }
                frame 1 {
                  n1051 = Divide(x=w2660, y=-1000.0) -> (x/y=w2661:dbl)
                }
                frame 0 {
                  n1052 = Divide(x=w2663, y=1000.0) -> (x/y=w2664:dbl)
                }
              }
            }
            n1053 = Join Numbers(hi=w2554, lo=w2555) -> ((hi.lo)=w2592:u32)
            n1054 = To Quad Integer(1:w2592) -> (0:w2575:i64)
            n1055 = call "Unix Time to Timestamp.vi"("Fractional Second"=w2574, "Unix Time (s)"=w2575) -> ("Timestamp"=w2577:timestamp)  [unwired: 8 in, 1 out]
            n1056 = Format Date/Time String(time format string (%c)="%x %X %.3u", seconds (now)=w2577) -> (date/time string=w2510:string)  [unwired: 1 in]
            "Time Ref" <- w2510
            n1057 = To Unsigned Quad Integer(1:w2569) -> (0:w2568:u64)
            n1058 = Increment(x=w2568) -> (x+1=w2570:u64)
            n1059 = for {
              N: w2570 -> [_]
              tunnel: w2568 -> [w2654]
              tunnel: [w2654] -> w2572
            }
            n1060 = case shown="6" w2580 {
              tunnel: ["" "LDCDA mode" "Alarm mode" "Streaming mode" "Shock Detection mode" "LDC Math Result" "S_E_T" "Dynamic Math Result"] -> w2512
              frame Default {
              }
              frame 1 {
              }
              frame 2 {
              }
              frame 3 {
              }
              frame 4 {
              }
              frame 5 {
              }
              frame 6 {
              }
              frame 7 {
              }
            }
            "Measure Mode" <- w2512
            n1061 = case shown="5" w2560 {
              tunnel: ["AX-3D" "HI_INC_MONO" "HI_INC_BI" "X_INC_MONO " "X _INC_BI " "AX_3DS" ""] -> w2511
              frame 1 {
              }
              frame 2 {
              }
              frame 3 {
              }
              frame 4 {
              }
              frame 5 {
              }
              frame 6 {
              }
              frame Default {
              }
            }
            "Device Type" <- w2511
            n1062 = Decrement(x=w2572) -> (x-1=w2571:u64)
            n1063 = for {
              tunnel: w2562 -> [w2651] mode=indexing
              shift-right: [w2653] -> _
              shift-left: w2571 -> [w2650]
              tunnel: [w2652] -> w2553 mode=indexing
              tunnel: [w2651] -> _ mode=indexing
              n1064 = Increment(x=w2650) -> (x+1=w2653:u64)
              n1065 = To Unsigned Quad Integer(1:w2653) -> (0:w2652:u64)
            }
            n1066 = Concatenate Strings("Device type :", w2511, ";", "Measure Mode :", w2512, ";", "Time reference :" ("string"), w2510, ";", " Sampling rate :", w2521, ";" ("string"), "Data acquisition cycle :" ("string"), w2518, ";" ("string"), "Data acquisition duration :" ("string"), w2515, ";" ("string"), "\n") -> (w2528:string)
            n1067 = Search and Replace String(replace all?=TRUE ("replace all? (F)"), input string=w2510, search string=":", replace string="_") -> (result string=w2539:string)  [unwired: 4 in, 3 out]
            n1068 = Search and Replace String(replace all?=TRUE ("replace all? (F)"), input string=w2539, search string=",", replace string="_") -> (result string=w2538:string)  [unwired: 4 in, 3 out]
            n1069 = Search and Replace String(replace all?=TRUE ("replace all? (F)"), input string=w2538, search string="/", replace string="_") -> (result string=w2534:string)  [unwired: 4 in, 3 out]
            n1070 = Build Array(w2528) -> (w2506:string[])
            n1071 = String Subset(string=w2534, offset (0)=0, length (rest)=20 ("length (rest)")) -> (substring=w2531:string)
            n1072 = To Double Precision Float(number=w2500) -> (double precision float=w2552:dbl)
            n1073 = call <vilib>:"Space Constant.vi"() -> ("String"=w2530:string)
            n1074 = Concatenate Strings(w2531, "_" ("string"), w2502, w2530) -> (w2507:string)
            n1075 = case shown="11111" w2499 {
              tunnel: ["" "no active channel" "chZ " "chX " "chZ & chX " "chY" "chZ & chY" "chX & chY " "chZ& chX& chY " "INC_X" "chZ & INC_X " "chX & INC_X " "chZ& chX & INC_X " "chY & INC_X " "chZ  & chY & INC_X are activated " "chX  & chY & INC_X " "chZ& chX  & chY & INC_X " "INC_Y  " " chZ & INC_Y " " chX & INC_Y" "chZ & chX & INC_Y " " chY & INC_Y" "chZ & chY & INC_Y" "chX & chY & INC_Y " " chZ &chX & chY & INC_Y " " INC_X & INC_Y " "chZ &   INC_X & INC_Y " "chX & INC_X & INC_Y " " chZ & chX &  INC_X & INC_Y " " chY &  INC_X & INC_Y " "chZ & chY &  INC_X & INC_Y " "chX & chY &  INC_X & INC_Y " "chZ & chX & chY &  INC_X & INC_Y  "] -> w2639
              tunnel: w2562 -> [_ _ w2717 w2772 w2829 w2887 w2945 w3006 w3070 w3131 w3189 w3250 w3314 w3378 w3442 w3509 w3579 w3643 w3701 w3761 w3825 w3888 w3952 w4019 w4086 w4151 w4213 w4278 w4345 w4413 w4480 w4550 w4622]
              tunnel: [_ _ w2714 w2769 w2825 w2884 w2943 w3002 w3066 w3130 w3186 w3248 w3310 w3374 w3438 w3504 w3574 w3640 w3698 w3758 w3822 w3885 w3949 w4016 w4081 w4147 w4209 w4274 w4344 w4408 w4477 w4544 w4615] -> w2563
              tunnel: w2553 -> [_ _ w2716 w2771 w2828 w2885 w2944 w3005 w3065 w3129 w3187 w3249 w3313 w3377 w3441 w3508 w3578 w3642 w3700 w3760 w3824 w3887 w3951 w4017 w4082 w4150 w4212 w4275 w4341 w4412 w4479 w4548 w4617]
              tunnel: [_ _ w2713 _ w2824 _ w2940 _ w3064 _ w3184 _ w3308 _ w3436 _ w3572 _ w3696 _ w3819 _ w3946 _ w4079 _ w4207 _ w4338 _ w4473 _ w4614] -> w2561
              tunnel: [_ _ _ w2768 w2823 _ _ w3001 w3063 _ _ w3245 w3307 _ _ w3503 w3571 _ _ w3756 w3818 _ _ w4013 w4078 _ _ w4272 w4337 _ _ w4543 w4613] -> w2559
              tunnel: [_ _ _ _ _ w2883 w2939 w3000 w3062 _ _ _ _ w3373 w3435 w3502 w3570 _ _ _ _ w3883 w3945 w4012 w4077 _ _ _ _ w4407 w4472 w4542 w4612] -> w2558
              tunnel: [_ _ _ _ _ _ _ _ _ w3127 w3183 w3244 w3306 w3372 w3434 w3501 w3569 _ _ _ _ _ _ _ _ w4146 w4206 w4271 w4336 w4406 w4471 w4541 w4611] -> w2557
              tunnel: [_ _ _ _ _ _ _ _ _ _ _ _ _ _ _ _ _ w3639 w3695 w3755 w3817 w3882 w3944 w4011 w4076 w4145 w4205 w4270 w4335 w4405 w4470 w4540 w4610] -> w2556
              tunnel: w2555 -> [_ _ w2712 w2766 w2821 w2881 w2937 w2998 w3060 w3125 w3181 w3242 w3304 w3370 w3432 w3499 w3567 w3637 w3693 w3753 w3815 w3880 w3942 w4009 w4074 w4143 w4203 w4268 w4333 w4403 w4468 w4538 w4608]
              tunnel: w2554 -> [_ _ w2711 w2767 w2822 w2882 w2938 w2999 w3061 w3126 w3182 w3243 w3305 w3371 w3433 w3500 w3568 w3638 w3694 w3754 w3816 w3881 w3943 w4010 w4075 w4144 w4204 w4269 w4334 w4404 w4469 w4539 w4609]
              tunnel: w2553 -> [_ _ w2710 w2765 w2820 w2880 w2936 w2997 w3059 w3124 w3180 w3241 w3303 w3369 w3431 w3498 w3566 w3636 w3692 w3752 w3814 w3879 w3941 w4008 w4073 w4142 w4202 w4267 w4332 w4402 w4467 w4537 w4607]
              tunnel: w2552 -> [_ _ w2709 w2764 w2819 w2879 w2935 w2996 w3058 w3123 w3179 w3240 w3302 w3368 w3430 w3497 w3565 w3635 w3691 w3751 w3813 w3878 w3940 w4007 w4072 w4141 w4201 w4266 w4331 w4401 w4466 w4536 w4606]
              tunnel: [_ _ w2708 _ w2818 _ w2934 _ w3057 _ w3178 _ w3301 _ w3429 _ w3564 _ w3690 _ w3812 _ w3939 _ w4071 _ w4200 _ w4330 _ w4465 _ w4605] -> w2551
              tunnel: [_ _ _ w2763 w2818 _ _ w2995 w3056 _ _ w3239 w3300 _ _ w3496 w3563 _ _ w3750 w3811 _ _ w4006 w4071 _ _ w4265 w4330 _ _ w4535 w4605] -> w2501
              tunnel: [_ _ _ _ _ w2878 w2933 w2994 w3055 _ _ _ _ w3367 w3428 w3495 w3562 _ _ _ _ w3877 w3938 w4005 w4071 _ _ _ _ w4400 w4465 w4535 w4605] -> w2550
              tunnel: [_ _ _ _ _ _ _ _ _ w3122 w3177 w3238 w3299 w3366 w3427 w3494 w3561 _ _ _ _ _ _ _ _ w4140 w4200 w4265 w4330 w4400 w4465 w4535 w4605] -> w2549
              tunnel: [_ _ _ _ _ _ _ _ _ _ _ _ _ _ _ _ _ w3634 w3689 w3750 w3810 w3877 w3937 w4004 w4071 w4140 w4200 w4265 w4330 w4400 w4465 w4535 w4605] -> w2547
              tunnel: w2507 -> [_ _ w2694 w2740 w2795 w2855 w2909 w2971 w3032 w3099 w3154 w3215 w3276 w3343 w3404 w3471 w3538 w3611 w3666 w3726 w3787 w3853 w3914 w3981 w4047 w4117 w4177 w4242 w4307 w4377 w4442 w4512 w4582]
              tunnel: [_ _ w2684 w2739 w2794 w2854 w2910 w2969 w3031 w3098 w3153 w3214 w3275 w3342 w3403 w3470 w3537 w3610 w3665 w3727 w3786 w3854 w3913 w3980 w4048 w4116 w4176 w4241 w4306 w4376 w4441 w4511 w4581] -> w2548
              tunnel: w2506 -> [_ _ w2683 w2738 w2793 w2853 w2908 w2970 w3030 w3097 w3152 w3213 w3274 w3341 w3402 w3469 w3536 w3609 w3664 w3725 w3785 w3852 w3912 w3979 w4046 w4115 w4175 w4240 w4305 w4375 w4440 w4510 w4580]
              frame Default {
              }
              frame 0 {
              }
              frame 1 {
                w2689 = T13 2 items=["User Home"=0, "User Desktop"=1, "User Documents"=2, "User Application Data"=3, "User Preferences"=4, "User Temporary"=5, "Public Documents"=6, "Public Application Data"=7, "Public Preferences"=8, "Public Cache"=13, "System Core Libraries"=9, "System Installed Libraries"=10, "Application Files"=11, "Boot Volume Root"=12] ("system directory type")
                n1076 = Decimate 1D Array(w2717) -> (w2715:dbl[])
                n1077 = Search and Replace String(replace all?=TRUE ("replace all? (F)"), input string=w2694, search string="/") -> (result string=w2706:string)  [unwired: 5 in, 3 out]
                n1078 = for {
                  tunnel: w2715 -> [w2732] mode=indexing
                  tunnel: [w2735] -> w2714 mode=indexing
                  tunnel: w2716 -> [w2734] mode=indexing
                  tunnel: [w2732] -> w2713 mode=indexing
                  tunnel: w2712 -> [w2727]
                  tunnel: w2711 -> [w2726]
                  tunnel: w2710 -> [w2725] mode=indexing
                  tunnel: w2709 -> [w2724]
                  tunnel: [w2722] -> w2708
                  n1079 = Join Numbers(hi=w2726, lo=w2727) -> ((hi.lo)=w2729:u32)
                  n1080 = To Double Precision Float(number=w2725) -> (double precision float=w2730:dbl)
                  n1081 = Number To Decimal String(number=w2734) -> (decimal integer string=w2733:string)  [unwired: 1 in]
                  n1082 = Number To Fractional String(number=w2732, precision (6)=i16 3 ("width (-)")) -> (F-format string=w2736:string)  [unwired: 2 in]
                  n1083 = Divide(x=w2730, y=w2724) -> (x/y=w2731:dbl)
                  n1084 = To Unsigned Quad Integer(1:w2729) -> (0:w2728:u64)
                  n1085 = Build Array(w2733, w2736) -> (w2735:string[])
                  n1086 = call "Unix Time to Timestamp.vi"("Fractional Second"=w2731, "Unix Time (s)"=w2728) -> ("Timestamp"=w2723:timestamp)  [unwired: 8 in, 1 out]
                  n1087 = To Double Precision Float(number=w2723) -> (double precision float=w2722:dbl)
                }
                n1088 = Concatenate Strings(w2683, "TimeStamp;MeasureCh_Z(g);", "\n") -> (w2699:string)
                n1089 = call <vilib>:"Get System Directory.vi"("system directory type"=w2689) -> ("system directory"=w2700:path)  [unwired: 10 in]
                n1090 = Concatenate Strings(w2706, "_" ("string"), "S_E_T.csv") -> (w2707:string)
                n1091 = Build Path(base path=w2700, name or relative path="Logfile") -> (appended path=w2701:path)
                n1092 = call <vilib>:"Check if File or Folder Exists.vi"("path"=w2701) -> ("file or folder exists?"=w2702:bool, "dup path"=w2703:path)  [unwired: 8 in, 1 out]
                n1093 = case shown="False" w2702 {
                  tunnel: w2703 -> [w2720 w2721]
                  tunnel: [w2719 w2721] -> w2704
                  frame False {
                    n1094 = Create Folder(path (use dialog)=w2720) -> (created path=w2719:path)  [unwired: 2 in, 2 out]
                  }
                  frame True {
                  }
                }
                n1095 = Build Path(base path=w2704, name or relative path=w2707) -> (appended path=w2705:path)
                n1096 = Open/Create/Replace File(file path (use dialog)=w2705, operation (0:open)=T10."open or create") -> (refnum out=w2698:refnum<file>, error out=w2696:errorcluster)  [unwired: 4 in, 1 out]
                n1097 = Write to Text File(file (use dialog)=w2698, text=w2699, error in=w2696) -> (refnum out=w2697:refnum<file>, error out=w2695:errorcluster)  [unwired: 1 in, 1 out]
                n1098 = Close File(refnum=w2697, error in=w2695) -> (path=w2684:path)  [unwired: 1 out]
              }
              frame 2 {
                w2745 = T13 2 items=["User Home"=0, "User Desktop"=1, "User Documents"=2, "User Application Data"=3, "User Preferences"=4, "User Temporary"=5, "Public Documents"=6, "Public Application Data"=7, "Public Preferences"=8, "Public Cache"=13, "System Core Libraries"=9, "System Installed Libraries"=10, "Application Files"=11, "Boot Volume Root"=12] ("system directory type")
                n1099 = Decimate 1D Array(w2772) -> (w2770:dbl[])
                n1100 = Search and Replace String(replace all?=TRUE ("replace all? (F)"), input string=w2740, search string="/") -> (result string=w2761:string)  [unwired: 5 in, 3 out]
                n1101 = for {
                  tunnel: w2770 -> [w2787] mode=indexing
                  tunnel: [w2790] -> w2769 mode=indexing
                  tunnel: w2771 -> [w2789] mode=indexing
                  tunnel: [w2787] -> w2768 mode=indexing
                  tunnel: w2767 -> [w2782]
                  tunnel: w2766 -> [w2781]
                  tunnel: w2765 -> [w2780] mode=indexing
                  tunnel: w2764 -> [w2779]
                  tunnel: [w2777] -> w2763
                  n1102 = Join Numbers(hi=w2782, lo=w2781) -> ((hi.lo)=w2784:u32)
                  n1103 = To Double Precision Float(number=w2780) -> (double precision float=w2785:dbl)
                  n1104 = Number To Decimal String(number=w2789) -> (decimal integer string=w2788:string)  [unwired: 1 in]
                  n1105 = Number To Fractional String(number=w2787, precision (6)=i16 3 ("width (-)")) -> (F-format string=w2791:string)  [unwired: 2 in]
                  n1106 = Divide(x=w2785, y=w2779) -> (x/y=w2786:dbl)
                  n1107 = To Unsigned Quad Integer(1:w2784) -> (0:w2783:u64)
                  n1108 = Build Array(w2788, w2791) -> (w2790:string[])
                  n1109 = call "Unix Time to Timestamp.vi"("Fractional Second"=w2786, "Unix Time (s)"=w2783) -> ("Timestamp"=w2778:timestamp)  [unwired: 8 in, 1 out]
                  n1110 = To Double Precision Float(number=w2778) -> (double precision float=w2777:dbl)
                }
                n1111 = Concatenate Strings(w2738, "TimeStamp;MeasureCh_X(g);", "\n") -> (w2754:string)
                n1112 = call <vilib>:"Get System Directory.vi"("system directory type"=w2745) -> ("system directory"=w2755:path)  [unwired: 10 in]
                n1113 = Concatenate Strings(w2761, "_" ("string"), "S_E_T.csv") -> (w2762:string)
                n1114 = Build Path(base path=w2755, name or relative path="Logfile") -> (appended path=w2756:path)
                n1115 = call <vilib>:"Check if File or Folder Exists.vi"("path"=w2756) -> ("file or folder exists?"=w2757:bool, "dup path"=w2758:path)  [unwired: 8 in, 1 out]
                n1116 = case shown="False" w2757 {
                  tunnel: w2758 -> [w2775 w2776]
                  tunnel: [w2774 w2776] -> w2759
                  frame False {
                    n1117 = Create Folder(path (use dialog)=w2775) -> (created path=w2774:path)  [unwired: 2 in, 2 out]
                  }
                  frame True {
                  }
                }
                n1118 = Build Path(base path=w2759, name or relative path=w2762) -> (appended path=w2760:path)
                n1119 = Open/Create/Replace File(file path (use dialog)=w2760, operation (0:open)=T10."open or create") -> (refnum out=w2753:refnum<file>, error out=w2751:errorcluster)  [unwired: 4 in, 1 out]
                n1120 = Write to Text File(file (use dialog)=w2753, text=w2754, error in=w2751) -> (refnum out=w2752:refnum<file>, error out=w2750:errorcluster)  [unwired: 1 in, 1 out]
                n1121 = Close File(refnum=w2752, error in=w2750) -> (path=w2739:path)  [unwired: 1 out]
              }
              frame 3 {
                w2800 = T13 2 items=["User Home"=0, "User Desktop"=1, "User Documents"=2, "User Application Data"=3, "User Preferences"=4, "User Temporary"=5, "Public Documents"=6, "Public Application Data"=7, "Public Preferences"=8, "Public Cache"=13, "System Core Libraries"=9, "System Installed Libraries"=10, "Application Files"=11, "Boot Volume Root"=12] ("system directory type")
                n1122 = Decimate 1D Array(w2829) -> (w2827:dbl[], w2826:dbl[])
                n1123 = Search and Replace String(replace all?=TRUE ("replace all? (F)"), input string=w2795, search string="/") -> (result string=w2816:string)  [unwired: 5 in, 3 out]
                n1124 = Concatenate Strings(w2793, "TimeStamp;MeasureCh_Z(g);Ch_X(g);", "\n") -> (w2809:string)
                n1125 = for {
                  tunnel: w2827 -> [w2845] mode=indexing
                  tunnel: w2826 -> [w2844] mode=indexing
                  tunnel: [w2848] -> w2825 mode=indexing
                  tunnel: w2828 -> [w2847] mode=indexing
                  tunnel: [w2845] -> w2824 mode=indexing
                  tunnel: [w2844] -> w2823 mode=indexing
                  tunnel: w2822 -> [w2839]
                  tunnel: w2821 -> [w2838]
                  tunnel: w2820 -> [w2837] mode=indexing
                  tunnel: w2819 -> [w2836]
                  tunnel: [w2834] -> w2818
                  n1126 = Join Numbers(hi=w2839, lo=w2838) -> ((hi.lo)=w2841:u32)
                  n1127 = To Double Precision Float(number=w2837) -> (double precision float=w2842:dbl)
                  n1128 = Number To Decimal String(number=w2847) -> (decimal integer string=w2846:string)  [unwired: 1 in]
                  n1129 = Number To Fractional String(number=w2845, precision (6)=i16 3 ("width (-)")) -> (F-format string=w2850:string)  [unwired: 2 in]
                  n1130 = Number To Fractional String(number=w2844, precision (6)=i16 3 ("width (-)")) -> (F-format string=w2849:string)  [unwired: 2 in]
                  n1131 = Divide(x=w2842, y=w2836) -> (x/y=w2843:dbl)
                  n1132 = To Unsigned Quad Integer(1:w2841) -> (0:w2840:u64)
                  n1133 = Build Array(w2846, w2850, w2849) -> (w2848:string[])
                  n1134 = call "Unix Time to Timestamp.vi"("Fractional Second"=w2843, "Unix Time (s)"=w2840) -> ("Timestamp"=w2835:timestamp)  [unwired: 8 in, 1 out]
                  n1135 = To Double Precision Float(number=w2835) -> (double precision float=w2834:dbl)
                }
                n1136 = call <vilib>:"Get System Directory.vi"("system directory type"=w2800) -> ("system directory"=w2810:path)  [unwired: 10 in]
                n1137 = Concatenate Strings(w2816, "_" ("string"), "S_E_T.csv") -> (w2817:string)
                n1138 = Build Path(base path=w2810, name or relative path="Logfile") -> (appended path=w2811:path)
                n1139 = call <vilib>:"Check if File or Folder Exists.vi"("path"=w2811) -> ("file or folder exists?"=w2812:bool, "dup path"=w2813:path)  [unwired: 8 in, 1 out]
                n1140 = case shown="False" w2812 {
                  tunnel: w2813 -> [w2832 w2833]
                  tunnel: [w2831 w2833] -> w2814
                  frame False {
                    n1141 = Create Folder(path (use dialog)=w2832) -> (created path=w2831:path)  [unwired: 2 in, 2 out]
                  }
                  frame True {
                  }
                }
                n1142 = Build Path(base path=w2814, name or relative path=w2817) -> (appended path=w2815:path)
                n1143 = Open/Create/Replace File(file path (use dialog)=w2815, operation (0:open)=T10."open or create") -> (refnum out=w2808:refnum<file>, error out=w2806:errorcluster)  [unwired: 4 in, 1 out]
                n1144 = Write to Text File(file (use dialog)=w2808, text=w2809, error in=w2806) -> (refnum out=w2807:refnum<file>, error out=w2805:errorcluster)  [unwired: 1 in, 1 out]
                n1145 = Close File(refnum=w2807, error in=w2805) -> (path=w2794:path)  [unwired: 1 out]
              }
              frame 4 {
                w2860 = T13 2 items=["User Home"=0, "User Desktop"=1, "User Documents"=2, "User Application Data"=3, "User Preferences"=4, "User Temporary"=5, "Public Documents"=6, "Public Application Data"=7, "Public Preferences"=8, "Public Cache"=13, "System Core Libraries"=9, "System Installed Libraries"=10, "Application Files"=11, "Boot Volume Root"=12] ("system directory type")
                # "this function calculate Time  of subpacket"
                n1146 = Decimate 1D Array(w2887) -> (w2886:dbl[])
                n1147 = Search and Replace String(replace all?=TRUE ("replace all? (F)"), input string=w2855, search string="/") -> (result string=w2876:string)  [unwired: 5 in, 3 out]
                n1148 = Concatenate Strings(w2853, "TimeStamp;MeasureCh_Y(g);", "\n") -> (w2869:string)
                n1149 = for {
                  tunnel: w2886 -> [w2902] mode=indexing
                  tunnel: [w2905] -> w2884 mode=indexing
                  tunnel: w2885 -> [w2904] mode=indexing
                  tunnel: [w2902] -> w2883 mode=indexing
                  tunnel: w2882 -> [w2896]
                  tunnel: w2881 -> [w2893]
                  tunnel: w2880 -> [w2894] mode=indexing
                  tunnel: w2879 -> [w2895]
                  tunnel: [w2892] -> w2878
                  n1150 = Join Numbers(hi=w2896, lo=w2893) -> ((hi.lo)=w2899:u32)
                  n1151 = To Double Precision Float(number=w2894) -> (double precision float=w2900:dbl)
                  n1152 = Number To Decimal String(number=w2904) -> (decimal integer string=w2903:string)  [unwired: 1 in]
                  n1153 = Number To Fractional String(number=w2902, precision (6)=i16 3 ("width (-)")) -> (F-format string=w2906:string)  [unwired: 2 in]
                  n1154 = Divide(x=w2900, y=w2895) -> (x/y=w2901:dbl)
                  n1155 = To Unsigned Quad Integer(1:w2899) -> (0:w2898:u64)
                  n1156 = Build Array(w2903, w2906) -> (w2905:string[])
                  n1157 = call "Unix Time to Timestamp.vi"("Fractional Second"=w2901, "Unix Time (s)"=w2898) -> ("Timestamp"=w2897:timestamp)  [unwired: 8 in, 1 out]
                  n1158 = To Double Precision Float(number=w2897) -> (double precision float=w2892:dbl)
                }
                n1159 = call <vilib>:"Get System Directory.vi"("system directory type"=w2860) -> ("system directory"=w2870:path)  [unwired: 10 in]
                n1160 = Concatenate Strings(w2876, "_" ("string"), "S_E_T.csv") -> (w2877:string)
                n1161 = Build Path(base path=w2870, name or relative path="Logfile") -> (appended path=w2871:path)
                n1162 = call <vilib>:"Check if File or Folder Exists.vi"("path"=w2871) -> ("file or folder exists?"=w2872:bool, "dup path"=w2873:path)  [unwired: 8 in, 1 out]
                n1163 = case shown="False" w2872 {
                  tunnel: w2873 -> [w2890 w2891]
                  tunnel: [w2889 w2891] -> w2874
                  frame False {
                    n1164 = Create Folder(path (use dialog)=w2890) -> (created path=w2889:path)  [unwired: 2 in, 2 out]
                  }
                  frame True {
                  }
                }
                n1165 = Build Path(base path=w2874, name or relative path=w2877) -> (appended path=w2875:path)
                n1166 = Open/Create/Replace File(file path (use dialog)=w2875, operation (0:open)=T10."open or create") -> (refnum out=w2868:refnum<file>, error out=w2866:errorcluster)  [unwired: 4 in, 1 out]
                n1167 = Write to Text File(file (use dialog)=w2868, text=w2869, error in=w2866) -> (refnum out=w2867:refnum<file>, error out=w2865:errorcluster)  [unwired: 1 in, 1 out]
                n1168 = Close File(refnum=w2867, error in=w2865) -> (path=w2854:path)  [unwired: 1 out]
              }
              frame 5 {
                w2915 = T13 2 items=["User Home"=0, "User Desktop"=1, "User Documents"=2, "User Application Data"=3, "User Preferences"=4, "User Temporary"=5, "Public Documents"=6, "Public Application Data"=7, "Public Preferences"=8, "Public Cache"=13, "System Core Libraries"=9, "System Installed Libraries"=10, "Application Files"=11, "Boot Volume Root"=12] ("system directory type")
                n1169 = Decimate 1D Array(w2945) -> (w2941:dbl[], w2942:dbl[])
                n1170 = Search and Replace String(replace all?=TRUE ("replace all? (F)"), input string=w2909, search string="/") -> (result string=w2931:string)  [unwired: 5 in, 3 out]
                n1171 = for {
                  tunnel: [w2964] -> w2943 mode=indexing
                  tunnel: w2944 -> [w2963] mode=indexing
                  tunnel: w2941 -> [w2961] mode=indexing
                  tunnel: w2942 -> [w2960] mode=indexing
                  tunnel: [w2961] -> w2940 mode=indexing
                  tunnel: [w2960] -> w2939 mode=indexing
                  tunnel: w2938 -> [w2954]
                  tunnel: w2937 -> [w2953]
                  tunnel: w2936 -> [w2952] mode=indexing
                  tunnel: w2935 -> [w2951]
                  tunnel: [w2950] -> w2934
                  tunnel: [w2950] -> w2933
                  n1172 = Join Numbers(hi=w2954, lo=w2953) -> ((hi.lo)=w2957:u32)
                  n1173 = To Double Precision Float(number=w2952) -> (double precision float=w2958:dbl)
                  n1174 = Number To Decimal String(number=w2963) -> (decimal integer string=w2962:string)  [unwired: 1 in]
                  n1175 = Number To Fractional String(number=w2961, precision (6)=i16 3 ("width (-)")) -> (F-format string=w2966:string)  [unwired: 2 in]
                  n1176 = Number To Fractional String(number=w2960, precision (6)=i16 3 ("width (-)")) -> (F-format string=w2965:string)  [unwired: 2 in]
                  n1177 = Divide(x=w2958, y=w2951) -> (x/y=w2959:dbl)
                  n1178 = To Unsigned Quad Integer(1:w2957) -> (0:w2956:u64)
                  n1179 = Build Array(w2962, w2966, w2965) -> (w2964:string[])
                  n1180 = call "Unix Time to Timestamp.vi"("Fractional Second"=w2959, "Unix Time (s)"=w2956) -> ("Timestamp"=w2955:timestamp)  [unwired: 8 in, 1 out]
                  n1181 = To Double Precision Float(number=w2955) -> (double precision float=w2950:dbl)
                }
                n1182 = Concatenate Strings(w2908, "TimeStamp;MeasureCh_Z(g);Ch_Y(g);", "\n") -> (w2924:string)
                n1183 = call <vilib>:"Get System Directory.vi"("system directory type"=w2915) -> ("system directory"=w2925:path)  [unwired: 10 in]
                n1184 = Concatenate Strings(w2931, "_" ("string"), "S_E_T.csv") -> (w2932:string)
                n1185 = Build Path(base path=w2925, name or relative path="Logfile") -> (appended path=w2926:path)
                n1186 = call <vilib>:"Check if File or Folder Exists.vi"("path"=w2926) -> ("file or folder exists?"=w2927:bool, "dup path"=w2928:path)  [unwired: 8 in, 1 out]
                n1187 = case shown="False" w2927 {
                  tunnel: w2928 -> [w2948 w2949]
                  tunnel: [w2947 w2949] -> w2929
                  frame False {
                    n1188 = Create Folder(path (use dialog)=w2948) -> (created path=w2947:path)  [unwired: 2 in, 2 out]
                  }
                  frame True {
                  }
                }
                n1189 = Build Path(base path=w2929, name or relative path=w2932) -> (appended path=w2930:path)
                n1190 = Open/Create/Replace File(file path (use dialog)=w2930, operation (0:open)=T10."open or create") -> (refnum out=w2923:refnum<file>, error out=w2921:errorcluster)  [unwired: 4 in, 1 out]
                n1191 = Write to Text File(file (use dialog)=w2923, text=w2924, error in=w2921) -> (refnum out=w2922:refnum<file>, error out=w2920:errorcluster)  [unwired: 1 in, 1 out]
                n1192 = Close File(refnum=w2922, error in=w2920) -> (path=w2910:path)  [unwired: 1 out]
              }
              frame 6 {
                w2976 = T13 2 items=["User Home"=0, "User Desktop"=1, "User Documents"=2, "User Application Data"=3, "User Preferences"=4, "User Temporary"=5, "Public Documents"=6, "Public Application Data"=7, "Public Preferences"=8, "Public Cache"=13, "System Core Libraries"=9, "System Installed Libraries"=10, "Application Files"=11, "Boot Volume Root"=12] ("system directory type")
                n1193 = Decimate 1D Array(w3006) -> (w3004:dbl[], w3003:dbl[])
                n1194 = Search and Replace String(replace all?=TRUE ("replace all? (F)"), input string=w2971, search string="/") -> (result string=w2992:string)  [unwired: 5 in, 3 out]
                n1195 = for {
                  tunnel: w3004 -> [w3022] mode=indexing
                  tunnel: w3003 -> [w3021] mode=indexing
                  tunnel: [w3025] -> w3002 mode=indexing
                  tunnel: w3005 -> [w3024] mode=indexing
                  tunnel: [w3022] -> w3001 mode=indexing
                  tunnel: [w3021] -> w3000 mode=indexing
                  tunnel: w2999 -> [w3015]
                  tunnel: w2998 -> [w3014]
                  tunnel: w2997 -> [w3013] mode=indexing
                  tunnel: w2996 -> [w3012]
                  tunnel: [w3011] -> w2995
                  tunnel: [w3011] -> w2994
                  n1196 = Join Numbers(hi=w3015, lo=w3014) -> ((hi.lo)=w3018:u32)
                  n1197 = To Double Precision Float(number=w3013) -> (double precision float=w3019:dbl)
                  n1198 = Number To Decimal String(number=w3024) -> (decimal integer string=w3023:string)  [unwired: 1 in]
                  n1199 = Number To Fractional String(number=w3022, precision (6)=i16 3 ("width (-)")) -> (F-format string=w3027:string)  [unwired: 2 in]
                  n1200 = Number To Fractional String(number=w3021, precision (6)=i16 3 ("width (-)")) -> (F-format string=w3026:string)  [unwired: 2 in]
                  n1201 = Divide(x=w3019, y=w3012) -> (x/y=w3020:dbl)
                  n1202 = To Unsigned Quad Integer(1:w3018) -> (0:w3017:u64)
                  n1203 = Build Array(w3023, w3027, w3026) -> (w3025:string[])
                  n1204 = call "Unix Time to Timestamp.vi"("Fractional Second"=w3020, "Unix Time (s)"=w3017) -> ("Timestamp"=w3016:timestamp)  [unwired: 8 in, 1 out]
                  n1205 = To Double Precision Float(number=w3016) -> (double precision float=w3011:dbl)
                }
                n1206 = Concatenate Strings(w2970, "TimeStamp;MeasureCh_X(g);Ch_Y(g);", "\n") -> (w2985:string)
                n1207 = call <vilib>:"Get System Directory.vi"("system directory type"=w2976) -> ("system directory"=w2986:path)  [unwired: 10 in]
                n1208 = Concatenate Strings(w2992, "_" ("string"), "S_E_T.csv") -> (w2993:string)
                n1209 = Build Path(base path=w2986, name or relative path="Logfile") -> (appended path=w2987:path)
                n1210 = call <vilib>:"Check if File or Folder Exists.vi"("path"=w2987) -> ("file or folder exists?"=w2988:bool, "dup path"=w2989:path)  [unwired: 8 in, 1 out]
                n1211 = case shown="False" w2988 {
                  tunnel: w2989 -> [w3009 w3010]
                  tunnel: [w3008 w3010] -> w2990
                  frame False {
                    n1212 = Create Folder(path (use dialog)=w3009) -> (created path=w3008:path)  [unwired: 2 in, 2 out]
                  }
                  frame True {
                  }
                }
                n1213 = Build Path(base path=w2990, name or relative path=w2993) -> (appended path=w2991:path)
                n1214 = Open/Create/Replace File(file path (use dialog)=w2991, operation (0:open)=T10."open or create") -> (refnum out=w2984:refnum<file>, error out=w2982:errorcluster)  [unwired: 4 in, 1 out]
                n1215 = Write to Text File(file (use dialog)=w2984, text=w2985, error in=w2982) -> (refnum out=w2983:refnum<file>, error out=w2981:errorcluster)  [unwired: 1 in, 1 out]
                n1216 = Close File(refnum=w2983, error in=w2981) -> (path=w2969:path)  [unwired: 1 out]
              }
              frame 7 {
                w3037 = T13 2 items=["User Home"=0, "User Desktop"=1, "User Documents"=2, "User Application Data"=3, "User Preferences"=4, "User Temporary"=5, "Public Documents"=6, "Public Application Data"=7, "Public Preferences"=8, "Public Cache"=13, "System Core Libraries"=9, "System Installed Libraries"=10, "Application Files"=11, "Boot Volume Root"=12] ("system directory type")
                n1217 = Search and Replace String(replace all?=TRUE ("replace all? (F)"), input string=w3032, search string="/") -> (result string=w3053:string)  [unwired: 5 in, 3 out]
                n1218 = Concatenate Strings(w3030, "TimeStamp;MeasureCh_Z(g);Ch_X(g);Ch_Y(g);", "\n") -> (w3046:string)
                n1219 = call <vilib>:"Get System Directory.vi"("system directory type"=w3037) -> ("system directory"=w3047:path)  [unwired: 10 in]
                n1220 = Concatenate Strings(w3053, "_" ("string"), "S_E_T.csv") -> (w3054:string)
                n1221 = Build Path(base path=w3047, name or relative path="Logfile") -> (appended path=w3048:path)
                n1222 = call <vilib>:"Check if File or Folder Exists.vi"("path"=w3048) -> ("file or folder exists?"=w3049:bool, "dup path"=w3050:path)  [unwired: 8 in, 1 out]
                n1223 = case shown="False" w3049 {
                  tunnel: w3050 -> [w3073 w3074]
                  tunnel: [w3072 w3074] -> w3051
                  frame False {
                    n1224 = Create Folder(path (use dialog)=w3073) -> (created path=w3072:path)  [unwired: 2 in, 2 out]
                  }
                  frame True {
                  }
                }
                n1225 = Decimate 1D Array(w3070) -> (w3069:dbl[], w3068:dbl[], w3067:dbl[])
                n1226 = for {
                  tunnel: w3069 -> [w3087] mode=indexing
                  tunnel: w3068 -> [w3086] mode=indexing
                  tunnel: w3067 -> [w3085] mode=indexing
                  tunnel: [w3090] -> w3066 mode=indexing
                  tunnel: w3065 -> [w3089] mode=indexing
                  tunnel: [w3087] -> w3064 mode=indexing
                  tunnel: [w3086] -> w3063 mode=indexing
                  tunnel: [w3085] -> w3062 mode=indexing
                  tunnel: w3061 -> [w3079]
                  tunnel: w3060 -> [w3078]
                  tunnel: w3059 -> [w3077] mode=indexing
                  tunnel: w3058 -> [w3076]
                  tunnel: [w3075] -> w3057
                  tunnel: [w3075] -> w3056
                  tunnel: [w3075] -> w3055
                  n1227 = Join Numbers(hi=w3079, lo=w3078) -> ((hi.lo)=w3082:u32)
                  n1228 = To Double Precision Float(number=w3077) -> (double precision float=w3083:dbl)
                  n1229 = Number To Decimal String(number=w3089) -> (decimal integer string=w3088:string)  [unwired: 1 in]
                  n1230 = Number To Fractional String(number=w3087, precision (6)=i16 3 ("width (-)")) -> (F-format string=w3094:string)  [unwired: 2 in]
                  n1231 = Number To Fractional String(number=w3086, precision (6)=i16 3 ("width (-)")) -> (F-format string=w3093:string)  [unwired: 2 in]
                  n1232 = Number To Fractional String(number=w3085, precision (6)=i16 3 ("width (-)")) -> (F-format string=w3091:string)  [unwired: 2 in]
                  n1233 = Divide(x=w3083, y=w3076) -> (x/y=w3084:dbl)
                  n1234 = To Unsigned Quad Integer(1:w3082) -> (0:w3081:u64)
                  n1235 = Build Array(w3088, w3094, w3093, w3091) -> (w3090:string[])
                  n1236 = call "Unix Time to Timestamp.vi"("Fractional Second"=w3084, "Unix Time (s)"=w3081) -> ("Timestamp"=w3080:timestamp)  [unwired: 8 in, 1 out]
                  n1237 = To Double Precision Float(number=w3080) -> (double precision float=w3075:dbl)
                }
                n1238 = Build Path(base path=w3051, name or relative path=w3054) -> (appended path=w3052:path)
                n1239 = Open/Create/Replace File(file path (use dialog)=w3052, operation (0:open)=T10."open or create") -> (refnum out=w3045:refnum<file>, error out=w3043:errorcluster)  [unwired: 4 in, 1 out]
                n1240 = Write to Text File(file (use dialog)=w3045, text=w3046, error in=w3043) -> (refnum out=w3044:refnum<file>, error out=w3042:errorcluster)  [unwired: 1 in, 1 out]
                n1241 = Close File(refnum=w3044, error in=w3042) -> (path=w3031:path)  [unwired: 1 out]
              }
              frame 8 {
                w3104 = T13 2 items=["User Home"=0, "User Desktop"=1, "User Documents"=2, "User Application Data"=3, "User Preferences"=4, "User Temporary"=5, "Public Documents"=6, "Public Application Data"=7, "Public Preferences"=8, "Public Cache"=13, "System Core Libraries"=9, "System Installed Libraries"=10, "Application Files"=11, "Boot Volume Root"=12] ("system directory type")
                n1242 = Decimate 1D Array(w3131) -> (w3128:dbl[])
                n1243 = Search and Replace String(replace all?=TRUE ("replace all? (F)"), input string=w3099, search string="/") -> (result string=w3120:string)  [unwired: 5 in, 3 out]
                n1244 = for {
                  tunnel: [w3150] -> w3130 mode=indexing
                  tunnel: w3129 -> [w3147] mode=indexing
                  tunnel: w3128 -> [w3146] mode=indexing
                  tunnel: [w3146] -> w3127 mode=indexing
                  tunnel: w3126 -> [w3140]
                  tunnel: w3125 -> [w3139]
                  tunnel: w3124 -> [w3138] mode=indexing
                  tunnel: w3123 -> [w3137]
                  tunnel: [w3136] -> w3122
                  n1245 = Join Numbers(hi=w3140, lo=w3139) -> ((hi.lo)=w3143:u32)
                  n1246 = To Double Precision Float(number=w3138) -> (double precision float=w3144:dbl)
                  n1247 = Number To Decimal String(number=w3147) -> (decimal integer string=w3149:string)  [unwired: 1 in]
                  n1248 = Number To Fractional String(number=w3146, precision (6)=i16 3 ("width (-)")) -> (F-format string=w3148:string)  [unwired: 2 in]
                  n1249 = Divide(x=w3144, y=w3137) -> (x/y=w3145:dbl)
                  n1250 = To Unsigned Quad Integer(1:w3143) -> (0:w3142:u64)
                  n1251 = Build Array(w3149, w3148) -> (w3150:string[])
                  n1252 = call "Unix Time to Timestamp.vi"("Fractional Second"=w3145, "Unix Time (s)"=w3142) -> ("Timestamp"=w3141:timestamp)  [unwired: 8 in, 1 out]
                  n1253 = To Double Precision Float(number=w3141) -> (double precision float=w3136:dbl)
                }
                n1254 = Concatenate Strings(w3097, "TimeStamp;Measure INC_X(Deg);", "\n") -> (w3113:string)
                n1255 = call <vilib>:"Get System Directory.vi"("system directory type"=w3104) -> ("system directory"=w3114:path)  [unwired: 10 in]
                n1256 = Concatenate Strings(w3120, "_" ("string"), "S_E_T.csv") -> (w3121:string)
                n1257 = Build Path(base path=w3114, name or relative path="Logfile") -> (appended path=w3115:path)
                n1258 = call <vilib>:"Check if File or Folder Exists.vi"("path"=w3115) -> ("file or folder exists?"=w3116:bool, "dup path"=w3117:path)  [unwired: 8 in, 1 out]
                n1259 = case shown="False" w3116 {
                  tunnel: w3117 -> [w3134 w3135]
                  tunnel: [w3133 w3135] -> w3118
                  frame False {
                    n1260 = Create Folder(path (use dialog)=w3134) -> (created path=w3133:path)  [unwired: 2 in, 2 out]
                  }
                  frame True {
                  }
                }
                n1261 = Build Path(base path=w3118, name or relative path=w3121) -> (appended path=w3119:path)
                n1262 = Open/Create/Replace File(file path (use dialog)=w3119, operation (0:open)=T10."open or create") -> (refnum out=w3112:refnum<file>, error out=w3110:errorcluster)  [unwired: 4 in, 1 out]
                n1263 = Write to Text File(file (use dialog)=w3112, text=w3113, error in=w3110) -> (refnum out=w3111:refnum<file>, error out=w3109:errorcluster)  [unwired: 1 in, 1 out]
                n1264 = Close File(refnum=w3111, error in=w3109) -> (path=w3098:path)  [unwired: 1 out]
              }
              frame 9 {
                w3159 = T13 2 items=["User Home"=0, "User Desktop"=1, "User Documents"=2, "User Application Data"=3, "User Preferences"=4, "User Temporary"=5, "Public Documents"=6, "Public Application Data"=7, "Public Preferences"=8, "Public Cache"=13, "System Core Libraries"=9, "System Installed Libraries"=10, "Application Files"=11, "Boot Volume Root"=12] ("system directory type")
                n1265 = Decimate 1D Array(w3189) -> (w3185:dbl[], w3188:dbl[])
                n1266 = Search and Replace String(replace all?=TRUE ("replace all? (F)"), input string=w3154, search string="/") -> (result string=w3175:string)  [unwired: 5 in, 3 out]
                n1267 = for {
                  tunnel: [w3208] -> w3186 mode=indexing
                  tunnel: w3185 -> [w3205] mode=indexing
                  tunnel: w3188 -> [w3204] mode=indexing
                  tunnel: w3187 -> [w3206] mode=indexing
                  tunnel: [w3205] -> w3184 mode=indexing
                  tunnel: [w3204] -> w3183 mode=indexing
                  tunnel: w3182 -> [w3198]
                  tunnel: w3181 -> [w3197]
                  tunnel: w3180 -> [w3196] mode=indexing
                  tunnel: w3179 -> [w3195]
                  tunnel: [w3194] -> w3177
                  tunnel: [w3194] -> w3178
                  n1268 = Join Numbers(hi=w3198, lo=w3197) -> ((hi.lo)=w3201:u32)
                  n1269 = To Double Precision Float(number=w3196) -> (double precision float=w3202:dbl)
                  n1270 = Number To Decimal String(number=w3206) -> (decimal integer string=w3207:string)  [unwired: 1 in]
                  n1271 = Number To Fractional String(number=w3205, precision (6)=i16 3 ("width (-)")) -> (F-format string=w3210:string)  [unwired: 2 in]
                  n1272 = Number To Fractional String(number=w3204, precision (6)=i16 3 ("width (-)")) -> (F-format string=w3209:string)  [unwired: 2 in]
                  n1273 = Divide(x=w3202, y=w3195) -> (x/y=w3203:dbl)
                  n1274 = To Unsigned Quad Integer(1:w3201) -> (0:w3200:u64)
                  n1275 = Build Array(w3207, w3210, w3209) -> (w3208:string[])
                  n1276 = call "Unix Time to Timestamp.vi"("Fractional Second"=w3203, "Unix Time (s)"=w3200) -> ("Timestamp"=w3199:timestamp)  [unwired: 8 in, 1 out]
                  n1277 = To Double Precision Float(number=w3199) -> (double precision float=w3194:dbl)
                }
                n1278 = Concatenate Strings(w3152, "TimeStamp;Measure Ch_Z(g);INC_X(Deg);", "\n") -> (w3168:string)
                n1279 = call <vilib>:"Get System Directory.vi"("system directory type"=w3159) -> ("system directory"=w3169:path)  [unwired: 10 in]
                n1280 = Concatenate Strings(w3175, "_" ("string"), "S_E_T.csv") -> (w3176:string)
                n1281 = Build Path(base path=w3169, name or relative path="Logfile") -> (appended path=w3170:path)
                n1282 = call <vilib>:"Check if File or Folder Exists.vi"("path"=w3170) -> ("file or folder exists?"=w3171:bool, "dup path"=w3172:path)  [unwired: 8 in, 1 out]
                n1283 = case shown="False" w3171 {
                  tunnel: w3172 -> [w3192 w3193]
                  tunnel: [w3191 w3193] -> w3173
                  frame False {
                    n1284 = Create Folder(path (use dialog)=w3192) -> (created path=w3191:path)  [unwired: 2 in, 2 out]
                  }
                  frame True {
                  }
                }
                n1285 = Build Path(base path=w3173, name or relative path=w3176) -> (appended path=w3174:path)
                n1286 = Open/Create/Replace File(file path (use dialog)=w3174, operation (0:open)=T10."open or create") -> (refnum out=w3167:refnum<file>, error out=w3165:errorcluster)  [unwired: 4 in, 1 out]
                n1287 = Write to Text File(file (use dialog)=w3167, text=w3168, error in=w3165) -> (refnum out=w3166:refnum<file>, error out=w3164:errorcluster)  [unwired: 1 in, 1 out]
                n1288 = Close File(refnum=w3166, error in=w3164) -> (path=w3153:path)  [unwired: 1 out]
              }
              frame 10 {
                w3220 = T13 2 items=["User Home"=0, "User Desktop"=1, "User Documents"=2, "User Application Data"=3, "User Preferences"=4, "User Temporary"=5, "Public Documents"=6, "Public Application Data"=7, "Public Preferences"=8, "Public Cache"=13, "System Core Libraries"=9, "System Installed Libraries"=10, "Application Files"=11, "Boot Volume Root"=12] ("system directory type")
                n1289 = Decimate 1D Array(w3250) -> (w3247:dbl[], w3246:dbl[])
                n1290 = Search and Replace String(replace all?=TRUE ("replace all? (F)"), input string=w3215, search string="/") -> (result string=w3236:string)  [unwired: 5 in, 3 out]
                n1291 = for {
                  tunnel: [w3266] -> _ mode=indexing
                  tunnel: [w3271] -> w3248 mode=indexing
                  tunnel: w3249 -> [w3270] mode=indexing
                  tunnel: w3247 -> [w3266] mode=indexing
                  tunnel: w3246 -> [w3265] mode=indexing
                  tunnel: [w3266] -> w3245 mode=indexing
                  tunnel: [w3265] -> w3244 mode=indexing
                  tunnel: w3243 -> [w3259]
                  tunnel: w3242 -> [w3258]
                  tunnel: w3241 -> [w3257] mode=indexing
                  tunnel: w3240 -> [w3256]
                  tunnel: [w3255] -> w3239
                  tunnel: [w3255] -> w3238
                  n1292 = Join Numbers(hi=w3259, lo=w3258) -> ((hi.lo)=w3262:u32)
                  n1293 = To Double Precision Float(number=w3257) -> (double precision float=w3263:dbl)
                  n1294 = Number To Decimal String(number=w3270) -> (decimal integer string=w3269:string)  [unwired: 1 in]
                  n1295 = Number To Fractional String(number=w3266, precision (6)=i16 3 ("width (-)")) -> (F-format string=w3272:string)  [unwired: 2 in]
                  n1296 = Number To Fractional String(number=w3265, width (-)=i16 3) -> (F-format string=w3268:string)  [unwired: 2 in]
                  n1297 = Divide(x=w3263, y=w3256) -> (x/y=w3264:dbl)
                  n1298 = To Unsigned Quad Integer(1:w3262) -> (0:w3261:u64)
                  n1299 = Build Array(w3269, w3272, w3268) -> (w3271:string[])
                  n1300 = call "Unix Time to Timestamp.vi"("Fractional Second"=w3264, "Unix Time (s)"=w3261) -> ("Timestamp"=w3260:timestamp)  [unwired: 8 in, 1 out]
                  n1301 = To Double Precision Float(number=w3260) -> (double precision float=w3255:dbl)
                }
                n1302 = Concatenate Strings(w3213, "TimeStamp;Measure Ch_X(g);INC_X(Deg);", "\n") -> (w3229:string)
                n1303 = call <vilib>:"Get System Directory.vi"("system directory type"=w3220) -> ("system directory"=w3230:path)  [unwired: 10 in]
                n1304 = Concatenate Strings(w3236, "_" ("string"), "S_E_T.csv") -> (w3237:string)
                n1305 = Build Path(base path=w3230, name or relative path="Logfile") -> (appended path=w3231:path)
                n1306 = call <vilib>:"Check if File or Folder Exists.vi"("path"=w3231) -> ("file or folder exists?"=w3232:bool, "dup path"=w3233:path)  [unwired: 8 in, 1 out]
                n1307 = case shown="False" w3232 {
                  tunnel: w3233 -> [w3253 w3254]
                  tunnel: [w3252 w3254] -> w3234
                  frame False {
                    n1308 = Create Folder(path (use dialog)=w3253) -> (created path=w3252:path)  [unwired: 2 in, 2 out]
                  }
                  frame True {
                  }
                }
                n1309 = Build Path(base path=w3234, name or relative path=w3237) -> (appended path=w3235:path)
                n1310 = Open/Create/Replace File(file path (use dialog)=w3235, operation (0:open)=T10."open or create") -> (refnum out=w3228:refnum<file>, error out=w3226:errorcluster)  [unwired: 4 in, 1 out]
                n1311 = Write to Text File(file (use dialog)=w3228, text=w3229, error in=w3226) -> (refnum out=w3227:refnum<file>, error out=w3225:errorcluster)  [unwired: 1 in, 1 out]
                n1312 = Close File(refnum=w3227, error in=w3225) -> (path=w3214:path)  [unwired: 1 out]
              }
              frame 11 {
                w3281 = T13 2 items=["User Home"=0, "User Desktop"=1, "User Documents"=2, "User Application Data"=3, "User Preferences"=4, "User Temporary"=5, "Public Documents"=6, "Public Application Data"=7, "Public Preferences"=8, "Public Cache"=13, "System Core Libraries"=9, "System Installed Libraries"=10, "Application Files"=11, "Boot Volume Root"=12] ("system directory type")
                n1313 = Search and Replace String(replace all?=TRUE ("replace all? (F)"), input string=w3276, search string="/") -> (result string=w3297:string)  [unwired: 5 in, 3 out]
                n1314 = Concatenate Strings(w3274, "TimeStamp;Measure Ch_Z(g);Ch_X(g);INC_X(Deg);", "\n") -> (w3290:string)
                n1315 = call <vilib>:"Get System Directory.vi"("system directory type"=w3281) -> ("system directory"=w3291:path)  [unwired: 10 in]
                n1316 = Concatenate Strings(w3297, "_" ("string"), "S_E_T.csv") -> (w3298:string)
                n1317 = Build Path(base path=w3291, name or relative path="Logfile") -> (appended path=w3292:path)
                n1318 = call <vilib>:"Check if File or Folder Exists.vi"("path"=w3292) -> ("file or folder exists?"=w3293:bool, "dup path"=w3294:path)  [unwired: 8 in, 1 out]
                n1319 = case shown="False" w3293 {
                  tunnel: w3294 -> [w3317 w3318]
                  tunnel: [w3316 w3318] -> w3295
                  frame False {
                    n1320 = Create Folder(path (use dialog)=w3317) -> (created path=w3316:path)  [unwired: 2 in, 2 out]
                  }
                  frame True {
                  }
                }
                n1321 = Decimate 1D Array(w3314) -> (w3312:dbl[], w3311:dbl[], w3309:dbl[])
                n1322 = for {
                  tunnel: [w3338] -> w3310 mode=indexing
                  tunnel: w3313 -> [w3334] mode=indexing
                  tunnel: w3312 -> [w3331] mode=indexing
                  tunnel: w3311 -> [w3330] mode=indexing
                  tunnel: w3309 -> [w3329] mode=indexing
                  tunnel: [w3331] -> w3308 mode=indexing
                  tunnel: [w3330] -> w3307 mode=indexing
                  tunnel: [w3329] -> w3306 mode=indexing
                  tunnel: w3305 -> [w3323]
                  tunnel: w3304 -> [w3322]
                  tunnel: w3303 -> [w3321] mode=indexing
                  tunnel: w3302 -> [w3320]
                  tunnel: [w3319] -> w3301
                  tunnel: [w3319] -> w3300
                  tunnel: [w3319] -> w3299
                  n1323 = Join Numbers(hi=w3323, lo=w3322) -> ((hi.lo)=w3326:u32)
                  n1324 = To Double Precision Float(number=w3321) -> (double precision float=w3327:dbl)
                  n1325 = Number To Decimal String(number=w3334) -> (decimal integer string=w3337:string)  [unwired: 1 in]
                  n1326 = Number To Fractional String(number=w3331, precision (6)=i16 3 ("width (-)")) -> (F-format string=w3339:string)  [unwired: 2 in]
                  n1327 = Number To Fractional String(number=w3330, width (-)=i16 3) -> (F-format string=w3336:string)  [unwired: 2 in]
                  n1328 = Number To Fractional String(number=w3329, width (-)=i16 3) -> (F-format string=w3332:string)  [unwired: 2 in]
                  n1329 = Divide(x=w3327, y=w3320) -> (x/y=w3328:dbl)
                  n1330 = To Unsigned Quad Integer(1:w3326) -> (0:w3325:u64)
                  n1331 = Build Array(w3337, w3339, w3336, w3332) -> (w3338:string[])
                  n1332 = call "Unix Time to Timestamp.vi"("Fractional Second"=w3328, "Unix Time (s)"=w3325) -> ("Timestamp"=w3324:timestamp)  [unwired: 8 in, 1 out]
                  n1333 = To Double Precision Float(number=w3324) -> (double precision float=w3319:dbl)
                }
                n1334 = Build Path(base path=w3295, name or relative path=w3298) -> (appended path=w3296:path)
                n1335 = Open/Create/Replace File(file path (use dialog)=w3296, operation (0:open)=T10."open or create") -> (refnum out=w3289:refnum<file>, error out=w3287:errorcluster)  [unwired: 4 in, 1 out]
                n1336 = Write to Text File(file (use dialog)=w3289, text=w3290, error in=w3287) -> (refnum out=w3288:refnum<file>, error out=w3286:errorcluster)  [unwired: 1 in, 1 out]
                n1337 = Close File(refnum=w3288, error in=w3286) -> (path=w3275:path)  [unwired: 1 out]
              }
              frame 12 {
                w3348 = T13 2 items=["User Home"=0, "User Desktop"=1, "User Documents"=2, "User Application Data"=3, "User Preferences"=4, "User Temporary"=5, "Public Documents"=6, "Public Application Data"=7, "Public Preferences"=8, "Public Cache"=13, "System Core Libraries"=9, "System Installed Libraries"=10, "Application Files"=11, "Boot Volume Root"=12] ("system directory type")
                n1338 = Decimate 1D Array(w3378) -> (w3376:dbl[], w3375:dbl[])
                n1339 = Search and Replace String(replace all?=TRUE ("replace all? (F)"), input string=w3343, search string="/") -> (result string=w3364:string)  [unwired: 5 in, 3 out]
                n1340 = Concatenate Strings(w3341, "TimeStamp;Measure Ch_Y(g);INC_X(Deg);", "\n") -> (w3357:string)
                n1341 = for {
                  tunnel: [w3399] -> w3374 mode=indexing
                  tunnel: w3377 -> [w3395] mode=indexing
                  tunnel: w3376 -> [w3394] mode=indexing
                  tunnel: w3375 -> [w3393] mode=indexing
                  tunnel: [w3394] -> w3373 mode=indexing
                  tunnel: [w3393] -> w3372 mode=indexing
                  tunnel: w3371 -> [w3387]
                  tunnel: w3370 -> [w3386]
                  tunnel: w3369 -> [w3385] mode=indexing
                  tunnel: w3368 -> [w3384]
                  tunnel: [w3383] -> w3367
                  tunnel: [w3383] -> w3366
                  n1342 = Join Numbers(hi=w3387, lo=w3386) -> ((hi.lo)=w3390:u32)
                  n1343 = To Double Precision Float(number=w3385) -> (double precision float=w3391:dbl)
                  n1344 = Number To Decimal String(number=w3395) -> (decimal integer string=w3398:string)  [unwired: 1 in]
                  n1345 = Number To Fractional String(number=w3394, precision (6)=i16 3 ("width (-)")) -> (F-format string=w3400:string)  [unwired: 2 in]
                  n1346 = Number To Fractional String(number=w3393, width (-)=i16 3) -> (F-format string=w3397:string)  [unwired: 2 in]
                  n1347 = Divide(x=w3391, y=w3384) -> (x/y=w3392:dbl)
                  n1348 = To Unsigned Quad Integer(1:w3390) -> (0:w3389:u64)
                  n1349 = Build Array(w3398, w3400, w3397) -> (w3399:string[])
                  n1350 = call "Unix Time to Timestamp.vi"("Fractional Second"=w3392, "Unix Time (s)"=w3389) -> ("Timestamp"=w3388:timestamp)  [unwired: 8 in, 1 out]
                  n1351 = To Double Precision Float(number=w3388) -> (double precision float=w3383:dbl)
                }
                n1352 = call <vilib>:"Get System Directory.vi"("system directory type"=w3348) -> ("system directory"=w3358:path)  [unwired: 10 in]
                n1353 = Concatenate Strings(w3364, "_" ("string"), "S_E_T.csv") -> (w3365:string)
                n1354 = Build Path(base path=w3358, name or relative path="Logfile") -> (appended path=w3359:path)
                n1355 = call <vilib>:"Check if File or Folder Exists.vi"("path"=w3359) -> ("file or folder exists?"=w3360:bool, "dup path"=w3361:path)  [unwired: 8 in, 1 out]
                n1356 = case shown="False" w3360 {
                  tunnel: w3361 -> [w3381 w3382]
                  tunnel: [w3380 w3382] -> w3362
                  frame False {
                    n1357 = Create Folder(path (use dialog)=w3381) -> (created path=w3380:path)  [unwired: 2 in, 2 out]
                  }
                  frame True {
                  }
                }
                n1358 = Build Path(base path=w3362, name or relative path=w3365) -> (appended path=w3363:path)
                n1359 = Open/Create/Replace File(file path (use dialog)=w3363, operation (0:open)=T10."open or create") -> (refnum out=w3356:refnum<file>, error out=w3354:errorcluster)  [unwired: 4 in, 1 out]
                n1360 = Write to Text File(file (use dialog)=w3356, text=w3357, error in=w3354) -> (refnum out=w3355:refnum<file>, error out=w3353:errorcluster)  [unwired: 1 in, 1 out]
                n1361 = Close File(refnum=w3355, error in=w3353) -> (path=w3342:path)  [unwired: 1 out]
              }
              frame 13 {
                w3409 = T13 2 items=["User Home"=0, "User Desktop"=1, "User Documents"=2, "User Application Data"=3, "User Preferences"=4, "User Temporary"=5, "Public Documents"=6, "Public Application Data"=7, "Public Preferences"=8, "Public Cache"=13, "System Core Libraries"=9, "System Installed Libraries"=10, "Application Files"=11, "Boot Volume Root"=12] ("system directory type")
                n1362 = Search and Replace String(replace all?=TRUE ("replace all? (F)"), input string=w3404, search string="/") -> (result string=w3425:string)  [unwired: 5 in, 3 out]
                n1363 = Concatenate Strings(w3402, "TimeStamp;Measure Ch_Z(g);Ch_Y(g);INC_X(Deg)", "\n") -> (w3418:string)
                n1364 = call <vilib>:"Get System Directory.vi"("system directory type"=w3409) -> ("system directory"=w3419:path)  [unwired: 10 in]
                n1365 = Concatenate Strings(w3425, "_" ("string"), "S_E_T.csv") -> (w3426:string)
                n1366 = Build Path(base path=w3419, name or relative path="Logfile") -> (appended path=w3420:path)
                n1367 = call <vilib>:"Check if File or Folder Exists.vi"("path"=w3420) -> ("file or folder exists?"=w3421:bool, "dup path"=w3422:path)  [unwired: 8 in, 1 out]
                n1368 = case shown="False" w3421 {
                  tunnel: w3422 -> [w3445 w3446]
                  tunnel: [w3444 w3446] -> w3423
                  frame False {
                    n1369 = Create Folder(path (use dialog)=w3445) -> (created path=w3444:path)  [unwired: 2 in, 2 out]
                  }
                  frame True {
                  }
                }
                n1370 = Decimate 1D Array(w3442) -> (w3437:dbl[], w3440:dbl[], w3439:dbl[])
                n1371 = for {
                  tunnel: [w3466] -> w3438 mode=indexing
                  tunnel: w3441 -> [w3462] mode=indexing
                  tunnel: w3437 -> [w3461] mode=indexing
                  tunnel: w3440 -> [w3460] mode=indexing
                  tunnel: w3439 -> [w3459] mode=indexing
                  tunnel: [w3461] -> w3436 mode=indexing
                  tunnel: [w3460] -> w3435 mode=indexing
                  tunnel: [w3459] -> w3434 mode=indexing
                  tunnel: w3433 -> [w3453]
                  tunnel: w3432 -> [w3452]
                  tunnel: w3431 -> [w3451] mode=indexing
                  tunnel: w3430 -> [w3450]
                  tunnel: [w3449] -> w3429
                  tunnel: [w3449] -> w3428
                  tunnel: [w3449] -> w3427
                  n1372 = Join Numbers(hi=w3453, lo=w3452) -> ((hi.lo)=w3456:u32)
                  n1373 = To Double Precision Float(number=w3451) -> (double precision float=w3457:dbl)
                  n1374 = Number To Decimal String(number=w3462) -> (decimal integer string=w3465:string)  [unwired: 1 in]
                  n1375 = Number To Fractional String(number=w3461, precision (6)=i16 3 ("width (-)")) -> (F-format string=w3467:string)  [unwired: 2 in]
                  n1376 = Number To Fractional String(number=w3460, precision (6)=i16 3 ("width (-)")) -> (F-format string=w3464:string)  [unwired: 2 in]
                  n1377 = Number To Fractional String(number=w3459, precision (6)=i16 3 ("width (-)")) -> (F-format string=w3463:string)  [unwired: 2 in]
                  n1378 = Divide(x=w3457, y=w3450) -> (x/y=w3458:dbl)
                  n1379 = To Unsigned Quad Integer(1:w3456) -> (0:w3455:u64)
                  n1380 = Build Array(w3465, w3467, w3464, w3463) -> (w3466:string[])
                  n1381 = call "Unix Time to Timestamp.vi"("Fractional Second"=w3458, "Unix Time (s)"=w3455) -> ("Timestamp"=w3454:timestamp)  [unwired: 8 in, 1 out]
                  n1382 = To Double Precision Float(number=w3454) -> (double precision float=w3449:dbl)
                }
                n1383 = Build Path(base path=w3423, name or relative path=w3426) -> (appended path=w3424:path)
                n1384 = Open/Create/Replace File(file path (use dialog)=w3424, operation (0:open)=T10."open or create") -> (refnum out=w3417:refnum<file>, error out=w3415:errorcluster)  [unwired: 4 in, 1 out]
                n1385 = Write to Text File(file (use dialog)=w3417, text=w3418, error in=w3415) -> (refnum out=w3416:refnum<file>, error out=w3414:errorcluster)  [unwired: 1 in, 1 out]
                n1386 = Close File(refnum=w3416, error in=w3414) -> (path=w3403:path)  [unwired: 1 out]
              }
              frame 14 {
                w3476 = T13 2 items=["User Home"=0, "User Desktop"=1, "User Documents"=2, "User Application Data"=3, "User Preferences"=4, "User Temporary"=5, "Public Documents"=6, "Public Application Data"=7, "Public Preferences"=8, "Public Cache"=13, "System Core Libraries"=9, "System Installed Libraries"=10, "Application Files"=11, "Boot Volume Root"=12] ("system directory type")
                n1387 = Search and Replace String(replace all?=TRUE ("replace all? (F)"), input string=w3471, search string="/") -> (result string=w3492:string)  [unwired: 5 in, 3 out]
                n1388 = Concatenate Strings(w3469, "TimeStamp;Measure Ch_X(g);Ch_Y(g);INC_X(Deg)", "\n") -> (w3485:string)
                n1389 = call <vilib>:"Get System Directory.vi"("system directory type"=w3476) -> ("system directory"=w3486:path)  [unwired: 10 in]
                n1390 = Concatenate Strings(w3492, "_" ("string"), "S_E_T.csv") -> (w3493:string)
                n1391 = Build Path(base path=w3486, name or relative path="Logfile") -> (appended path=w3487:path)
                n1392 = call <vilib>:"Check if File or Folder Exists.vi"("path"=w3487) -> ("file or folder exists?"=w3488:bool, "dup path"=w3489:path)  [unwired: 8 in, 1 out]
                n1393 = case shown="False" w3488 {
                  tunnel: w3489 -> [w3512 w3513]
                  tunnel: [w3511 w3513] -> w3490
                  frame False {
                    n1394 = Create Folder(path (use dialog)=w3512) -> (created path=w3511:path)  [unwired: 2 in, 2 out]
                  }
                  frame True {
                  }
                }
                n1395 = Decimate 1D Array(w3509) -> (w3507:dbl[], w3506:dbl[], w3505:dbl[])
                n1396 = for {
                  tunnel: [w3533] -> w3504 mode=indexing
                  tunnel: w3508 -> [w3529] mode=indexing
                  tunnel: w3507 -> [w3528] mode=indexing
                  tunnel: w3506 -> [w3527] mode=indexing
                  tunnel: w3505 -> [w3526] mode=indexing
                  tunnel: [w3528] -> w3503 mode=indexing
                  tunnel: [w3527] -> w3502 mode=indexing
                  tunnel: [w3526] -> w3501 mode=indexing
                  tunnel: w3500 -> [w3520]
                  tunnel: w3499 -> [w3519]
                  tunnel: w3498 -> [w3518] mode=indexing
                  tunnel: w3497 -> [w3517]
                  tunnel: [w3516] -> w3496
                  tunnel: [w3516] -> w3495
                  tunnel: [w3516] -> w3494
                  n1397 = Join Numbers(hi=w3520, lo=w3519) -> ((hi.lo)=w3523:u32)
                  n1398 = To Double Precision Float(number=w3518) -> (double precision float=w3524:dbl)
                  n1399 = Number To Decimal String(number=w3529) -> (decimal integer string=w3532:string)  [unwired: 1 in]
                  n1400 = Number To Fractional String(number=w3528, precision (6)=i16 3 ("width (-)")) -> (F-format string=w3534:string)  [unwired: 2 in]
                  n1401 = Number To Fractional String(number=w3527, precision (6)=i16 3 ("width (-)")) -> (F-format string=w3531:string)  [unwired: 2 in]
                  n1402 = Number To Fractional String(number=w3526, precision (6)=i16 3 ("width (-)")) -> (F-format string=w3530:string)  [unwired: 2 in]
                  n1403 = Divide(x=w3524, y=w3517) -> (x/y=w3525:dbl)
                  n1404 = To Unsigned Quad Integer(1:w3523) -> (0:w3522:u64)
                  n1405 = Build Array(w3532, w3534, w3531, w3530) -> (w3533:string[])
                  n1406 = call "Unix Time to Timestamp.vi"("Fractional Second"=w3525, "Unix Time (s)"=w3522) -> ("Timestamp"=w3521:timestamp)  [unwired: 8 in, 1 out]
                  n1407 = To Double Precision Float(number=w3521) -> (double precision float=w3516:dbl)
                }
                n1408 = Build Path(base path=w3490, name or relative path=w3493) -> (appended path=w3491:path)
                n1409 = Open/Create/Replace File(file path (use dialog)=w3491, operation (0:open)=T10."open or create") -> (refnum out=w3484:refnum<file>, error out=w3482:errorcluster)  [unwired: 4 in, 1 out]
                n1410 = Write to Text File(file (use dialog)=w3484, text=w3485, error in=w3482) -> (refnum out=w3483:refnum<file>, error out=w3481:errorcluster)  [unwired: 1 in, 1 out]
                n1411 = Close File(refnum=w3483, error in=w3481) -> (path=w3470:path)  [unwired: 1 out]
              }
              frame 15 {
                w3543 = T13 2 items=["User Home"=0, "User Desktop"=1, "User Documents"=2, "User Application Data"=3, "User Preferences"=4, "User Temporary"=5, "Public Documents"=6, "Public Application Data"=7, "Public Preferences"=8, "Public Cache"=13, "System Core Libraries"=9, "System Installed Libraries"=10, "Application Files"=11, "Boot Volume Root"=12] ("system directory type")
                n1412 = Search and Replace String(replace all?=TRUE ("replace all? (F)"), input string=w3538, search string="/") -> (result string=w3559:string)  [unwired: 5 in, 3 out]
                n1413 = Concatenate Strings(w3536, "TimeStamp;MeasureCh_Z(g);Ch_X(g);Ch_Y(g);INC_X(Deg)", "\n") -> (w3552:string)
                n1414 = call <vilib>:"Get System Directory.vi"("system directory type"=w3543) -> ("system directory"=w3553:path)  [unwired: 10 in]
                n1415 = Concatenate Strings(w3559, "_" ("string"), "S_E_T.csv") -> (w3560:string)
                n1416 = Build Path(base path=w3553, name or relative path="Logfile") -> (appended path=w3554:path)
                n1417 = call <vilib>:"Check if File or Folder Exists.vi"("path"=w3554) -> ("file or folder exists?"=w3555:bool, "dup path"=w3556:path)  [unwired: 8 in, 1 out]
                n1418 = case shown="False" w3555 {
                  tunnel: w3556 -> [w3582 w3583]
                  tunnel: [w3581 w3583] -> w3557
                  frame False {
                    n1419 = Create Folder(path (use dialog)=w3582) -> (created path=w3581:path)  [unwired: 2 in, 2 out]
                  }
                  frame True {
                  }
                }
                n1420 = Decimate 1D Array(w3579) -> (w3577:dbl[], w3576:dbl[], w3575:dbl[], w3573:dbl[])
                n1421 = for {
                  tunnel: [w3606] -> w3574 mode=indexing
                  tunnel: w3578 -> [w3601] mode=indexing
                  tunnel: w3577 -> [w3600] mode=indexing
                  tunnel: w3576 -> [w3599] mode=indexing
                  tunnel: w3575 -> [w3598] mode=indexing
                  tunnel: w3573 -> [w3597] mode=indexing
                  tunnel: [w3600] -> w3572 mode=indexing
                  tunnel: [w3599] -> w3571 mode=indexing
                  tunnel: [w3598] -> w3570 mode=indexing
                  tunnel: [w3597] -> w3569 mode=indexing
                  tunnel: w3568 -> [w3591]
                  tunnel: w3567 -> [w3590]
                  tunnel: w3566 -> [w3589] mode=indexing
                  tunnel: w3565 -> [w3588]
                  tunnel: [w3587] -> w3564
                  tunnel: [w3587] -> w3563
                  tunnel: [w3587] -> w3562
                  tunnel: [w3587] -> w3561
                  n1422 = Join Numbers(hi=w3591, lo=w3590) -> ((hi.lo)=w3594:u32)
                  n1423 = To Double Precision Float(number=w3589) -> (double precision float=w3595:dbl)
                  n1424 = Number To Decimal String(number=w3601) -> (decimal integer string=w3605:string)  [unwired: 1 in]
                  n1425 = Number To Fractional String(number=w3600, precision (6)=i16 3 ("width (-)")) -> (F-format string=w3607:string)  [unwired: 2 in]
                  n1426 = Number To Fractional String(number=w3599, precision (6)=i16 3 ("width (-)")) -> (F-format string=w3604:string)  [unwired: 2 in]
                  n1427 = Number To Fractional String(number=w3598, precision (6)=i16 3 ("width (-)")) -> (F-format string=w3603:string)  [unwired: 2 in]
                  n1428 = Number To Fractional String(number=w3597, precision (6)=i16 3 ("width (-)")) -> (F-format string=w3602:string)  [unwired: 2 in]
                  n1429 = Divide(x=w3595, y=w3588) -> (x/y=w3596:dbl)
                  n1430 = To Unsigned Quad Integer(1:w3594) -> (0:w3593:u64)
                  n1431 = Build Array(w3605, w3607, w3604, w3603, w3602) -> (w3606:string[])
                  n1432 = call "Unix Time to Timestamp.vi"("Fractional Second"=w3596, "Unix Time (s)"=w3593) -> ("Timestamp"=w3592:timestamp)  [unwired: 8 in, 1 out]
                  n1433 = To Double Precision Float(number=w3592) -> (double precision float=w3587:dbl)
                }
                n1434 = Build Path(base path=w3557, name or relative path=w3560) -> (appended path=w3558:path)
                n1435 = Open/Create/Replace File(file path (use dialog)=w3558, operation (0:open)=T10."open or create") -> (refnum out=w3551:refnum<file>, error out=w3549:errorcluster)  [unwired: 4 in, 1 out]
                n1436 = Write to Text File(file (use dialog)=w3551, text=w3552, error in=w3549) -> (refnum out=w3550:refnum<file>, error out=w3548:errorcluster)  [unwired: 1 in, 1 out]
                n1437 = Close File(refnum=w3550, error in=w3548) -> (path=w3537:path)  [unwired: 1 out]
              }
              frame 16 {
                w3616 = T13 2 items=["User Home"=0, "User Desktop"=1, "User Documents"=2, "User Application Data"=3, "User Preferences"=4, "User Temporary"=5, "Public Documents"=6, "Public Application Data"=7, "Public Preferences"=8, "Public Cache"=13, "System Core Libraries"=9, "System Installed Libraries"=10, "Application Files"=11, "Boot Volume Root"=12] ("system directory type")
                n1438 = Decimate 1D Array(w3643) -> (w3641:dbl[])
                n1439 = Search and Replace String(replace all?=TRUE ("replace all? (F)"), input string=w3611, search string="/") -> (result string=w3632:string)  [unwired: 5 in, 3 out]
                n1440 = for {
                  tunnel: [w3661] -> w3640 mode=indexing
                  tunnel: w3642 -> [w3659] mode=indexing
                  tunnel: w3641 -> [w3658] mode=indexing
                  tunnel: [w3658] -> w3639 mode=indexing
                  tunnel: w3638 -> [w3652]
                  tunnel: w3637 -> [w3651]
                  tunnel: w3636 -> [w3650] mode=indexing
                  tunnel: w3635 -> [w3649]
                  tunnel: [w3648] -> w3634
                  n1441 = Join Numbers(hi=w3652, lo=w3651) -> ((hi.lo)=w3655:u32)
                  n1442 = To Double Precision Float(number=w3650) -> (double precision float=w3656:dbl)
                  n1443 = Number To Decimal String(number=w3659) -> (decimal integer string=w3660:string)  [unwired: 1 in]
                  n1444 = Number To Fractional String(number=w3658, precision (6)=i16 3 ("width (-)")) -> (F-format string=w3662:string)  [unwired: 2 in]
                  n1445 = Divide(x=w3656, y=w3649) -> (x/y=w3657:dbl)
                  n1446 = To Unsigned Quad Integer(1:w3655) -> (0:w3654:u64)
                  n1447 = Build Array(w3660, w3662) -> (w3661:string[])
                  n1448 = call "Unix Time to Timestamp.vi"("Fractional Second"=w3657, "Unix Time (s)"=w3654) -> ("Timestamp"=w3653:timestamp)  [unwired: 8 in, 1 out]
                  n1449 = To Double Precision Float(number=w3653) -> (double precision float=w3648:dbl)
                }
                n1450 = Concatenate Strings(w3609, "TimeStamp;MeasureINC_Y(Deg)", "\n") -> (w3625:string)
                n1451 = call <vilib>:"Get System Directory.vi"("system directory type"=w3616) -> ("system directory"=w3626:path)  [unwired: 10 in]
                n1452 = Concatenate Strings(w3632, "_" ("string"), "S_E_T.csv") -> (w3633:string)
                n1453 = Build Path(base path=w3626, name or relative path="Logfile") -> (appended path=w3627:path)
                n1454 = call <vilib>:"Check if File or Folder Exists.vi"("path"=w3627) -> ("file or folder exists?"=w3628:bool, "dup path"=w3629:path)  [unwired: 8 in, 1 out]
                n1455 = case shown="False" w3628 {
                  tunnel: w3629 -> [w3646 w3647]
                  tunnel: [w3645 w3647] -> w3630
                  frame False {
                    n1456 = Create Folder(path (use dialog)=w3646) -> (created path=w3645:path)  [unwired: 2 in, 2 out]
                  }
                  frame True {
                  }
                }
                n1457 = Build Path(base path=w3630, name or relative path=w3633) -> (appended path=w3631:path)
                n1458 = Open/Create/Replace File(file path (use dialog)=w3631, operation (0:open)=T10."open or create") -> (refnum out=w3624:refnum<file>, error out=w3622:errorcluster)  [unwired: 4 in, 1 out]
                n1459 = Write to Text File(file (use dialog)=w3624, text=w3625, error in=w3622) -> (refnum out=w3623:refnum<file>, error out=w3621:errorcluster)  [unwired: 1 in, 1 out]
                n1460 = Close File(refnum=w3623, error in=w3621) -> (path=w3610:path)  [unwired: 1 out]
              }
              frame 17 {
                w3671 = T13 2 items=["User Home"=0, "User Desktop"=1, "User Documents"=2, "User Application Data"=3, "User Preferences"=4, "User Temporary"=5, "Public Documents"=6, "Public Application Data"=7, "Public Preferences"=8, "Public Cache"=13, "System Core Libraries"=9, "System Installed Libraries"=10, "Application Files"=11, "Boot Volume Root"=12] ("system directory type")
                n1461 = Decimate 1D Array(w3701) -> (w3697:dbl[], w3699:dbl[])
                n1462 = Search and Replace String(replace all?=TRUE ("replace all? (F)"), input string=w3666, search string="/") -> (result string=w3687:string)  [unwired: 5 in, 3 out]
                n1463 = for {
                  tunnel: [w3722] -> w3698 mode=indexing
                  tunnel: w3700 -> [w3720] mode=indexing
                  tunnel: w3697 -> [w3717] mode=indexing
                  tunnel: w3699 -> [w3716] mode=indexing
                  tunnel: [w3717] -> w3696 mode=indexing
                  tunnel: [w3716] -> w3695 mode=indexing
                  tunnel: w3694 -> [w3710]
                  tunnel: w3693 -> [w3709]
                  tunnel: w3692 -> [w3708] mode=indexing
                  tunnel: w3691 -> [w3707]
                  tunnel: [w3706] -> w3690
                  tunnel: [w3706] -> w3689
                  n1464 = Join Numbers(hi=w3710, lo=w3709) -> ((hi.lo)=w3713:u32)
                  n1465 = To Double Precision Float(number=w3708) -> (double precision float=w3714:dbl)
                  n1466 = Number To Decimal String(number=w3720) -> (decimal integer string=w3721:string)  [unwired: 1 in]
                  n1467 = Number To Fractional String(number=w3717, precision (6)=i16 3 ("width (-)")) -> (F-format string=w3723:string)  [unwired: 2 in]
                  n1468 = Number To Fractional String(number=w3716, precision (6)=i16 3 ("width (-)")) -> (F-format string=w3718:string)  [unwired: 2 in]
                  n1469 = Divide(x=w3714, y=w3707) -> (x/y=w3715:dbl)
                  n1470 = To Unsigned Quad Integer(1:w3713) -> (0:w3712:u64)
                  n1471 = Build Array(w3721, w3723, w3718) -> (w3722:string[])
                  n1472 = call "Unix Time to Timestamp.vi"("Fractional Second"=w3715, "Unix Time (s)"=w3712) -> ("Timestamp"=w3711:timestamp)  [unwired: 8 in, 1 out]
                  n1473 = To Double Precision Float(number=w3711) -> (double precision float=w3706:dbl)
                }
                n1474 = call <vilib>:"Get System Directory.vi"("system directory type"=w3671) -> ("system directory"=w3681:path)  [unwired: 10 in]
                n1475 = Concatenate Strings(w3687, "_" ("string"), "S_E_T.csv") -> (w3688:string)
                n1476 = Concatenate Strings(w3664, "TimeStamp;MeasureCh_Z(g);INC_Y(Deg)", "\n") -> (w3680:string)
                n1477 = Build Path(base path=w3681, name or relative path="Logfile") -> (appended path=w3682:path)
                n1478 = call <vilib>:"Check if File or Folder Exists.vi"("path"=w3682) -> ("file or folder exists?"=w3683:bool, "dup path"=w3684:path)  [unwired: 8 in, 1 out]
                n1479 = case shown="False" w3683 {
                  tunnel: w3684 -> [w3704 w3705]
                  tunnel: [w3703 w3705] -> w3685
                  frame False {
                    n1480 = Create Folder(path (use dialog)=w3704) -> (created path=w3703:path)  [unwired: 2 in, 2 out]
                  }
                  frame True {
                  }
                }
                n1481 = Build Path(base path=w3685, name or relative path=w3688) -> (appended path=w3686:path)
                n1482 = Open/Create/Replace File(file path (use dialog)=w3686, operation (0:open)=T10."open or create") -> (refnum out=w3679:refnum<file>, error out=w3677:errorcluster)  [unwired: 4 in, 1 out]
                n1483 = Write to Text File(file (use dialog)=w3679, text=w3680, error in=w3677) -> (refnum out=w3678:refnum<file>, error out=w3676:errorcluster)  [unwired: 1 in, 1 out]
                n1484 = Close File(refnum=w3678, error in=w3676) -> (path=w3665:path)  [unwired: 1 out]
              }
              frame 18 {
                w3732 = T13 2 items=["User Home"=0, "User Desktop"=1, "User Documents"=2, "User Application Data"=3, "User Preferences"=4, "User Temporary"=5, "Public Documents"=6, "Public Application Data"=7, "Public Preferences"=8, "Public Cache"=13, "System Core Libraries"=9, "System Installed Libraries"=10, "Application Files"=11, "Boot Volume Root"=12] ("system directory type")
                n1485 = Decimate 1D Array(w3761) -> (w3757:dbl[], w3759:dbl[])
                n1486 = Search and Replace String(replace all?=TRUE ("replace all? (F)"), input string=w3726, search string="/") -> (result string=w3748:string)  [unwired: 5 in, 3 out]
                n1487 = Concatenate Strings(w3725, "TimeStamp;MeasureCh_X(g);INC_Y(Deg)", "\n") -> (w3741:string)
                n1488 = for {
                  tunnel: [w3782] -> w3758 mode=indexing
                  tunnel: w3760 -> [w3778] mode=indexing
                  tunnel: w3757 -> [w3777] mode=indexing
                  tunnel: w3759 -> [w3776] mode=indexing
                  tunnel: [w3777] -> w3756 mode=indexing
                  tunnel: [w3776] -> w3755 mode=indexing
                  tunnel: w3754 -> [w3770]
                  tunnel: w3753 -> [w3769]
                  tunnel: w3752 -> [w3768] mode=indexing
                  tunnel: w3751 -> [w3767]
                  tunnel: [w3766] -> w3750
                  n1489 = Join Numbers(hi=w3770, lo=w3769) -> ((hi.lo)=w3773:u32)
                  n1490 = To Double Precision Float(number=w3768) -> (double precision float=w3774:dbl)
                  n1491 = Number To Decimal String(number=w3778) -> (decimal integer string=w3781:string)  [unwired: 1 in]
                  n1492 = Number To Fractional String(number=w3777, precision (6)=i16 3 ("width (-)")) -> (F-format string=w3783:string)  [unwired: 2 in]
                  n1493 = Number To Fractional String(number=w3776, precision (6)=i16 3 ("width (-)")) -> (F-format string=w3779:string)  [unwired: 2 in]
                  n1494 = Divide(x=w3774, y=w3767) -> (x/y=w3775:dbl)
                  n1495 = To Unsigned Quad Integer(1:w3773) -> (0:w3772:u64)
                  n1496 = Build Array(w3781, w3783, w3779) -> (w3782:string[])
                  n1497 = call "Unix Time to Timestamp.vi"("Fractional Second"=w3775, "Unix Time (s)"=w3772) -> ("Timestamp"=w3771:timestamp)  [unwired: 8 in, 1 out]
                  n1498 = To Double Precision Float(number=w3771) -> (double precision float=w3766:dbl)
                }
                n1499 = call <vilib>:"Get System Directory.vi"("system directory type"=w3732) -> ("system directory"=w3742:path)  [unwired: 10 in]
                n1500 = Concatenate Strings(w3748, "_" ("string"), "S_E_T.csv") -> (w3749:string)
                n1501 = Build Path(base path=w3742, name or relative path="Logfile") -> (appended path=w3743:path)
                n1502 = call <vilib>:"Check if File or Folder Exists.vi"("path"=w3743) -> ("file or folder exists?"=w3744:bool, "dup path"=w3745:path)  [unwired: 8 in, 1 out]
                n1503 = case shown="False" w3744 {
                  tunnel: w3745 -> [w3764 w3765]
                  tunnel: [w3763 w3765] -> w3746
                  frame False {
                    n1504 = Create Folder(path (use dialog)=w3764) -> (created path=w3763:path)  [unwired: 2 in, 2 out]
                  }
                  frame True {
                  }
                }
                n1505 = Build Path(base path=w3746, name or relative path=w3749) -> (appended path=w3747:path)
                n1506 = Open/Create/Replace File(file path (use dialog)=w3747, operation (0:open)=T10."open or create") -> (refnum out=w3740:refnum<file>, error out=w3738:errorcluster)  [unwired: 4 in, 1 out]
                n1507 = Write to Text File(file (use dialog)=w3740, text=w3741, error in=w3738) -> (refnum out=w3739:refnum<file>, error out=w3737:errorcluster)  [unwired: 1 in, 1 out]
                n1508 = Close File(refnum=w3739, error in=w3737) -> (path=w3727:path)  [unwired: 1 out]
              }
              frame 19 {
                w3792 = T13 2 items=["User Home"=0, "User Desktop"=1, "User Documents"=2, "User Application Data"=3, "User Preferences"=4, "User Temporary"=5, "Public Documents"=6, "Public Application Data"=7, "Public Preferences"=8, "Public Cache"=13, "System Core Libraries"=9, "System Installed Libraries"=10, "Application Files"=11, "Boot Volume Root"=12] ("system directory type")
                n1509 = Search and Replace String(replace all?=TRUE ("replace all? (F)"), input string=w3787, search string="/") -> (result string=w3808:string)  [unwired: 5 in, 3 out]
                n1510 = call <vilib>:"Get System Directory.vi"("system directory type"=w3792) -> ("system directory"=w3802:path)  [unwired: 10 in]
                n1511 = Concatenate Strings(w3808, "_" ("string"), "S_E_T.csv") -> (w3809:string)
                n1512 = Concatenate Strings(w3785, "TimeStamp;MeasureCh_Z(g);Ch_X(g);INC_Y(Deg)", "\n") -> (w3801:string)
                n1513 = Build Path(base path=w3802, name or relative path="Logfile") -> (appended path=w3803:path)
                n1514 = call <vilib>:"Check if File or Folder Exists.vi"("path"=w3803) -> ("file or folder exists?"=w3804:bool, "dup path"=w3805:path)  [unwired: 8 in, 1 out]
                n1515 = case shown="False" w3804 {
                  tunnel: w3805 -> [w3828 w3829]
                  tunnel: [w3827 w3829] -> w3806
                  frame False {
                    n1516 = Create Folder(path (use dialog)=w3828) -> (created path=w3827:path)  [unwired: 2 in, 2 out]
                  }
                  frame True {
                  }
                }
                n1517 = Decimate 1D Array(w3825) -> (w3821:dbl[], w3820:dbl[], w3823:dbl[])
                n1518 = for {
                  tunnel: [w3849] -> w3822 mode=indexing
                  tunnel: w3824 -> [w3843] mode=indexing
                  tunnel: w3821 -> [w3842] mode=indexing
                  tunnel: w3820 -> [w3841] mode=indexing
                  tunnel: w3823 -> [w3840] mode=indexing
                  tunnel: [w3842] -> w3819 mode=indexing
                  tunnel: [w3841] -> w3818 mode=indexing
                  tunnel: [w3840] -> w3817 mode=indexing
                  tunnel: w3816 -> [w3834]
                  tunnel: w3815 -> [w3833]
                  tunnel: w3814 -> [w3832] mode=indexing
                  tunnel: w3813 -> [w3831]
                  tunnel: [w3830] -> w3812
                  tunnel: [w3830] -> w3811
                  tunnel: [w3830] -> w3810
                  n1519 = Join Numbers(hi=w3834, lo=w3833) -> ((hi.lo)=w3837:u32)
                  n1520 = To Double Precision Float(number=w3832) -> (double precision float=w3838:dbl)
                  n1521 = Number To Decimal String(number=w3843) -> (decimal integer string=w3848:string)  [unwired: 1 in]
                  n1522 = Number To Fractional String(number=w3842, precision (6)=i16 3 ("width (-)")) -> (F-format string=w3850:string)  [unwired: 2 in]
                  n1523 = Number To Fractional String(number=w3841, precision (6)=i16 3 ("width (-)")) -> (F-format string=w3846:string)  [unwired: 2 in]
                  n1524 = Number To Fractional String(number=w3840, precision (6)=i16 3 ("width (-)")) -> (F-format string=w3844:string)  [unwired: 2 in]
                  n1525 = Divide(x=w3838, y=w3831) -> (x/y=w3839:dbl)
                  n1526 = To Unsigned Quad Integer(1:w3837) -> (0:w3836:u64)
                  n1527 = Build Array(w3848, w3850, w3846, w3844) -> (w3849:string[])
                  n1528 = call "Unix Time to Timestamp.vi"("Fractional Second"=w3839, "Unix Time (s)"=w3836) -> ("Timestamp"=w3835:timestamp)  [unwired: 8 in, 1 out]
                  n1529 = To Double Precision Float(number=w3835) -> (double precision float=w3830:dbl)
                }
                n1530 = Build Path(base path=w3806, name or relative path=w3809) -> (appended path=w3807:path)
                n1531 = Open/Create/Replace File(file path (use dialog)=w3807, operation (0:open)=T10."open or create") -> (refnum out=w3800:refnum<file>, error out=w3798:errorcluster)  [unwired: 4 in, 1 out]
                n1532 = Write to Text File(file (use dialog)=w3800, text=w3801, error in=w3798) -> (refnum out=w3799:refnum<file>, error out=w3797:errorcluster)  [unwired: 1 in, 1 out]
                n1533 = Close File(refnum=w3799, error in=w3797) -> (path=w3786:path)  [unwired: 1 out]
              }
              frame 20 {
                w3859 = T13 2 items=["User Home"=0, "User Desktop"=1, "User Documents"=2, "User Application Data"=3, "User Preferences"=4, "User Temporary"=5, "Public Documents"=6, "Public Application Data"=7, "Public Preferences"=8, "Public Cache"=13, "System Core Libraries"=9, "System Installed Libraries"=10, "Application Files"=11, "Boot Volume Root"=12] ("system directory type")
                n1534 = Decimate 1D Array(w3888) -> (w3884:dbl[], w3886:dbl[])
                n1535 = Search and Replace String(replace all?=TRUE ("replace all? (F)"), input string=w3853, search string="/") -> (result string=w3875:string)  [unwired: 5 in, 3 out]
                n1536 = for {
                  tunnel: [w3909] -> w3885 mode=indexing
                  tunnel: w3887 -> [w3905] mode=indexing
                  tunnel: w3884 -> [w3904] mode=indexing
                  tunnel: w3886 -> [w3903] mode=indexing
                  tunnel: [w3904] -> w3883 mode=indexing
                  tunnel: [w3903] -> w3882 mode=indexing
                  tunnel: w3881 -> [w3897]
                  tunnel: w3880 -> [w3896]
                  tunnel: w3879 -> [w3895] mode=indexing
                  tunnel: w3878 -> [w3894]
                  tunnel: [w3893] -> w3877
                  n1537 = Join Numbers(hi=w3897, lo=w3896) -> ((hi.lo)=w3900:u32)
                  n1538 = To Double Precision Float(number=w3895) -> (double precision float=w3901:dbl)
                  n1539 = Number To Decimal String(number=w3905) -> (decimal integer string=w3908:string)  [unwired: 1 in]
                  n1540 = Number To Fractional String(number=w3904, precision (6)=i16 3 ("width (-)")) -> (F-format string=w3910:string)  [unwired: 2 in]
                  n1541 = Number To Fractional String(number=w3903, precision (6)=i16 3 ("width (-)")) -> (F-format string=w3906:string)  [unwired: 2 in]
                  n1542 = Divide(x=w3901, y=w3894) -> (x/y=w3902:dbl)
                  n1543 = To Unsigned Quad Integer(1:w3900) -> (0:w3899:u64)
                  n1544 = Build Array(w3908, w3910, w3906) -> (w3909:string[])
                  n1545 = call "Unix Time to Timestamp.vi"("Fractional Second"=w3902, "Unix Time (s)"=w3899) -> ("Timestamp"=w3898:timestamp)  [unwired: 8 in, 1 out]
                  n1546 = To Double Precision Float(number=w3898) -> (double precision float=w3893:dbl)
                }
                n1547 = Concatenate Strings(w3852, "TimeStamp;MeasureCh_Y(g);INC_Y(Deg)", "\n") -> (w3868:string)
                n1548 = call <vilib>:"Get System Directory.vi"("system directory type"=w3859) -> ("system directory"=w3869:path)  [unwired: 10 in]
                n1549 = Concatenate Strings(w3875, "_" ("string"), "S_E_T.csv") -> (w3876:string)
                n1550 = Build Path(base path=w3869, name or relative path="Logfile") -> (appended path=w3870:path)
                n1551 = call <vilib>:"Check if File or Folder Exists.vi"("path"=w3870) -> ("file or folder exists?"=w3871:bool, "dup path"=w3872:path)  [unwired: 8 in, 1 out]
                n1552 = case shown="False" w3871 {
                  tunnel: w3872 -> [w3891 w3892]
                  tunnel: [w3890 w3892] -> w3873
                  frame False {
                    n1553 = Create Folder(path (use dialog)=w3891) -> (created path=w3890:path)  [unwired: 2 in, 2 out]
                  }
                  frame True {
                  }
                }
                n1554 = Build Path(base path=w3873, name or relative path=w3876) -> (appended path=w3874:path)
                n1555 = Open/Create/Replace File(file path (use dialog)=w3874, operation (0:open)=T10."open or create") -> (refnum out=w3867:refnum<file>, error out=w3865:errorcluster)  [unwired: 4 in, 1 out]
                n1556 = Write to Text File(file (use dialog)=w3867, text=w3868, error in=w3865) -> (refnum out=w3866:refnum<file>, error out=w3864:errorcluster)  [unwired: 1 in, 1 out]
                n1557 = Close File(refnum=w3866, error in=w3864) -> (path=w3854:path)  [unwired: 1 out]
              }
              frame 21 {
                w3919 = T13 2 items=["User Home"=0, "User Desktop"=1, "User Documents"=2, "User Application Data"=3, "User Preferences"=4, "User Temporary"=5, "Public Documents"=6, "Public Application Data"=7, "Public Preferences"=8, "Public Cache"=13, "System Core Libraries"=9, "System Installed Libraries"=10, "Application Files"=11, "Boot Volume Root"=12] ("system directory type")
                n1558 = Search and Replace String(replace all?=TRUE ("replace all? (F)"), input string=w3914, search string="/") -> (result string=w3935:string)  [unwired: 5 in, 3 out]
                n1559 = Concatenate Strings(w3912, "TimeStamp;MeasureCh_Z(g);Ch_Y(g);INC_Y(Deg)", "\n") -> (w3928:string)
                n1560 = call <vilib>:"Get System Directory.vi"("system directory type"=w3919) -> ("system directory"=w3929:path)  [unwired: 10 in]
                n1561 = Concatenate Strings(w3935, "_" ("string"), "S_E_T.csv") -> (w3936:string)
                n1562 = Build Path(base path=w3929, name or relative path="Logfile") -> (appended path=w3930:path)
                n1563 = call <vilib>:"Check if File or Folder Exists.vi"("path"=w3930) -> ("file or folder exists?"=w3931:bool, "dup path"=w3932:path)  [unwired: 8 in, 1 out]
                n1564 = case shown="False" w3931 {
                  tunnel: w3932 -> [w3955 w3956]
                  tunnel: [w3954 w3956] -> w3933
                  frame False {
                    n1565 = Create Folder(path (use dialog)=w3955) -> (created path=w3954:path)  [unwired: 2 in, 2 out]
                  }
                  frame True {
                  }
                }
                n1566 = Decimate 1D Array(w3952) -> (w3948:dbl[], w3947:dbl[], w3950:dbl[])
                n1567 = for {
                  tunnel: [w3976] -> w3949 mode=indexing
                  tunnel: w3951 -> [w3970] mode=indexing
                  tunnel: w3948 -> [w3969] mode=indexing
                  tunnel: w3947 -> [w3968] mode=indexing
                  tunnel: w3950 -> [w3967] mode=indexing
                  tunnel: [w3969] -> w3946 mode=indexing
                  tunnel: [w3968] -> w3945 mode=indexing
                  tunnel: [w3967] -> w3944 mode=indexing
                  tunnel: w3943 -> [w3961]
                  tunnel: w3942 -> [w3960]
                  tunnel: w3941 -> [w3959] mode=indexing
                  tunnel: w3940 -> [w3958]
                  tunnel: [w3957] -> w3939
                  tunnel: [w3957] -> w3938
                  tunnel: [w3957] -> w3937
                  n1568 = Join Numbers(hi=w3961, lo=w3960) -> ((hi.lo)=w3964:u32)
                  n1569 = To Double Precision Float(number=w3959) -> (double precision float=w3965:dbl)
                  n1570 = Number To Decimal String(number=w3970) -> (decimal integer string=w3975:string)  [unwired: 1 in]
                  n1571 = Number To Fractional String(number=w3969, precision (6)=i16 3 ("width (-)")) -> (F-format string=w3977:string)  [unwired: 2 in]
                  n1572 = Number To Fractional String(number=w3968, precision (6)=i16 3 ("width (-)")) -> (F-format string=w3973:string)  [unwired: 2 in]
                  n1573 = Number To Fractional String(number=w3967, precision (6)=i16 3 ("width (-)")) -> (F-format string=w3971:string)  [unwired: 2 in]
                  n1574 = Divide(x=w3965, y=w3958) -> (x/y=w3966:dbl)
                  n1575 = To Unsigned Quad Integer(1:w3964) -> (0:w3963:u64)
                  n1576 = Build Array(w3975, w3977, w3973, w3971) -> (w3976:string[])
                  n1577 = call "Unix Time to Timestamp.vi"("Fractional Second"=w3966, "Unix Time (s)"=w3963) -> ("Timestamp"=w3962:timestamp)  [unwired: 8 in, 1 out]
                  n1578 = To Double Precision Float(number=w3962) -> (double precision float=w3957:dbl)
                }
                n1579 = Build Path(base path=w3933, name or relative path=w3936) -> (appended path=w3934:path)
                n1580 = Open/Create/Replace File(file path (use dialog)=w3934, operation (0:open)=T10."open or create") -> (refnum out=w3927:refnum<file>, error out=w3925:errorcluster)  [unwired: 4 in, 1 out]
                n1581 = Write to Text File(file (use dialog)=w3927, text=w3928, error in=w3925) -> (refnum out=w3926:refnum<file>, error out=w3924:errorcluster)  [unwired: 1 in, 1 out]
                n1582 = Close File(refnum=w3926, error in=w3924) -> (path=w3913:path)  [unwired: 1 out]
              }
              frame 22 {
                w3986 = T13 2 items=["User Home"=0, "User Desktop"=1, "User Documents"=2, "User Application Data"=3, "User Preferences"=4, "User Temporary"=5, "Public Documents"=6, "Public Application Data"=7, "Public Preferences"=8, "Public Cache"=13, "System Core Libraries"=9, "System Installed Libraries"=10, "Application Files"=11, "Boot Volume Root"=12] ("system directory type")
                n1583 = Search and Replace String(replace all?=TRUE ("replace all? (F)"), input string=w3981, search string="/") -> (result string=w4002:string)  [unwired: 5 in, 3 out]
                n1584 = Concatenate Strings(w3979, "TimeStamp;MeasureCh_X(g);Ch_Y(g);INC_X(Deg)", "\n") -> (w3995:string)
                n1585 = call <vilib>:"Get System Directory.vi"("system directory type"=w3986) -> ("system directory"=w3996:path)  [unwired: 10 in]
                n1586 = Concatenate Strings(w4002, "_" ("string"), "S_E_T.csv") -> (w4003:string)
                n1587 = Build Path(base path=w3996, name or relative path="Logfile") -> (appended path=w3997:path)
                n1588 = call <vilib>:"Check if File or Folder Exists.vi"("path"=w3997) -> ("file or folder exists?"=w3998:bool, "dup path"=w3999:path)  [unwired: 8 in, 1 out]
                n1589 = case shown="False" w3998 {
                  tunnel: w3999 -> [w4022 w4023]
                  tunnel: [w4021 w4023] -> w4000
                  frame False {
                    n1590 = Create Folder(path (use dialog)=w4022) -> (created path=w4021:path)  [unwired: 2 in, 2 out]
                  }
                  frame True {
                  }
                }
                n1591 = Decimate 1D Array(w4019) -> (w4015:dbl[], w4014:dbl[], w4018:dbl[])
                n1592 = for {
                  tunnel: [w4043] -> w4016 mode=indexing
                  tunnel: w4017 -> [w4037] mode=indexing
                  tunnel: w4015 -> [w4036] mode=indexing
                  tunnel: w4014 -> [w4035] mode=indexing
                  tunnel: w4018 -> [w4034] mode=indexing
                  tunnel: [w4036] -> w4013 mode=indexing
                  tunnel: [w4035] -> w4012 mode=indexing
                  tunnel: [w4034] -> w4011 mode=indexing
                  tunnel: w4010 -> [w4028]
                  tunnel: w4009 -> [w4027]
                  tunnel: w4008 -> [w4026] mode=indexing
                  tunnel: w4007 -> [w4025]
                  tunnel: [w4024] -> w4006
                  tunnel: [w4024] -> w4005
                  tunnel: [w4024] -> w4004
                  n1593 = Join Numbers(hi=w4028, lo=w4027) -> ((hi.lo)=w4031:u32)
                  n1594 = To Double Precision Float(number=w4026) -> (double precision float=w4032:dbl)
                  n1595 = Number To Decimal String(number=w4037) -> (decimal integer string=w4042:string)  [unwired: 1 in]
                  n1596 = Number To Fractional String(number=w4036, precision (6)=i16 3 ("width (-)")) -> (F-format string=w4044:string)  [unwired: 2 in]
                  n1597 = Number To Fractional String(number=w4035, precision (6)=i16 3 ("width (-)")) -> (F-format string=w4040:string)  [unwired: 2 in]
                  n1598 = Number To Fractional String(number=w4034, precision (6)=i16 3 ("width (-)")) -> (F-format string=w4038:string)  [unwired: 2 in]
                  n1599 = Divide(x=w4032, y=w4025) -> (x/y=w4033:dbl)
                  n1600 = To Unsigned Quad Integer(1:w4031) -> (0:w4030:u64)
                  n1601 = Build Array(w4042, w4044, w4040, w4038) -> (w4043:string[])
                  n1602 = call "Unix Time to Timestamp.vi"("Fractional Second"=w4033, "Unix Time (s)"=w4030) -> ("Timestamp"=w4029:timestamp)  [unwired: 8 in, 1 out]
                  n1603 = To Double Precision Float(number=w4029) -> (double precision float=w4024:dbl)
                }
                n1604 = Build Path(base path=w4000, name or relative path=w4003) -> (appended path=w4001:path)
                n1605 = Open/Create/Replace File(file path (use dialog)=w4001, operation (0:open)=T10."open or create") -> (refnum out=w3994:refnum<file>, error out=w3992:errorcluster)  [unwired: 4 in, 1 out]
                n1606 = Write to Text File(file (use dialog)=w3994, text=w3995, error in=w3992) -> (refnum out=w3993:refnum<file>, error out=w3991:errorcluster)  [unwired: 1 in, 1 out]
                n1607 = Close File(refnum=w3993, error in=w3991) -> (path=w3980:path)  [unwired: 1 out]
              }
              frame 23 {
                w4053 = T13 2 items=["User Home"=0, "User Desktop"=1, "User Documents"=2, "User Application Data"=3, "User Preferences"=4, "User Temporary"=5, "Public Documents"=6, "Public Application Data"=7, "Public Preferences"=8, "Public Cache"=13, "System Core Libraries"=9, "System Installed Libraries"=10, "Application Files"=11, "Boot Volume Root"=12] ("system directory type")
                n1608 = Search and Replace String(replace all?=TRUE ("replace all? (F)"), input string=w4047, search string="/") -> (result string=w4069:string)  [unwired: 5 in, 3 out]
                n1609 = Concatenate Strings(w4046, "TimeStamp;MeasureCh_Z(g);Ch_X(g);Ch_Y(g);INC_Y(Deg)", "\n") -> (w4062:string)
                n1610 = call <vilib>:"Get System Directory.vi"("system directory type"=w4053) -> ("system directory"=w4063:path)  [unwired: 10 in]
                n1611 = Concatenate Strings(w4069, "_" ("string"), "S_E_T.csv") -> (w4070:string)
                n1612 = Build Path(base path=w4063, name or relative path="Logfile") -> (appended path=w4064:path)
                n1613 = call <vilib>:"Check if File or Folder Exists.vi"("path"=w4064) -> ("file or folder exists?"=w4065:bool, "dup path"=w4066:path)  [unwired: 8 in, 1 out]
                n1614 = Decimate 1D Array(w4086) -> (w4085:dbl[], w4084:dbl[], w4083:dbl[], w4080:dbl[])
                n1615 = case shown="False" w4065 {
                  tunnel: w4066 -> [w4089 w4090]
                  tunnel: [w4088 w4090] -> w4067
                  frame False {
                    n1616 = Create Folder(path (use dialog)=w4089) -> (created path=w4088:path)  [unwired: 2 in, 2 out]
                  }
                  frame True {
                  }
                }
                n1617 = for {
                  tunnel: [w4112] -> w4081 mode=indexing
                  tunnel: w4082 -> [w4106] mode=indexing
                  tunnel: w4085 -> [w4104] mode=indexing
                  tunnel: w4084 -> [w4103] mode=indexing
                  tunnel: w4083 -> [w4102] mode=indexing
                  tunnel: w4080 -> [w4101] mode=indexing
                  tunnel: [w4104] -> w4079 mode=indexing
                  tunnel: [w4103] -> w4078 mode=indexing
                  tunnel: [w4102] -> w4077 mode=indexing
                  tunnel: [w4101] -> w4076 mode=indexing
                  tunnel: w4075 -> [w4095]
                  tunnel: w4074 -> [w4094]
                  tunnel: w4073 -> [w4093] mode=indexing
                  tunnel: w4072 -> [w4092]
                  tunnel: [w4091] -> w4071
                  n1618 = Number To Fractional String(number=w4101, precision (6)=i16 3 ("width (-)")) -> ()  [unwired: 2 in, 1 out]
                  n1619 = Join Numbers(hi=w4095, lo=w4094) -> ((hi.lo)=w4098:u32)
                  n1620 = To Double Precision Float(number=w4093) -> (double precision float=w4099:dbl)
                  n1621 = Number To Decimal String(number=w4106) -> (decimal integer string=w4111:string)  [unwired: 1 in]
                  n1622 = Number To Fractional String(number=w4104, precision (6)=i16 3 ("width (-)")) -> (F-format string=w4113:string)  [unwired: 2 in]
                  n1623 = Number To Fractional String(number=w4103, precision (6)=i16 3 ("width (-)")) -> (F-format string=w4109:string)  [unwired: 2 in]
                  n1624 = Number To Fractional String(number=w4102, precision (6)=i16 3 ("width (-)")) -> (F-format string=w4107:string)  [unwired: 2 in]
                  n1625 = Divide(x=w4099, y=w4092) -> (x/y=w4100:dbl)
                  n1626 = To Unsigned Quad Integer(1:w4098) -> (0:w4097:u64)
                  n1627 = Build Array(w4111, w4113, w4109, w4107) -> (w4112:string[])
                  n1628 = call "Unix Time to Timestamp.vi"("Fractional Second"=w4100, "Unix Time (s)"=w4097) -> ("Timestamp"=w4096:timestamp)  [unwired: 8 in, 1 out]
                  n1629 = To Double Precision Float(number=w4096) -> (double precision float=w4091:dbl)
                }
                n1630 = Build Path(base path=w4067, name or relative path=w4070) -> (appended path=w4068:path)
                n1631 = Open/Create/Replace File(file path (use dialog)=w4068, operation (0:open)=T10."open or create") -> (refnum out=w4061:refnum<file>, error out=w4059:errorcluster)  [unwired: 4 in, 1 out]
                n1632 = Write to Text File(file (use dialog)=w4061, text=w4062, error in=w4059) -> (refnum out=w4060:refnum<file>, error out=w4058:errorcluster)  [unwired: 1 in, 1 out]
                n1633 = Close File(refnum=w4060, error in=w4058) -> (path=w4048:path)  [unwired: 1 out]
              }
              frame 24 {
                w4122 = T13 2 items=["User Home"=0, "User Desktop"=1, "User Documents"=2, "User Application Data"=3, "User Preferences"=4, "User Temporary"=5, "Public Documents"=6, "Public Application Data"=7, "Public Preferences"=8, "Public Cache"=13, "System Core Libraries"=9, "System Installed Libraries"=10, "Application Files"=11, "Boot Volume Root"=12] ("system directory type")
                n1634 = Decimate 1D Array(w4151) -> (w4149:dbl[], w4148:dbl[])
                n1635 = Search and Replace String(replace all?=TRUE ("replace all? (F)"), input string=w4117, search string="/") -> (result string=w4138:string)  [unwired: 5 in, 3 out]
                n1636 = Concatenate Strings(w4115, "TimeStamp;Measure INC_X(Deg);INC_Y(Deg)", "\n") -> (w4131:string)
                n1637 = for {
                  tunnel: [w4172] -> w4147 mode=indexing
                  tunnel: w4150 -> [w4168] mode=indexing
                  tunnel: w4149 -> [w4167] mode=indexing
                  tunnel: w4148 -> [w4166] mode=indexing
                  tunnel: [w4167] -> w4146 mode=indexing
                  tunnel: [w4166] -> w4145 mode=indexing
                  tunnel: w4144 -> [w4160]
                  tunnel: w4143 -> [w4159]
                  tunnel: w4142 -> [w4158] mode=indexing
                  tunnel: w4141 -> [w4157]
                  tunnel: [w4156] -> w4140
                  n1638 = Join Numbers(hi=w4160, lo=w4159) -> ((hi.lo)=w4163:u32)
                  n1639 = To Double Precision Float(number=w4158) -> (double precision float=w4164:dbl)
                  n1640 = Number To Decimal String(number=w4168) -> (decimal integer string=w4171:string)  [unwired: 1 in]
                  n1641 = Number To Fractional String(number=w4167, precision (6)=i16 3 ("width (-)")) -> (F-format string=w4173:string)  [unwired: 2 in]
                  n1642 = Number To Fractional String(number=w4166, precision (6)=i16 3 ("width (-)")) -> (F-format string=w4169:string)  [unwired: 2 in]
                  n1643 = Divide(x=w4164, y=w4157) -> (x/y=w4165:dbl)
                  n1644 = To Unsigned Quad Integer(1:w4163) -> (0:w4162:u64)
                  n1645 = Build Array(w4171, w4173, w4169) -> (w4172:string[])
                  n1646 = call "Unix Time to Timestamp.vi"("Fractional Second"=w4165, "Unix Time (s)"=w4162) -> ("Timestamp"=w4161:timestamp)  [unwired: 8 in, 1 out]
                  n1647 = To Double Precision Float(number=w4161) -> (double precision float=w4156:dbl)
                }
                n1648 = call <vilib>:"Get System Directory.vi"("system directory type"=w4122) -> ("system directory"=w4132:path)  [unwired: 10 in]
                n1649 = Concatenate Strings(w4138, "_" ("string"), "S_E_T.csv") -> (w4139:string)
                n1650 = Build Path(base path=w4132, name or relative path="Logfile") -> (appended path=w4133:path)
                n1651 = call <vilib>:"Check if File or Folder Exists.vi"("path"=w4133) -> ("file or folder exists?"=w4134:bool, "dup path"=w4135:path)  [unwired: 8 in, 1 out]
                n1652 = case shown="False" w4134 {
                  tunnel: w4135 -> [w4154 w4155]
                  tunnel: [w4153 w4155] -> w4136
                  frame False {
                    n1653 = Create Folder(path (use dialog)=w4154) -> (created path=w4153:path)  [unwired: 2 in, 2 out]
                  }
                  frame True {
                  }
                }
                n1654 = Build Path(base path=w4136, name or relative path=w4139) -> (appended path=w4137:path)
                n1655 = Open/Create/Replace File(file path (use dialog)=w4137, operation (0:open)=T10."open or create") -> (refnum out=w4130:refnum<file>, error out=w4128:errorcluster)  [unwired: 4 in, 1 out]
                n1656 = Write to Text File(file (use dialog)=w4130, text=w4131, error in=w4128) -> (refnum out=w4129:refnum<file>, error out=w4127:errorcluster)  [unwired: 1 in, 1 out]
                n1657 = Close File(refnum=w4129, error in=w4127) -> (path=w4116:path)  [unwired: 1 out]
              }
              frame 25 {
                w4182 = T13 2 items=["User Home"=0, "User Desktop"=1, "User Documents"=2, "User Application Data"=3, "User Preferences"=4, "User Temporary"=5, "Public Documents"=6, "Public Application Data"=7, "Public Preferences"=8, "Public Cache"=13, "System Core Libraries"=9, "System Installed Libraries"=10, "Application Files"=11, "Boot Volume Root"=12] ("system directory type")
                n1658 = Search and Replace String(replace all?=TRUE ("replace all? (F)"), input string=w4177, search string="/") -> (result string=w4198:string)  [unwired: 5 in, 3 out]
                n1659 = Concatenate Strings(w4175, "TimeStamp;Measure Ch_Z(g);INC_X(Deg);INC_Y(Deg)", "\n") -> (w4191:string)
                n1660 = call <vilib>:"Get System Directory.vi"("system directory type"=w4182) -> ("system directory"=w4192:path)  [unwired: 10 in]
                n1661 = Concatenate Strings(w4198, "_" ("string"), "S_E_T.csv") -> (w4199:string)
                n1662 = Build Path(base path=w4192, name or relative path="Logfile") -> (appended path=w4193:path)
                n1663 = call <vilib>:"Check if File or Folder Exists.vi"("path"=w4193) -> ("file or folder exists?"=w4194:bool, "dup path"=w4195:path)  [unwired: 8 in, 1 out]
                n1664 = case shown="False" w4194 {
                  tunnel: w4195 -> [w4216 w4217]
                  tunnel: [w4215 w4217] -> w4196
                  frame False {
                    n1665 = Create Folder(path (use dialog)=w4216) -> (created path=w4215:path)  [unwired: 2 in, 2 out]
                  }
                  frame True {
                  }
                }
                n1666 = Decimate 1D Array(w4213) -> (w4208:dbl[], w4211:dbl[], w4210:dbl[])
                n1667 = for {
                  tunnel: [w4237] -> w4209 mode=indexing
                  tunnel: w4212 -> [w4231] mode=indexing
                  tunnel: w4208 -> [w4230] mode=indexing
                  tunnel: w4211 -> [w4229] mode=indexing
                  tunnel: w4210 -> [w4228] mode=indexing
                  tunnel: [w4230] -> w4207 mode=indexing
                  tunnel: [w4229] -> w4206 mode=indexing
                  tunnel: [w4228] -> w4205 mode=indexing
                  tunnel: w4204 -> [w4222]
                  tunnel: w4203 -> [w4221]
                  tunnel: w4202 -> [w4220] mode=indexing
                  tunnel: w4201 -> [w4219]
                  tunnel: [w4218] -> w4200
                  n1668 = Join Numbers(hi=w4222, lo=w4221) -> ((hi.lo)=w4225:u32)
                  n1669 = To Double Precision Float(number=w4220) -> (double precision float=w4226:dbl)
                  n1670 = Number To Decimal String(number=w4231) -> (decimal integer string=w4236:string)  [unwired: 1 in]
                  n1671 = Number To Fractional String(number=w4230, precision (6)=i16 3 ("width (-)")) -> (F-format string=w4238:string)  [unwired: 2 in]
                  n1672 = Number To Fractional String(number=w4229, precision (6)=i16 3 ("width (-)")) -> (F-format string=w4234:string)  [unwired: 2 in]
                  n1673 = Number To Fractional String(number=w4228, precision (6)=i16 3 ("width (-)")) -> (F-format string=w4232:string)  [unwired: 2 in]
                  n1674 = Divide(x=w4226, y=w4219) -> (x/y=w4227:dbl)
                  n1675 = To Unsigned Quad Integer(1:w4225) -> (0:w4224:u64)
                  n1676 = Build Array(w4236, w4238, w4234, w4232) -> (w4237:string[])
                  n1677 = call "Unix Time to Timestamp.vi"("Fractional Second"=w4227, "Unix Time (s)"=w4224) -> ("Timestamp"=w4223:timestamp)  [unwired: 8 in, 1 out]
                  n1678 = To Double Precision Float(number=w4223) -> (double precision float=w4218:dbl)
                }
                n1679 = Build Path(base path=w4196, name or relative path=w4199) -> (appended path=w4197:path)
                n1680 = Open/Create/Replace File(file path (use dialog)=w4197, operation (0:open)=T10."open or create") -> (refnum out=w4190:refnum<file>, error out=w4188:errorcluster)  [unwired: 4 in, 1 out]
                n1681 = Write to Text File(file (use dialog)=w4190, text=w4191, error in=w4188) -> (refnum out=w4189:refnum<file>, error out=w4187:errorcluster)  [unwired: 1 in, 1 out]
                n1682 = Close File(refnum=w4189, error in=w4187) -> (path=w4176:path)  [unwired: 1 out]
              }
              frame 26 {
                w4247 = T13 2 items=["User Home"=0, "User Desktop"=1, "User Documents"=2, "User Application Data"=3, "User Preferences"=4, "User Temporary"=5, "Public Documents"=6, "Public Application Data"=7, "Public Preferences"=8, "Public Cache"=13, "System Core Libraries"=9, "System Installed Libraries"=10, "Application Files"=11, "Boot Volume Root"=12] ("system directory type")
                n1683 = Search and Replace String(replace all?=TRUE ("replace all? (F)"), input string=w4242, search string="/") -> (result string=w4263:string)  [unwired: 5 in, 3 out]
                n1684 = Concatenate Strings(w4240, "TimeStamp;Measure Ch_X(g);INC_X(Deg);INC_Y(Deg)", "\n") -> (w4256:string)
                n1685 = call <vilib>:"Get System Directory.vi"("system directory type"=w4247) -> ("system directory"=w4257:path)  [unwired: 10 in]
                n1686 = Concatenate Strings(w4263, "_" ("string"), "S_E_T.csv") -> (w4264:string)
                n1687 = Build Path(base path=w4257, name or relative path="Logfile") -> (appended path=w4258:path)
                n1688 = call <vilib>:"Check if File or Folder Exists.vi"("path"=w4258) -> ("file or folder exists?"=w4259:bool, "dup path"=w4260:path)  [unwired: 8 in, 1 out]
                n1689 = case shown="False" w4259 {
                  tunnel: w4260 -> [w4281 w4282]
                  tunnel: [w4280 w4282] -> w4261
                  frame False {
                    n1690 = Create Folder(path (use dialog)=w4281) -> (created path=w4280:path)  [unwired: 2 in, 2 out]
                  }
                  frame True {
                  }
                }
                n1691 = Decimate 1D Array(w4278) -> (w4273:dbl[], w4277:dbl[], w4276:dbl[])
                n1692 = for {
                  tunnel: [w4302] -> w4274 mode=indexing
                  tunnel: w4275 -> [w4296] mode=indexing
                  tunnel: w4273 -> [w4295] mode=indexing
                  tunnel: w4277 -> [w4294] mode=indexing
                  tunnel: w4276 -> [w4293] mode=indexing
                  tunnel: [w4295] -> w4272 mode=indexing
                  tunnel: [w4294] -> w4271 mode=indexing
                  tunnel: [w4293] -> w4270 mode=indexing
                  tunnel: w4269 -> [w4287]
                  tunnel: w4268 -> [w4286]
                  tunnel: w4267 -> [w4285] mode=indexing
                  tunnel: w4266 -> [w4284]
                  tunnel: [w4283] -> w4265
                  n1693 = Join Numbers(hi=w4287, lo=w4286) -> ((hi.lo)=w4290:u32)
                  n1694 = To Double Precision Float(number=w4285) -> (double precision float=w4291:dbl)
                  n1695 = Number To Decimal String(number=w4296) -> (decimal integer string=w4301:string)  [unwired: 1 in]
                  n1696 = Number To Fractional String(number=w4295, precision (6)=i16 3 ("width (-)")) -> (F-format string=w4303:string)  [unwired: 2 in]
                  n1697 = Number To Fractional String(number=w4294, precision (6)=i16 3 ("width (-)")) -> (F-format string=w4299:string)  [unwired: 2 in]
                  n1698 = Number To Fractional String(number=w4293, precision (6)=i16 3 ("width (-)")) -> (F-format string=w4297:string)  [unwired: 2 in]
                  n1699 = Divide(x=w4291, y=w4284) -> (x/y=w4292:dbl)
                  n1700 = To Unsigned Quad Integer(1:w4290) -> (0:w4289:u64)
                  n1701 = Build Array(w4301, w4303, w4299, w4297) -> (w4302:string[])
                  n1702 = call "Unix Time to Timestamp.vi"("Fractional Second"=w4292, "Unix Time (s)"=w4289) -> ("Timestamp"=w4288:timestamp)  [unwired: 8 in, 1 out]
                  n1703 = To Double Precision Float(number=w4288) -> (double precision float=w4283:dbl)
                }
                n1704 = Build Path(base path=w4261, name or relative path=w4264) -> (appended path=w4262:path)
                n1705 = Open/Create/Replace File(file path (use dialog)=w4262, operation (0:open)=T10."open or create") -> (refnum out=w4255:refnum<file>, error out=w4253:errorcluster)  [unwired: 4 in, 1 out]
                n1706 = Write to Text File(file (use dialog)=w4255, text=w4256, error in=w4253) -> (refnum out=w4254:refnum<file>, error out=w4252:errorcluster)  [unwired: 1 in, 1 out]
                n1707 = Close File(refnum=w4254, error in=w4252) -> (path=w4241:path)  [unwired: 1 out]
              }
              frame 27 {
                w4312 = T13 2 items=["User Home"=0, "User Desktop"=1, "User Documents"=2, "User Application Data"=3, "User Preferences"=4, "User Temporary"=5, "Public Documents"=6, "Public Application Data"=7, "Public Preferences"=8, "Public Cache"=13, "System Core Libraries"=9, "System Installed Libraries"=10, "Application Files"=11, "Boot Volume Root"=12] ("system directory type")
                n1708 = Search and Replace String(replace all?=TRUE ("replace all? (F)"), input string=w4307, search string="/") -> (result string=w4328:string)  [unwired: 5 in, 3 out]
                n1709 = Concatenate Strings(w4305, "TimeStamp;Measure Ch_Z(g);Ch_X(g);INC_X(Deg);INC_Y(Deg)", "\n") -> (w4321:string)
                n1710 = call <vilib>:"Get System Directory.vi"("system directory type"=w4312) -> ("system directory"=w4322:path)  [unwired: 10 in]
                n1711 = Concatenate Strings(w4328, "_" ("string"), "S_E_T.csv") -> (w4329:string)
                n1712 = Build Path(base path=w4322, name or relative path="Logfile") -> (appended path=w4323:path)
                n1713 = call <vilib>:"Check if File or Folder Exists.vi"("path"=w4323) -> ("file or folder exists?"=w4324:bool, "dup path"=w4325:path)  [unwired: 8 in, 1 out]
                n1714 = case shown="False" w4324 {
                  tunnel: w4325 -> [w4348 w4349]
                  tunnel: [w4347 w4349] -> w4326
                  frame False {
                    n1715 = Create Folder(path (use dialog)=w4348) -> (created path=w4347:path)  [unwired: 2 in, 2 out]
                  }
                  frame True {
                  }
                }
                n1716 = Decimate 1D Array(w4345) -> (w4343:dbl[], w4342:dbl[], w4340:dbl[], w4339:dbl[])
                n1717 = for {
                  tunnel: [w4372] -> w4344 mode=indexing
                  tunnel: w4341 -> [w4366] mode=indexing
                  tunnel: w4343 -> [w4363] mode=indexing
                  tunnel: w4342 -> [w4362] mode=indexing
                  tunnel: w4340 -> [w4361] mode=indexing
                  tunnel: w4339 -> [w4360] mode=indexing
                  tunnel: [w4363] -> w4338 mode=indexing
                  tunnel: [w4362] -> w4337 mode=indexing
                  tunnel: [w4361] -> w4336 mode=indexing
                  tunnel: [w4360] -> w4335 mode=indexing
                  tunnel: w4334 -> [w4354]
                  tunnel: w4333 -> [w4353]
                  tunnel: w4332 -> [w4352] mode=indexing
                  tunnel: w4331 -> [w4351]
                  tunnel: [w4350] -> w4330
                  n1718 = Join Numbers(hi=w4354, lo=w4353) -> ((hi.lo)=w4357:u32)
                  n1719 = To Double Precision Float(number=w4352) -> (double precision float=w4358:dbl)
                  n1720 = Number To Decimal String(number=w4366) -> (decimal integer string=w4371:string)  [unwired: 1 in]
                  n1721 = Number To Fractional String(number=w4363, precision (6)=i16 3 ("width (-)")) -> (F-format string=w4373:string)  [unwired: 2 in]
                  n1722 = Number To Fractional String(number=w4362, precision (6)=i16 3 ("width (-)")) -> (F-format string=w4369:string)  [unwired: 2 in]
                  n1723 = Number To Fractional String(number=w4361, precision (6)=i16 3 ("width (-)")) -> (F-format string=w4367:string)  [unwired: 2 in]
                  n1724 = Number To Fractional String(number=w4360, precision (6)=i16 3 ("width (-)")) -> (F-format string=w4364:string)  [unwired: 2 in]
                  n1725 = Divide(x=w4358, y=w4351) -> (x/y=w4359:dbl)
                  n1726 = To Unsigned Quad Integer(1:w4357) -> (0:w4356:u64)
                  n1727 = Build Array(w4371, w4373, w4369, w4367, w4364) -> (w4372:string[])
                  n1728 = call "Unix Time to Timestamp.vi"("Fractional Second"=w4359, "Unix Time (s)"=w4356) -> ("Timestamp"=w4355:timestamp)  [unwired: 8 in, 1 out]
                  n1729 = To Double Precision Float(number=w4355) -> (double precision float=w4350:dbl)
                }
                n1730 = Build Path(base path=w4326, name or relative path=w4329) -> (appended path=w4327:path)
                n1731 = Open/Create/Replace File(file path (use dialog)=w4327, operation (0:open)=T10."open or create") -> (refnum out=w4320:refnum<file>, error out=w4318:errorcluster)  [unwired: 4 in, 1 out]
                n1732 = Write to Text File(file (use dialog)=w4320, text=w4321, error in=w4318) -> (refnum out=w4319:refnum<file>, error out=w4317:errorcluster)  [unwired: 1 in, 1 out]
                n1733 = Close File(refnum=w4319, error in=w4317) -> (path=w4306:path)  [unwired: 1 out]
              }
              frame 28 {
                w4382 = T13 2 items=["User Home"=0, "User Desktop"=1, "User Documents"=2, "User Application Data"=3, "User Preferences"=4, "User Temporary"=5, "Public Documents"=6, "Public Application Data"=7, "Public Preferences"=8, "Public Cache"=13, "System Core Libraries"=9, "System Installed Libraries"=10, "Application Files"=11, "Boot Volume Root"=12] ("system directory type")
                n1734 = Search and Replace String(replace all?=TRUE ("replace all? (F)"), input string=w4377, search string="/") -> (result string=w4398:string)  [unwired: 5 in, 3 out]
                n1735 = Concatenate Strings(w4375, "TimeStamp;Measure Ch_Y(g);INC_X(Deg);INC_Y(Deg)", "\n") -> (w4391:string)
                n1736 = call <vilib>:"Get System Directory.vi"("system directory type"=w4382) -> ("system directory"=w4392:path)  [unwired: 10 in]
                n1737 = Concatenate Strings(w4398, "_" ("string"), "S_E_T.csv") -> (w4399:string)
                n1738 = Build Path(base path=w4392, name or relative path="Logfile") -> (appended path=w4393:path)
                n1739 = call <vilib>:"Check if File or Folder Exists.vi"("path"=w4393) -> ("file or folder exists?"=w4394:bool, "dup path"=w4395:path)  [unwired: 8 in, 1 out]
                n1740 = case shown="False" w4394 {
                  tunnel: w4395 -> [w4416 w4417]
                  tunnel: [w4415 w4417] -> w4396
                  frame False {
                    n1741 = Create Folder(path (use dialog)=w4416) -> (created path=w4415:path)  [unwired: 2 in, 2 out]
                  }
                  frame True {
                  }
                }
                n1742 = Decimate 1D Array(w4413) -> (w4411:dbl[], w4410:dbl[], w4409:dbl[])
                n1743 = for {
                  tunnel: [w4437] -> w4408 mode=indexing
                  tunnel: w4412 -> [w4431] mode=indexing
                  tunnel: w4411 -> [w4430] mode=indexing
                  tunnel: w4410 -> [w4429] mode=indexing
                  tunnel: w4409 -> [w4428] mode=indexing
                  tunnel: [w4430] -> w4407 mode=indexing
                  tunnel: [w4429] -> w4406 mode=indexing
                  tunnel: [w4428] -> w4405 mode=indexing
                  tunnel: w4404 -> [w4422]
                  tunnel: w4403 -> [w4421]
                  tunnel: w4402 -> [w4420] mode=indexing
                  tunnel: w4401 -> [w4419]
                  tunnel: [w4418] -> w4400
                  n1744 = Join Numbers(hi=w4422, lo=w4421) -> ((hi.lo)=w4425:u32)
                  n1745 = To Double Precision Float(number=w4420) -> (double precision float=w4426:dbl)
                  n1746 = Number To Decimal String(number=w4431) -> (decimal integer string=w4436:string)  [unwired: 1 in]
                  n1747 = Number To Fractional String(number=w4430, precision (6)=i16 3 ("width (-)")) -> (F-format string=w4438:string)  [unwired: 2 in]
                  n1748 = Number To Fractional String(number=w4429, precision (6)=i16 3 ("width (-)")) -> (F-format string=w4434:string)  [unwired: 2 in]
                  n1749 = Number To Fractional String(number=w4428, precision (6)=i16 3 ("width (-)")) -> (F-format string=w4432:string)  [unwired: 2 in]
                  n1750 = Divide(x=w4426, y=w4419) -> (x/y=w4427:dbl)
                  n1751 = To Unsigned Quad Integer(1:w4425) -> (0:w4424:u64)
                  n1752 = Build Array(w4436, w4438, w4434, w4432) -> (w4437:string[])
                  n1753 = call "Unix Time to Timestamp.vi"("Fractional Second"=w4427, "Unix Time (s)"=w4424) -> ("Timestamp"=w4423:timestamp)  [unwired: 8 in, 1 out]
                  n1754 = To Double Precision Float(number=w4423) -> (double precision float=w4418:dbl)
                }
                n1755 = Build Path(base path=w4396, name or relative path=w4399) -> (appended path=w4397:path)
                n1756 = Open/Create/Replace File(file path (use dialog)=w4397, operation (0:open)=T10."open or create") -> (refnum out=w4390:refnum<file>, error out=w4388:errorcluster)  [unwired: 4 in, 1 out]
                n1757 = Write to Text File(file (use dialog)=w4390, text=w4391, error in=w4388) -> (refnum out=w4389:refnum<file>, error out=w4387:errorcluster)  [unwired: 1 in, 1 out]
                n1758 = Close File(refnum=w4389, error in=w4387) -> (path=w4376:path)  [unwired: 1 out]
              }
              frame 29 {
                w4447 = T13 2 items=["User Home"=0, "User Desktop"=1, "User Documents"=2, "User Application Data"=3, "User Preferences"=4, "User Temporary"=5, "Public Documents"=6, "Public Application Data"=7, "Public Preferences"=8, "Public Cache"=13, "System Core Libraries"=9, "System Installed Libraries"=10, "Application Files"=11, "Boot Volume Root"=12] ("system directory type")
                n1759 = Search and Replace String(replace all?=TRUE ("replace all? (F)"), input string=w4442, search string="/") -> (result string=w4463:string)  [unwired: 5 in, 3 out]
                n1760 = Concatenate Strings(w4440, "TimeStamp;Measure Ch_Z(g);Ch_Y(g);INC_X(Deg);INC_Y(Deg)", "\n") -> (w4456:string)
                n1761 = call <vilib>:"Get System Directory.vi"("system directory type"=w4447) -> ("system directory"=w4457:path)  [unwired: 10 in]
                n1762 = Concatenate Strings(w4463, "_" ("string"), "S_E_T.csv") -> (w4464:string)
                n1763 = Build Path(base path=w4457, name or relative path="Logfile") -> (appended path=w4458:path)
                n1764 = call <vilib>:"Check if File or Folder Exists.vi"("path"=w4458) -> ("file or folder exists?"=w4459:bool, "dup path"=w4460:path)  [unwired: 8 in, 1 out]
                n1765 = case shown="False" w4459 {
                  tunnel: w4460 -> [w4483 w4484]
                  tunnel: [w4482 w4484] -> w4461
                  frame False {
                    n1766 = Create Folder(path (use dialog)=w4483) -> (created path=w4482:path)  [unwired: 2 in, 2 out]
                  }
                  frame True {
                  }
                }
                n1767 = Decimate 1D Array(w4480) -> (w4474:dbl[], w4478:dbl[], w4475:dbl[], w4476:dbl[])
                n1768 = for {
                  tunnel: [w4507] -> w4477 mode=indexing
                  tunnel: w4479 -> [w4501] mode=indexing
                  tunnel: w4474 -> [w4498] mode=indexing
                  tunnel: w4478 -> [w4497] mode=indexing
                  tunnel: w4475 -> [w4496] mode=indexing
                  tunnel: w4476 -> [w4495] mode=indexing
                  tunnel: [w4498] -> w4473 mode=indexing
                  tunnel: [w4497] -> w4472 mode=indexing
                  tunnel: [w4496] -> w4471 mode=indexing
                  tunnel: [w4495] -> w4470 mode=indexing
                  tunnel: w4469 -> [w4489]
                  tunnel: w4468 -> [w4488]
                  tunnel: w4467 -> [w4487] mode=indexing
                  tunnel: w4466 -> [w4486]
                  tunnel: [w4485] -> w4465
                  n1769 = Join Numbers(hi=w4489, lo=w4488) -> ((hi.lo)=w4492:u32)
                  n1770 = To Double Precision Float(number=w4487) -> (double precision float=w4493:dbl)
                  n1771 = Number To Decimal String(number=w4501) -> (decimal integer string=w4506:string)  [unwired: 1 in]
                  n1772 = Number To Fractional String(number=w4498, precision (6)=i16 3 ("width (-)")) -> (F-format string=w4508:string)  [unwired: 2 in]
                  n1773 = Number To Fractional String(number=w4497, precision (6)=i16 3 ("width (-)")) -> (F-format string=w4504:string)  [unwired: 2 in]
                  n1774 = Number To Fractional String(number=w4496, precision (6)=i16 3 ("width (-)")) -> (F-format string=w4502:string)  [unwired: 2 in]
                  n1775 = Number To Fractional String(number=w4495, precision (6)=i16 3 ("width (-)")) -> (F-format string=w4499:string)  [unwired: 2 in]
                  n1776 = Divide(x=w4493, y=w4486) -> (x/y=w4494:dbl)
                  n1777 = To Unsigned Quad Integer(1:w4492) -> (0:w4491:u64)
                  n1778 = Build Array(w4506, w4508, w4504, w4502, w4499) -> (w4507:string[])
                  n1779 = call "Unix Time to Timestamp.vi"("Fractional Second"=w4494, "Unix Time (s)"=w4491) -> ("Timestamp"=w4490:timestamp)  [unwired: 8 in, 1 out]
                  n1780 = To Double Precision Float(number=w4490) -> (double precision float=w4485:dbl)
                }
                n1781 = Build Path(base path=w4461, name or relative path=w4464) -> (appended path=w4462:path)
                n1782 = Open/Create/Replace File(file path (use dialog)=w4462, operation (0:open)=T10."open or create") -> (refnum out=w4455:refnum<file>, error out=w4453:errorcluster)  [unwired: 4 in, 1 out]
                n1783 = Write to Text File(file (use dialog)=w4455, text=w4456, error in=w4453) -> (refnum out=w4454:refnum<file>, error out=w4452:errorcluster)  [unwired: 1 in, 1 out]
                n1784 = Close File(refnum=w4454, error in=w4452) -> (path=w4441:path)  [unwired: 1 out]
              }
              frame 30 {
                w4517 = T13 2 items=["User Home"=0, "User Desktop"=1, "User Documents"=2, "User Application Data"=3, "User Preferences"=4, "User Temporary"=5, "Public Documents"=6, "Public Application Data"=7, "Public Preferences"=8, "Public Cache"=13, "System Core Libraries"=9, "System Installed Libraries"=10, "Application Files"=11, "Boot Volume Root"=12] ("system directory type")
                n1785 = Search and Replace String(replace all?=TRUE ("replace all? (F)"), input string=w4512, search string="/") -> (result string=w4533:string)  [unwired: 5 in, 3 out]
                n1786 = Concatenate Strings(w4510, "TimeStamp;Measure Ch_X(g);Ch_Y(g);INC_X(Deg);INC_Y(Deg)", "\n") -> (w4526:string)
                n1787 = call <vilib>:"Get System Directory.vi"("system directory type"=w4517) -> ("system directory"=w4527:path)  [unwired: 10 in]
                n1788 = Concatenate Strings(w4533, "_" ("string"), "S_E_T.csv") -> (w4534:string)
                n1789 = Build Path(base path=w4527, name or relative path="Logfile") -> (appended path=w4528:path)
                n1790 = call <vilib>:"Check if File or Folder Exists.vi"("path"=w4528) -> ("file or folder exists?"=w4529:bool, "dup path"=w4530:path)  [unwired: 8 in, 1 out]
                n1791 = case shown="False" w4529 {
                  tunnel: w4530 -> [w4553 w4554]
                  tunnel: [w4552 w4554] -> w4531
                  frame False {
                    n1792 = Create Folder(path (use dialog)=w4553) -> (created path=w4552:path)  [unwired: 2 in, 2 out]
                  }
                  frame True {
                  }
                }
                n1793 = Decimate 1D Array(w4550) -> (w4549:dbl[], w4547:dbl[], w4545:dbl[], w4546:dbl[])
                n1794 = for {
                  tunnel: [w4577] -> w4544 mode=indexing
                  tunnel: w4548 -> [w4571] mode=indexing
                  tunnel: w4549 -> [w4568] mode=indexing
                  tunnel: w4547 -> [w4567] mode=indexing
                  tunnel: w4545 -> [w4566] mode=indexing
                  tunnel: w4546 -> [w4565] mode=indexing
                  tunnel: [w4568] -> w4543 mode=indexing
                  tunnel: [w4567] -> w4542 mode=indexing
                  tunnel: [w4566] -> w4541 mode=indexing
                  tunnel: [w4565] -> w4540 mode=indexing
                  tunnel: w4539 -> [w4559]
                  tunnel: w4538 -> [w4558]
                  tunnel: w4537 -> [w4557] mode=indexing
                  tunnel: w4536 -> [w4556]
                  tunnel: [w4555] -> w4535
                  n1795 = Join Numbers(hi=w4559, lo=w4558) -> ((hi.lo)=w4562:u32)
                  n1796 = To Double Precision Float(number=w4557) -> (double precision float=w4563:dbl)
                  n1797 = Number To Decimal String(number=w4571) -> (decimal integer string=w4576:string)  [unwired: 1 in]
                  n1798 = Number To Fractional String(number=w4568, precision (6)=i16 3 ("width (-)")) -> (F-format string=w4578:string)  [unwired: 2 in]
                  n1799 = Number To Fractional String(number=w4567, precision (6)=i16 3 ("width (-)")) -> (F-format string=w4574:string)  [unwired: 2 in]
                  n1800 = Number To Fractional String(number=w4566, precision (6)=i16 3 ("width (-)")) -> (F-format string=w4572:string)  [unwired: 2 in]
                  n1801 = Number To Fractional String(number=w4565, precision (6)=i16 3 ("width (-)")) -> (F-format string=w4569:string)  [unwired: 2 in]
                  n1802 = Divide(x=w4563, y=w4556) -> (x/y=w4564:dbl)
                  n1803 = To Unsigned Quad Integer(1:w4562) -> (0:w4561:u64)
                  n1804 = Build Array(w4576, w4578, w4574, w4572, w4569) -> (w4577:string[])
                  n1805 = call "Unix Time to Timestamp.vi"("Fractional Second"=w4564, "Unix Time (s)"=w4561) -> ("Timestamp"=w4560:timestamp)  [unwired: 8 in, 1 out]
                  n1806 = To Double Precision Float(number=w4560) -> (double precision float=w4555:dbl)
                }
                n1807 = Build Path(base path=w4531, name or relative path=w4534) -> (appended path=w4532:path)
                n1808 = Open/Create/Replace File(file path (use dialog)=w4532, operation (0:open)=T10."open or create") -> (refnum out=w4525:refnum<file>, error out=w4523:errorcluster)  [unwired: 4 in, 1 out]
                n1809 = Write to Text File(file (use dialog)=w4525, text=w4526, error in=w4523) -> (refnum out=w4524:refnum<file>, error out=w4522:errorcluster)  [unwired: 1 in, 1 out]
                n1810 = Close File(refnum=w4524, error in=w4522) -> (path=w4511:path)  [unwired: 1 out]
              }
              frame 31 {
                w4587 = T13 2 items=["User Home"=0, "User Desktop"=1, "User Documents"=2, "User Application Data"=3, "User Preferences"=4, "User Temporary"=5, "Public Documents"=6, "Public Application Data"=7, "Public Preferences"=8, "Public Cache"=13, "System Core Libraries"=9, "System Installed Libraries"=10, "Application Files"=11, "Boot Volume Root"=12] ("system directory type")
                n1811 = Search and Replace String(replace all?=TRUE ("replace all? (F)"), input string=w4582, search string="/") -> (result string=w4603:string)  [unwired: 5 in, 3 out]
                n1812 = Concatenate Strings(w4580, "TimeStamp;Measure Ch_Z(g);Ch_X(g);Ch_Y(g);INC_X(Deg);INC_Y(Deg)", "\n") -> (w4596:string)
                n1813 = Concatenate Strings(w4603, "_" ("string"), "S_E_T.csv") -> (w4604:string)
                n1814 = call <vilib>:"Get System Directory.vi"("system directory type"=w4587) -> ("system directory"=w4597:path)  [unwired: 10 in]
                n1815 = Build Path(base path=w4597, name or relative path="Logfile") -> (appended path=w4598:path)
                n1816 = call <vilib>:"Check if File or Folder Exists.vi"("path"=w4598) -> ("file or folder exists?"=w4599:bool, "dup path"=w4600:path)  [unwired: 8 in, 1 out]
                n1817 = case shown="False" w4599 {
                  tunnel: w4600 -> [w4625 w4626]
                  tunnel: [w4624 w4626] -> w4601
                  frame False {
                    n1818 = Create Folder(path (use dialog)=w4625) -> (created path=w4624:path)  [unwired: 2 in, 2 out]
                  }
                  frame True {
                  }
                }
                n1819 = Decimate 1D Array(w4622) -> (w4621:dbl[], w4620:dbl[], w4619:dbl[], w4618:dbl[], w4616:dbl[])
                n1820 = Build Path(base path=w4601, name or relative path=w4604) -> (appended path=w4602:path)
                n1821 = for {
                  tunnel: [w4652] -> w4615 mode=indexing
                  tunnel: w4617 -> [w4646] mode=indexing
                  tunnel: w4621 -> [w4641] mode=indexing
                  tunnel: w4620 -> [w4640] mode=indexing
                  tunnel: w4619 -> [w4639] mode=indexing
                  tunnel: w4618 -> [w4638] mode=indexing
                  tunnel: w4616 -> [w4637] mode=indexing
                  tunnel: [w4641] -> w4614 mode=indexing
                  tunnel: [w4640] -> w4613 mode=indexing
                  tunnel: [w4639] -> w4612 mode=indexing
                  tunnel: [w4638] -> w4611 mode=indexing
                  tunnel: [w4637] -> w4610 mode=indexing
                  tunnel: w4609 -> [w4631]
                  tunnel: w4608 -> [w4630]
                  tunnel: w4607 -> [w4629] mode=indexing
                  tunnel: w4606 -> [w4628]
                  tunnel: [w4627] -> w4605
                  n1822 = Join Numbers(hi=w4631, lo=w4630) -> ((hi.lo)=w4634:u32)
                  n1823 = To Double Precision Float(number=w4629) -> (double precision float=w4635:dbl)
                  n1824 = Number To Decimal String(number=w4646) -> (decimal integer string=w4651:string)  [unwired: 1 in]
                  n1825 = Number To Fractional String(number=w4641, precision (6)=i16 3 ("width (-)")) -> (F-format string=w4653:string)  [unwired: 2 in]
                  n1826 = Number To Fractional String(number=w4640, precision (6)=i16 3 ("width (-)")) -> (F-format string=w4649:string)  [unwired: 2 in]
                  n1827 = Number To Fractional String(number=w4639, precision (6)=i16 3 ("width (-)")) -> (F-format string=w4647:string)  [unwired: 2 in]
                  n1828 = Number To Fractional String(number=w4638, precision (6)=i16 3 ("width (-)")) -> (F-format string=w4644:string)  [unwired: 2 in]
                  n1829 = Number To Fractional String(number=w4637, precision (6)=i16 3 ("width (-)")) -> (F-format string=w4642:string)  [unwired: 2 in]
                  n1830 = Divide(x=w4635, y=w4628) -> (x/y=w4636:dbl)
                  n1831 = To Unsigned Quad Integer(1:w4634) -> (0:w4633:u64)
                  n1832 = Build Array(w4651, w4653, w4649, w4647, w4644, w4642) -> (w4652:string[])
                  n1833 = call "Unix Time to Timestamp.vi"("Fractional Second"=w4636, "Unix Time (s)"=w4633) -> ("Timestamp"=w4632:timestamp)  [unwired: 8 in, 1 out]
                  n1834 = To Double Precision Float(number=w4632) -> (double precision float=w4627:dbl)
                }
                n1835 = Open/Create/Replace File(file path (use dialog)=w4602, operation (0:open)=T10."open or create") -> (refnum out=w4595:refnum<file>, error out=w4593:errorcluster)  [unwired: 4 in, 1 out]
                n1836 = Write to Text File(file (use dialog)=w4595, text=w4596, error in=w4593) -> (refnum out=w4594:refnum<file>, error out=w4592:errorcluster)  [unwired: 1 in, 1 out]
                n1837 = Close File(refnum=w4594, error in=w4592) -> (path=w4581:path)  [unwired: 1 out]
              }
            }
            "Enabled channels" <- w2639
            "CH_Z Graph" <- w2561
            "CH_X Graph" <- w2559
            "CH_Y Graph" <- w2558
            "INC_X Graph" <- w2557
            "INC_Y Graph" <- w2556
            "File path" <- w2548
            n1838 = call-poly <vilib>:"Write Delimited Spreadsheet.vi"("file path (dialog if empty)"=w2548, "format (%s)"="%s", "2D data"=w2563, "append to file? (new file:F)"=TRUE, "transpose? (no:F)"=FALSE, "delimiter (\\t)"=";" ("delimiter (\\t)")) -> ()  [unwired: 8 in, 2 out]
            n1839 = property on="CH_Z Graph" class="WFChart (strict)"("XScale.Offset"=w2551) -> ()  [unwired: 2 in, 2 out]
            n1840 = property on="INC_Y Graph" class="WFChart (strict)"("XScale.Offset"=w2547) -> ()  [unwired: 2 in, 2 out]
            n1841 = property on="CH_X Graph" class="WFChart (strict)"("XScale.Offset"=w2501) -> ()  [unwired: 2 in, 2 out]
            n1842 = property on="INC_X Graph" class="WFChart (strict)"("XScale.Offset"=w2549) -> ()  [unwired: 2 in, 2 out]
            n1843 = property on="CH_Y Graph" class="WFChart (strict)"("XScale.Offset"=w2550) -> ()  [unwired: 2 in, 2 out]
          }
          frame 7 {
            w4692 = "NA"
            w4730 = T13 2 items=["User Home"=0, "User Desktop"=1, "User Documents"=2, "User Application Data"=3, "User Preferences"=4, "User Temporary"=5, "Public Documents"=6, "Public Application Data"=7, "Public Preferences"=8, "Public Cache"=13, "System Core Libraries"=9, "System Installed Libraries"=10, "Application Files"=11, "Boot Volume Root"=12] ("system directory type")
            # "function to write data in log file"
            # "this block conttain measures + dates of different  sensor channels"
            # "logfile path"
            # "logfile headers"
            # "this block contain Channels bitmap"
            n1844 = String To Byte Array(string=w4840) -> (unsigned byte array=w4773:u8[])
            n1845 = String Subset(string=w4683, offset (0)=0, length (rest)=16 ("length (rest)")) -> (substring=w4682:string)
            n1846 = Array To Cluster(array=w4773) -> (cluster=w4839:T16)
            n1847 = Array Size(array=w4773) -> (size(s)=w4775:i32)
            n1848 = property on="Measure Mode" class="Str"() -> ("Value"=w4657:string)  [unwired: 2 in, 2 out]
            n1849 = Unbundle(w4839) -> ("unsigned byte array[2]"=w4677:u8, "unsigned byte array[3]"=w4838:u8, "unsigned byte array[4]"=w4837:u8, "unsigned byte array[5]"=w4831:u8, "unsigned byte array[6]"=w4830:u8, "unsigned byte array[7]"=w4829:u8, "unsigned byte array[8]"=w4828:u8, "unsigned byte array[9]"=w4827:u8, "unsigned byte array[10]"=w4826:u8, "unsigned byte array[12]"=w4825:u8, "unsigned byte array[16]"=w4822:u8, "unsigned byte array[17]"=w4819:u8, "unsigned byte array[18]"=w4818:u8, "unsigned byte array[19]"=w4806:u8, "unsigned byte array[20]"=w4817:u8, "unsigned byte array[21]"=w4816:u8, "unsigned byte array[22]"=w4815:u8, "unsigned byte array[23]"=w4814:u8, "unsigned byte array[24]"=w4813:u8, "unsigned byte array[25]"=w4823:u8, "unsigned byte array[26]"=w4812:u8, "unsigned byte array[27]"=w4811:u8, "unsigned byte array[28]"=w4804:u8, "unsigned byte array[29]"=w4810:u8, "unsigned byte array[30]"=w4809:u8, "unsigned byte array[31]"=w4808:u8, "unsigned byte array[32]"=w4824:u8, "unsigned byte array[33]"=w4807:u8, "unsigned byte array[34]"=w4820:u8, "unsigned byte array[35]"=w4821:u8)  [unwired: 6 out]
            n1850 = Subtract(x=w4775, y=35) -> (x-y=w4774:i32)
            n1851 = Join Numbers(hi=w4830, lo=w4831) -> ((hi.lo)=w4835:u16)
            n1852 = Join Numbers(hi=w4837, lo=w4838) -> ((hi.lo)=w4836:u16)
            n1853 = Join Numbers(hi=w4827, lo=w4828) -> ((hi.lo)=w4833:u16)
            n1854 = Join Numbers(hi=w4826, lo=w4833) -> ((hi.lo)=w4832:u32)
            n1855 = Equal?(x=w4657, y="S_E_T") -> (x = y?=w4659:bool)
            n1856 = To Long Integer(number=w4832) -> (32bit integer=→"Acquisition duration":i32)
            n1857 = To Unsigned Byte Integer(number=w4825) -> (unsigned 8bit integer=w4681:u8)
            n1858 = Join Numbers(hi=w4812, lo=w4823) -> ((hi.lo)=w4803:u16)
            n1859 = Join Numbers(hi=w4807, lo=w4824) -> ((hi.lo)=w4799:u16)
            n1860 = Join Numbers(hi=w4819, lo=w4822) -> ((hi.lo)=w4805:u16)
            n1861 = Join Numbers(hi=w4821, lo=w4820) -> ((hi.lo)=w4668:u16)
            "Number of data per channel" <- w4668
            n1862 = Join Numbers(hi=w4829, lo=w4835) -> ((hi.lo)=w4834:u32)
            n1863 = To Word Integer(number=w4836) -> (16bit integer=w4669:i16)
            "Acquisition frequency" <- w4669
            n1864 = To Long Integer(number=w4834) -> (32bit integer=→"Acquisition cycle":i32)
            n1865 = Format Into String(format string="%d/%d/%d %d:%d:%d,%d", w4804, w4811, w4803, w4810, w4809, w4808, w4799) -> (resulting string=w4745:string)  [unwired: 2 in, 1 out]
            "End date" <- w4745
            n1866 = Join Numbers(hi=w4813, lo=w4814) -> ((hi.lo)=w4798:u16)
            n1867 = Array Subset(array=w4773, index=36, length=w4774) -> (w4671:u8[])
            n1868 = Format Into String(format string="%d/%d/%d %d:%d:%d,%d", w4806, w4818, w4805, w4817, w4816, w4815, w4798) -> (resulting string=w4670:string)  [unwired: 2 in, 1 out]
            "Start date" <- w4670
            n1869 = property on="concatenated string" class="Str"() -> ("Value"=w4656:string)  [unwired: 2 in, 2 out]
            n1870 = call <vilib>:"Get System Directory.vi"("system directory type"=w4730) -> ("system directory"=w4737:path)  [unwired: 10 in]
            n1871 = case shown="1001" w4681 {
              tunnel: ["" "no active channel" "chZ " "chX " "chZ & chX " "chY " "chZ & chY  " "chX & chY " "chZ& chX& chY " "INC_X " "chZ & INC_X " "chX & INC_X " "chZ& chX & INC_X " "chY & INC_X " "chZ  & chY & INC_X " "chX  & chY & INC_X " "chZ& chX  & chY & INC_X " "INC_Y  " " chZ & INC_Y " " chX & INC_Y  " "chZ & chX & INC_Y " " chY & INC_Y " "chZ & chY & INC_Y" "chX & chY & INC_Y" " chZ &chX & chY & INC_Y  " " INC_X & INC_Y " "chZ &   INC_X & INC_Y" "chX & INC_X & INC_Y" " chZ & chX &  INC_X & INC_Y  " " chY &  INC_X & INC_Y  " "chZ & chY &  INC_X & INC_Y " "chX & chY &  INC_X & INC_Y" "chZ & chX & chY &  INC_X & INC_Y"] -> w4680
              frame Default {
              }
              frame 0 {
              }
              frame 1 {
              }
              frame 2 {
              }
              frame 3 {
              }
              frame 4 {
              }
              frame 5 {
              }
              frame 6 {
              }
              frame 7 {
              }
              frame 8 {
              }
              frame 9 {
              }
              frame 10 {
              }
              frame 11 {
              }
              frame 12 {
              }
              frame 13 {
              }
              frame 14 {
              }
              frame 15 {
              }
              frame 16 {
              }
              frame 17 {
              }
              frame 18 {
              }
              frame 19 {
              }
              frame 20 {
              }
              frame 21 {
              }
              frame 22 {
              }
              frame 23 {
              }
              frame 24 {
              }
              frame 25 {
              }
              frame 26 {
              }
              frame 27 {
              }
              frame 28 {
              }
              frame 29 {
              }
              frame 30 {
              }
              frame 31 {
              }
            }
            "Enabled channels" <- w4680
            n1872 = case shown="7" w4677 {
              tunnel: ["" "LDCDA mode" "Alarm mode" "Streaming mode" "S.E.T mode " "Dynamic mode"] -> w4676
              frame Default {
              }
              frame 1 {
              }
              frame 2 {
              }
              frame 3 {
              }
              frame 6 {
              }
              frame 7 {
              }
            }
            "Acquisition Mode" <- w4676
            n1873 = Select(t=w4657, s=w4659, f=w4656) -> (s? t:f=w4655:string)
            n1874 = Build Path(base path=w4737, name or relative path="Logfile") -> (appended path=w4738:path)
            n1875 = call <vilib>:"Check if File or Folder Exists.vi"("path"=w4738) -> ("file or folder exists?"=w4739:bool, "dup path"=w4740:path)  [unwired: 8 in, 1 out]
            n1876 = case shown="False" w4739 {
              tunnel: w4740 -> [w4885 w4886]
              tunnel: [w4884 w4886] -> w4741
              frame False {
                n1877 = Create Folder(path (use dialog)=w4885) -> (created path=w4884:path)  [unwired: 2 in, 2 out]
              }
              frame True {
              }
            }
            n1878 = Concatenate Strings(w4682, "_" ("string"), w4655, "_" ("string"), "Transmit_Math_Mode.txt") -> (w4743:string)
            n1879 = Decimate 1D Array(w4671) -> (w4797:u8[], w4796:u8[], w4795:u8[], w4794:u8[], w4793:u8[], w4792:u8[], w4791:u8[], w4790:u8[], w4789:u8[], w4788:u8[], w4787:u8[], w4786:u8[], w4785:u8[], w4784:u8[], w4783:u8[], w4782:u8[], w4781:u8[], w4780:u8[], w4779:u8[], w4778:u8[], w4777:u8[])
            n1880 = Concatenate Strings(w4670, ";", w4745) -> (w4748:string)
            n1881 = Build Path(base path=w4741, name or relative path=w4743) -> (appended path=w4742:path)
            n1882 = for {
              tunnel: w4668 -> [w4914]
              tunnel: w4797 -> [w4949] mode=indexing
              tunnel: w4796 -> [w4948] mode=indexing
              tunnel: w4795 -> [w4947] mode=indexing
              tunnel: w4794 -> [w4946] mode=indexing
              tunnel: w4793 -> [w4945] mode=indexing
              tunnel: w4792 -> [w4944] mode=indexing
              tunnel: w4791 -> [w4943] mode=indexing
              tunnel: w4790 -> [w4942] mode=indexing
              tunnel: w4789 -> [w4904] mode=indexing
              tunnel: w4788 -> [w4941] mode=indexing
              tunnel: w4787 -> [w4940] mode=indexing
              tunnel: w4786 -> [w4939] mode=indexing
              tunnel: w4785 -> [w4938] mode=indexing
              tunnel: w4784 -> [w4937] mode=indexing
              tunnel: w4783 -> [w4936] mode=indexing
              tunnel: w4782 -> [w4935] mode=indexing
              tunnel: w4781 -> [w4934] mode=indexing
              tunnel: w4780 -> [w4902] mode=indexing
              tunnel: w4779 -> [w4933] mode=indexing
              tunnel: w4778 -> [w4932] mode=indexing
              tunnel: w4777 -> [w4903] mode=indexing
              tunnel: [w4890] -> w4761 mode=indexing
              tunnel: [w4931] -> w4762 mode=indexing
              tunnel: [w4891] -> w4770 mode=indexing
              tunnel: w4669 -> [w4921]
              tunnel: w4670 -> [w4917]
              tunnel: w4669 -> [w4916]
              tunnel: [w4892] -> w4768 mode=indexing
              tunnel: [w4896] -> w4765 mode=indexing
              n1883 = Sign(1:w4903) -> (0:w4956:u8)
              n1884 = Scan From String(format string="%<%d/%m/%Y %H:%M:%S%3u>T", input string=w4917) -> (output 1=w4923:timestamp)  [unwired: 3 in, 3 out]
              n1885 = Join Numbers(hi=w4948, lo=w4949) -> ((hi.lo)=w4962:u16)
              n1886 = Join Numbers(hi=w4946, lo=w4947) -> ((hi.lo)=w4961:u16)
              n1887 = Join Numbers(hi=w4940, lo=w4941) -> ((hi.lo)=w4959:u16)
              n1888 = Join Numbers(hi=w4938, lo=w4939) -> ((hi.lo)=w4958:u16)
              n1889 = Join Numbers(hi=w4934, lo=w4935) -> ((hi.lo)=w4908:u16)
              n1890 = Join Numbers(hi=w4932, lo=w4933) -> ((hi.lo)=w4957:u16)
              n1891 = To Byte Integer(number=w4943) -> (8bit integer=w4901:i8)
              n1892 = To Byte Integer(number=w4942) -> (8bit integer=w4900:i8)
              n1893 = Sign(1:w4904) -> (0:w4960:u8)
              n1894 = Sign(1:w4902) -> (0:w4907:u8)
              n1895 = Join Numbers(hi=w4944, lo=w4945) -> ((hi.lo)=w4954:u16)
              "index minval" <- w4954
              n1896 = Join Numbers(hi=w4936, lo=w4937) -> ((hi.lo)=w4950:u16)
              "index maxval" <- w4950
              n1897 = To Byte Integer(number=w4956) -> (8bit integer=w4911:i8)
              n1898 = Join Numbers(hi=w4900, lo=w4901) -> ((hi.lo)=w4913:u16)
              n1899 = Join Numbers(hi=w4961, lo=w4962) -> ((hi.lo)=w4955:u32)
              "fid min ch1" <- w4955
              n1900 = Join Numbers(hi=w4958, lo=w4959) -> ((hi.lo)=w4951:u32)
              "fid max ch1" <- w4951
              n1901 = To Word Integer(number=w4908) -> (16bit integer=w4909:i16)
              n1902 = To Byte Integer(number=w4907) -> (8bit integer=w4905:i8)
              n1903 = To Word Integer(number=w4957) -> (16bit integer=w4910:i16)
              n1904 = case shown="1" w4905 {
                tunnel: w4909 -> [_ w4971 w4977]
                tunnel: [_ w4969 w4976] -> w4890
                frame Default {
                }
                frame 1 {
                  n1905 = Equal?(x=w4971, y=i16 0) -> (x = y?=w4973:bool)
                  n1906 = Divide(x=w4971, y=-1000.0) -> (x/y=w4970:dbl)
                  n1907 = Select(t=0.0 ("f"), s=w4973, f=w4970) -> (s? t:f=w4969:dbl)
                }
                frame 0 {
                  n1908 = Equal?(x=w4977, y=i16 -1) -> (x = y?=w4980:bool)
                  n1909 = Divide(x=w4977, y=1000.0) -> (x/y=w4978:dbl)
                  n1910 = Select(t=0.0 ("f"), s=w4980, f=w4978) -> (s? t:f=w4976:dbl)
                }
              }
              n1911 = case shown="0" w4911 {
                tunnel: [_ w4964 w4967] -> w4931
                tunnel: w4910 -> [_ w4963 w4966]
                frame Default {
                }
                frame 1 {
                  n1912 = Divide(x=w4963, y=-1000.0) -> (x/y=w4964:dbl)
                }
                frame 0 {
                  n1913 = Divide(x=w4966, y=1000.0) -> (x/y=w4967:dbl)
                }
              }
              n1914 = Multiply(x=w4914, y=w4955) -> (x*y=w4953:u32)
              n1915 = Multiply(x=w4914, y=w4951) -> (x*y=w4952:u32)
              n1916 = To Word Integer(number=w4913) -> (16bit integer=w4912:i16)
              n1917 = To Byte Integer(number=w4960) -> (8bit integer=w4906:i8)
              n1918 = case shown="0" w4906 {
                tunnel: w4912 -> [_ w4988 w4993]
                tunnel: [_ w4985 w4992] -> w4891
                frame Default {
                }
                frame 1 {
                  n1919 = Equal?(x=w4988, y=i16 -1) -> (x = y?=w4986:bool)
                  n1920 = Divide(x=w4988, y=-1000.0) -> (x/y=w4983:dbl)
                  n1921 = Select(t=0.0 ("f"), s=w4986, f=w4983) -> (s? t:f=w4985:dbl)
                }
                frame 0 {
                  n1922 = Equal?(x=w4993, y=i16 -1) -> (x = y?=w4994:bool)
                  n1923 = Divide(x=w4993, y=1000.0) -> (x/y=w4990:dbl)
                  n1924 = Select(t=0.0 ("f"), s=w4994, f=w4990) -> (s? t:f=w4992:dbl)
                }
              }
              n1925 = Add(x=w4954, y=w4953) -> (x+y=w4919:u32)
              n1926 = Add(x=w4950, y=w4952) -> (x+y=w4922:u32)
              n1927 = Divide(x=1, y=w4916) -> (x/y=w4925:dbl)
              n1928 = Divide(x=1, y=w4921) -> (x/y=w4928:dbl)
              n1929 = Multiply(x=w4925, y=w4919) -> (x*y=w4926:dbl)
              n1930 = Multiply(x=w4928, y=w4922) -> (x*y=w4929:dbl)
              n1931 = call "Timestamp to Unix Time.vi"("Timestamp (now)"=w4923) -> ("Unix Time (s)"=w4930:i64)  [unwired: 9 in, 1 out]
              n1932 = Add(x=w4930, y=w4926) -> (x+y=w4924:dbl)
              n1933 = Add(x=w4930, y=w4929) -> (x+y=w4927:dbl)
              n1934 = call "Unix Time to Timestamp.vi"("Unix Time (s)"=w4924) -> ("Timestamp"=w4899:timestamp)  [unwired: 9 in, 1 out]
              n1935 = Equal To 0?(x=w4890) -> (x = 0?=w4888:bool)
              n1936 = call "Unix Time to Timestamp.vi"("Unix Time (s)"=w4927) -> ("Timestamp"=w4893:timestamp)  [unwired: 9 in, 1 out]
              n1937 = Equal To 0?(x=w4891) -> (x = 0?=w4889:bool)
              n1938 = Format Date/Time String(seconds (now)=w4899) -> (date/time string=w4897:string)  [unwired: 2 in]
              n1939 = Format Date/Time String(seconds (now)=w4893) -> (date/time string=w4894:string)  [unwired: 2 in]
              n1940 = And(x=w4889, y=w4888) -> (x .and. y?=w4887:bool)
              n1941 = Select(t="NA", s=w4887, f=w4897) -> (s? t:f=w4896:string)
              n1942 = Select(t="NA", s=w4887, f=w4894) -> (s? t:f=w4892:string)
            }
            "Max value" <- w4761
            "Average value" <- w4762
            "Min value" <- w4770
            "Min date" <- w4765
            "Max date" <- w4768
            n1943 = Open/Create/Replace File(file path (use dialog)=w4742, operation (0:open)=T10."open or create") -> (refnum out=w4735:refnum<file>, error out=w4733:errorcluster)  [unwired: 4 in, 1 out]
            n1944 = Concatenate Strings("Start Date;End Date;Ch_Z_Min value date;Ch_Z_Min value;Ch_Z_Max value date;Ch_Z_Max value;Ch_Z_Average value;Ch_X_Min value date;Ch_X_Min value;Ch_X_Max value date;Ch_X_Max value;Ch_X_Average value;Ch_Y_Min value date;Ch_Y_Min value;Ch_Y_Max value date;Ch_Y_Max value;Ch_Y_Average value;INC_X_Min value date;INC_X_Min value_Deg;INC_X_Max value date;INC_X_Max value_Deg;INC_X_Average value_Deg;INC_Y_Min value date\t;INC_Y_Min value_Deg;INC_Y_Max value date;INC_Y_Max value_Deg;INC_Y_Average value\t", "\n") -> (w4736:string)
            n1945 = Write to Text File(file (use dialog)=w4735, text=w4736, error in=w4733) -> (refnum out=w4734:refnum<file>, error out=w4732:errorcluster)  [unwired: 1 in, 1 out]
            n1946 = Close File(refnum=w4734, error in=w4732) -> (path=w4726:path)  [unwired: 1 out]
            "File path" <- w4726
            n1947 = Equal?(x=w4721, y=u8 1) -> (x = y?=w4672:bool)
            n1948 = Equal?(x=w4721, y=u8 6) -> (x = y?=w4722:bool)
            n1949 = Not Or(1:w4722, 2:w4672) -> (0:w4705:bool)
            n1950 = Array To Cluster(array=w4765) -> (cluster=w4766:T17)
            n1951 = Array To Cluster(array=w4768) -> (cluster=w4767:T17)
            n1952 = Array To Cluster(array=w4770) -> (cluster=w4769:T18)
            n1953 = Array To Cluster(array=w4761) -> (cluster=w4764:T18)
            n1954 = Array To Cluster(array=w4762) -> (cluster=w4763:T18)
            n1955 = Unbundle(w4766) -> ("[0]"=w4667:string, "[1]"=w4757:string, "[2]"=w4754:string, "[3]"=w4665:string, "[4]"=w4664:string)
            n1956 = Unbundle(w4767) -> ("[0]"=w4760:string, "[1]"=w4756:string, "[2]"=w4715:string, "[3]"=w4663:string, "[4]"=w4662:string)
            n1957 = Unbundle(w4769) -> ("[0]"=w4666:dbl, "[1]"=w4675:dbl, "[2]"=w4753:dbl, "[3]"=w4711:dbl, "[4]"=w4710:dbl)
            n1958 = Unbundle(w4764) -> ("[0]"=w4759:dbl, "[1]"=w4752:dbl, "[2]"=w4751:dbl, "[3]"=w4709:dbl, "[4]"=w4708:dbl)
            n1959 = Unbundle(w4763) -> ("[0]"=w4758:dbl, "[1]"=w4755:dbl, "[2]"=w4750:dbl, "[3]"=w4707:dbl, "[4]"=w4706:dbl)
            n1960 = Number To Fractional String(number=w4711, precision (6)=i16 3 ("width (-)")) -> (F-format string=w4704:string)  [unwired: 2 in]
            n1961 = Number To Fractional String(number=w4709, precision (6)=i16 3 ("width (-)")) -> (F-format string=w4702:string)  [unwired: 2 in]
            n1962 = Number To Fractional String(number=w4707, precision (6)=i16 3 ("width (-)")) -> (F-format string=w4700:string)  [unwired: 2 in]
            n1963 = Number To Fractional String(number=w4710, precision (6)=i16 3 ("width (-)")) -> (F-format string=w4703:string)  [unwired: 2 in]
            n1964 = Number To Fractional String(number=w4708, precision (6)=i16 3 ("width (-)")) -> (F-format string=w4701:string)  [unwired: 2 in]
            n1965 = Number To Fractional String(number=w4706, precision (6)=i16 3 ("width (-)")) -> (F-format string=w4699:string)  [unwired: 2 in]
            n1966 = Select(t=w4665, s=w4705, f="NA") -> (s? t:f=w4717:string)
            n1967 = Select(t=w4663, s=w4705, f="NA") -> (s? t:f=w4716:string)
            n1968 = Select(t=w4704, s=w4705, f=w4692) -> (s? t:f=w4698:string)
            n1969 = Select(t=w4702, s=w4705, f=w4692) -> (s? t:f=w4696:string)
            n1970 = Select(t=w4700, s=w4705, f=w4692) -> (s? t:f=w4693:string)
            n1971 = Select(t=w4703, s=w4705, f=w4692) -> (s? t:f=w4697:string)
            n1972 = Select(t=w4701, s=w4705, f=w4692) -> (s? t:f=w4695:string)
            n1973 = Select(t=w4699, s=w4705, f=w4692) -> (s? t:f=w4694:string)
            n1974 = Select(t=w4664, s=w4705, f="") -> (s? t:f=w4714:string)
            n1975 = Select(t=w4662, s=w4705, f="") -> (s? t:f=w4718:string)
            n1976 = Format Into String(format string=";%S ;%.3f;%s;%.3f;%.3f;%S;%.3f;%s;%.3f;%.3f;%S ;%.3f ;%s;%.3f; %.3f ;%s ;%s; %s ;%s ;%s; %s ;%s ;%s ;%s ;%s\\n", initial string=w4748, w4667, w4666, w4760, w4759, w4758, w4757, w4675, w4756, w4752, w4755, w4754, w4753, w4715, w4751, w4750, w4717, w4698, w4716, w4696, w4693, w4714, w4697, w4718, w4695, w4694) -> (resulting string=w4747:string)  [unwired: 1 in, 1 out]
            n1977 = Build Array(w4747) -> (w4746:string[])
            n1978 = call-poly <vilib>:"Write Delimited Spreadsheet.vi"("file path (dialog if empty)"=w4726, "1D data"=w4746, "append to file? (new file:F)"=TRUE, "transpose? (no:F)"=TRUE, "delimiter (\\t)"=";" ("delimiter (\\t)")) -> ()  [unwired: 9 in, 2 out]
            "Device type" <- w4841
            "String" <- "Ch_Z                    Ch_X                     Ch_Y                     INC_X                     INC_Y" ("String")
          }
        }
        "Measure Mode" <- w70
        "Date & time" <- w65
        "Sensor Label" <- w68
        "Device type" <- w69
        "Date & time" <- w65
        "Sensor Label" <- w68
        "Measure Mode" <- w70
        "Measure" <- w55
        "Measure" <- w55
        "Numeric" <- w50
      }
    }
  }
  n1979 = Unregister For Events(event registration refnum=w7, error in=w9) -> (error out=w8:errorcluster)
  n1980 = call "api_mqttDisconnect.vi"("error in (no error)"=w8) -> ("error out"=w14:errorcluster)  [unwired: 13 in, 1 out]
  n1981 = call "mqttTXdataQueue.vi"("function"=mqttTXdataQueueFunction."deinit", "error in (no error)"=w14) -> ("error out"=w10:errorcluster)  [unwired: 12 in, 1 out]
  n1982 = call "mqttRXsubscriptionEvent.vi"("function"=mqttRXsubscriptionEventFunction."deinit", "error in (no error)"=w10) -> ()  [unwired: 12 in, 2 out]
